vi "LifeEye_ver18_32bit.vi"() -> ()   [LabVIEW 2014]
uses:
  Keithley 2600 Series/sync_global.vi
  32bitDLLs/MADLib.dll
  LaserLineTunableFIlter/PHySpec-SDK-1.0.0/Labview-example/libPhyspec/libPhyspec.lvlib
panel:
  out "FilterWheelTemp":i32
  in  "Interline Delay (s)":dbl
  in  "2D Hyperspectral":bool
  out "Mono Calibration Handle":u32 caption="Calibration Handle"
  out "OMA V error":errorcluster
  in  "Tab Control 2":T1(tab)
  out "XY Graph OMA V":T2(graph)
  out "OMA V Hyperspectral graph":dbl[][](graph)
  out "OMA V PLE map graph":dbl[][](graph)
  out "OMA V PL external  sync plot":dbl[][](graph)
  out "timeend":i64
  out "timestart":i64
  out "Real Delay (seconds/step)":dbl
  out "Mono handle":u32
  in  "Grating Number":i16(ring) items=["", "Mirror", "300g/mm, blz=1.2um", "150g/mm, blz=1.2um"]
  in  "Filter Wheel Position":u16(ring) items=["", "Open", "320 nm", "590 nm", "715 nm", "655  nm", "Closed"]
  in  "Number of Spectra":i16=2 min=2 step=1
  out "Detector control":T3(tab)
  out "OMA V ready for sync":bool caption="ready"
  in  "OMA V correct background":bool
  in  "OMA V start background":bool
  in  "OMA V set temp":i8 caption="Set temp" min=-125 max=25 step=1
  in  "OMA V get temp":bool
  in  "OMA V start Focus":bool
  in  "OMA V Start Aquire":bool caption="Aquire"
  in  "OMA V gain":u32(ring) caption="Gain" items=["low", "high"]
  out "OMA V temp":dbl(slide) caption="Sensor Temperature" scale=-125.0..25.0
  in  "OMA V exposure time":dbl=0.001 caption="Integration time (s)" min=0.001 max=1000.0 step=0.001
  out "OMA  V ON":bool
  in  "Init OMA  V":bool
  in  "OMA V aquire mode":T4(radio) caption="Aquire mode"
  out "OMAV external sync":bool caption="sync"
  out "OMA V acquire from external":bool caption="acquire"
  out "OMA V Handles Out":T5
  out "OMA V Calibrated Array":dbl[](array[numeric]) caption="Calibrated Array" format="%.2f"
  out "Adjusted Values":T6 {"Pixel Width (microns)" format="%.2f"; "Magnification" format="%.2f"; "Detector Angle (degrees)" format="%.2f"; "Inclusion Angle (degrees)" format="%.2f"; "Focal Length (mm)" format="%.2f"; "Slope Adjust" format="%.2f"; "Center Offset" format="%.2f"}
  in  "Get param":bool
  in  "Init LockIn":bool
  out "LockIn ON":bool
  in  "Input Connection (0: Single-Ended Voltage)":u16(ring) items=["Single-Ended Voltage", "Differential Voltage", "1 MOhm Current Gain", "100 MOhm Current Gain"]
  in  "Input Coupling (0: AC)":u16(ring) items=["AC", "DC"]
  in  "Dynamic Reserve (2: Low Noise)":i8(ring)=2 items=["High Reserve"=0, "Normal"=1, "Low Noise"=2, "Auto Reserve"=-1]
  in  "Sensitivity (26: 1 V/uA)":i8(ring)=26 items=["Auto Gain"=-1, "2 nV/fA"=0, "5 nV/fA"=1, "10 nV/fA"=2, "20 nV/fA"=3, "50 nV/fA"=4, "100 nV/fA"=5, "200 nV/fA"=6, "500 nV/fA"=7, "1 uV/pA"=8, "2 uV/pA"=9, "5 uV/pA"=10, "10 uV/pA"=11, "20 uV/pA"=12, "50 uV/pA"=13, "100 uV/pA"=14, "200 uV/pA"=15, "500 uV/pA"=16, "1 mV/nA"=17, "2 mV/nA"=18, "5 mV/nA"=19, "10 mV/nA"=20, "20 mV/nA"=21, "50 mV/nA"=22, "100 mV/nA"=23, "200 mV/nA"=24, "500 mV/mA"=25, "1 V/uA"=26]
  in  "VISA resource name":refnum<visa-resource-name>
  out "LockIn Value":dbl
  in  "Histro start":bool
  in  "Histogramming Time (s)":dbl=0.001 min=0.001 max=360000.0 step=0.001
  in  "SaveHistro":bool
  in  "Init PicoHarp":bool
  out "PicoHarp ON":bool
  in  "Apply PicoHarp Settings":bool
  out "Error":bool
  out "Resolution":i32 min=0 max=2000 step=1
  out "SyncRate":i32 format="%#_7f"
  out "Ch1Rate":i32
  in  "Shutter:":bool
  in  "Bandpass (nm)":dbl min=0.0 max=30.0 step=0.1
  in  "ExcitationMap start":bool caption="OK Button"
  in  "PL Map Start":bool
  in  "Configuration File":path
  out "Current System":string
  out "LLTF error":errorcluster
  in  "PLE Start":bool
  out "LLTF handle":u32
  in  "Init LLTF":bool
  out "LLTF ON":bool
  in  "Wavelength LLTF (nm)":dbl=400.0 caption="Wavelength (nm)" min=400.0 max=1000.0 step=0.1
  in  "Tab Control":enum32{"Excitation", "Detection"}(tab)
  in  "Step delay LLTF":dbl caption="Step Delay (s)"
  in  "Steps LLTF":i32=1 caption="Steps" min=1 max=1000 step=1
  in  "End Wavelength LLTF":dbl=400.0 caption="End Wavelength (nm)" min=400.0 max=990.0 step=0.1
  in  "Start Wavelength LLTF":dbl=400.0 caption="Start Wavelength (nm)" min=400.0 max=1000.0 step=0.1
  in  "StepsDet":i32=1 caption="Steps" min=1 max=1000 step=1
  in  "Start Wavelength (nm)":dbl=400.0 min=400.0 max=2000.0 step=0.1
  in  "End Wavelength (nm)":dbl=400.0 min=400.0 max=2000.0 step=0.1
  in  "Step Delay (s)":dbl=0.1 min=0.001 max=360000.0 step=0.001
  in  "StepW (nm)":dbl=0.1 min=0.1 max=100.0 step=0.1
  in  "Forwardpix_scan":bool
  in  "Bidirectional scan":bool caption="Bidirectional"
  in  "PL_Clock":bool
  in  "SpectrMap start":bool
  in  "Stop Measurement":bool
  in  "ZScan start":bool
  out "MonoError":errorcluster
  out "PicoHarpInitError":bool
  out "PicoHarpHandle":i32
  out "Piezohandle":i32 caption="handle"
  in  "SaveIntMap":bool
  in  "SaveTRES":bool
  in  "SavePL":bool
  in  "IntMapping start":bool
  in  "StepZ (µm)":dbl=0.001 min=0.001 max=200.0 step=0.001
  in  "StepY (µm)":dbl=0.001 min=0.001 max=200.0 step=0.001
  in  "StepX (µm)":dbl=0.001 min=0.001 max=200.0 step=0.001
  in  "Pixel Delay (s)":dbl=0.1 min=0.001 max=360000.0 step=0.001
  in  "EndZ (µm)":dbl min=0.0 max=200.0 step=0.001
  in  "StartZ (µm)":dbl min=0.0 max=200.0 step=0.001
  in  "EndY (µm)":dbl min=0.0 max=200.0 step=0.001
  in  "StartY (µm)":dbl min=0.0 max=200.0 step=0.001
  in  "EndX (µm)":dbl min=0.0 max=200.0 step=0.001
  in  "StartX (µm)":dbl min=0.0 max=200.0 step=0.001
  in  "Stability check":bool
  in  "PL start":bool
  out "xRead":dbl format="%#.3g"
  out "yRead":dbl format="%#.3g"
  out "zRead":dbl format="%#.3g"
  in  "zCommand":dbl min=0.0 max=200.0 step=0.001
  in  "yCommand":dbl min=0.0 max=200.0 step=0.001
  in  "xCommand":dbl min=0.0 max=200.0 step=0.001
  in  "zGo":bool
  in  "yGo":bool
  in  "xGo":bool
  out "Busy":bool
  in  "Output Slit (µm)":i32=10 min=10 max=5000 step=1
  in  "Input Slit (µm)":i32=10 min=10 max=5000 step=1
  in  "Output Port":bool
  in  "Wavelength (nm)":dbl=400.0 min=-2000.0 max=2000.0 step=0.1
  out "PiezoStage ON":bool
  in  "Init Piezo":bool
  in  "Exit":bool
  out "Mono ON":bool
  in  "Init Mono":bool
  # "(only PLE Map)"
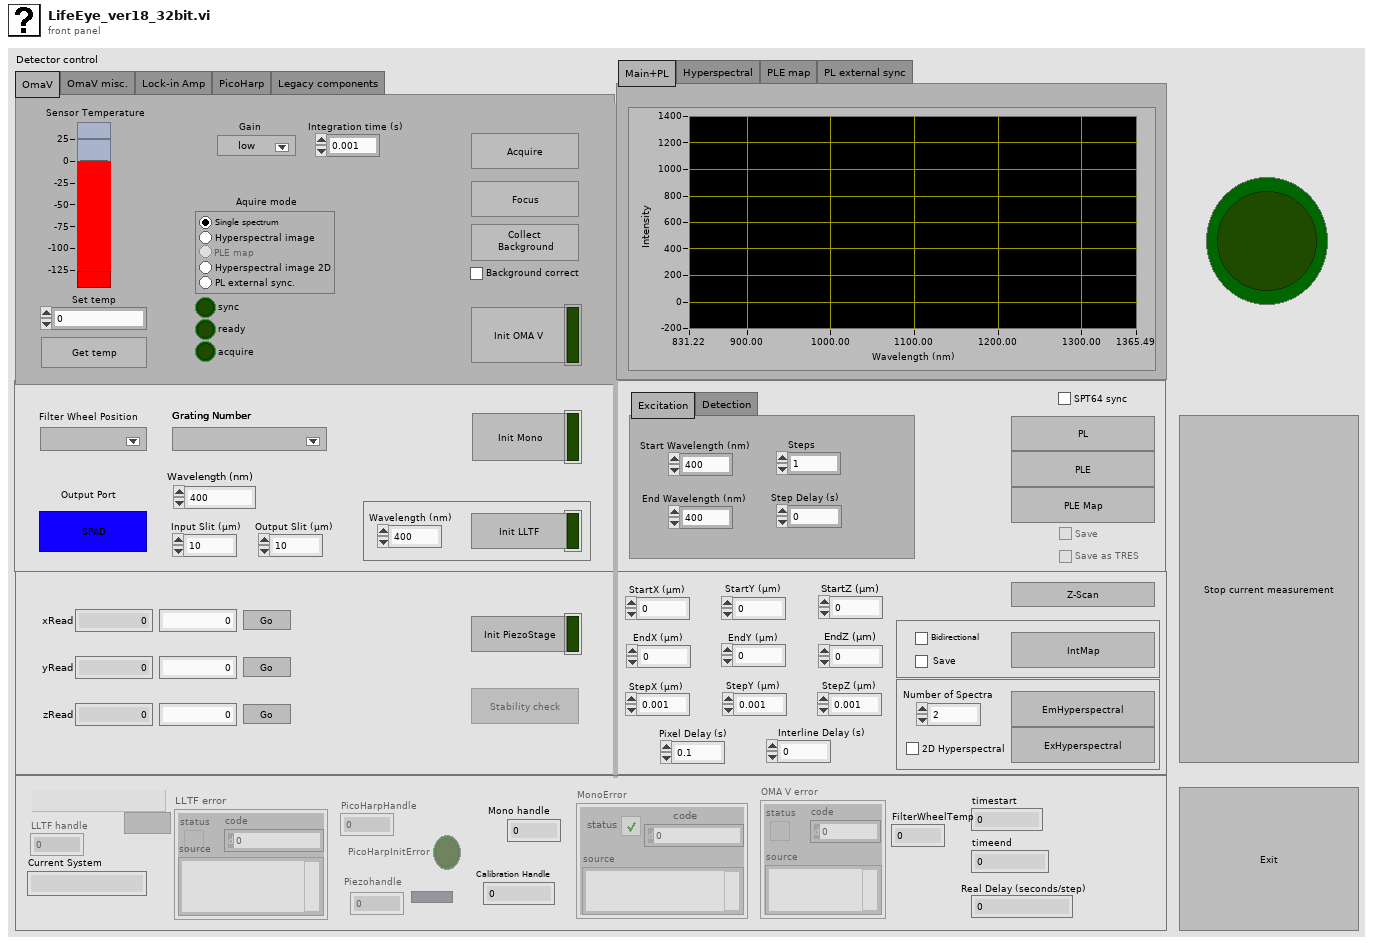
[diagram p1: front panel]
types:
  T1 = enum32{"Main+PL", "Hyperspectral", "PLE map", "PL external sync"}
  T2 = cluster{"Calibrated Array":dbl[], "Array F32":sgl[]}
  T3 = enum32{"OmaV", "OmaV misc.", "Lock-in Amp", "PicoHarp", "Legacy components"}
  T4 = enum32{"OMA V mode Single spectrum", "OMA V mode Hyperspectral", "OMA V mode PLE map", "OMA V mode Hyperspectral 2D", "OMA V mode PL external sync"}
  T5 = cluster{"Camera Handle":u32, "Pulser Handle":u32, "File Handle":u32, "Display Handle":u32, "Image Handle":u32}
  T6 = cluster{"Center Offset":dbl, "Slope Adjust":dbl, "Focal Length (mm)":dbl, "Inclusion Angle (degrees)":dbl, "Detector Angle (degrees)":dbl, "Magnification":dbl, "Pixel Width (microns)":dbl}
  T7 = enum8{"Enabled", "Disabled", "Disabled and Grayed Out"}
  T8 = cluster{"Acquire / focus mode \n1 is Sync circualar buffers":i32, "OMA V exposure time":dbl, "Number of Images":i32, "Number of software\naccumulations":i32}
  T9 = cluster{"Value From Calibration":dbl, "Value From Calibration":dbl, "Value From Calibration":dbl, "Value From Calibration":dbl, "Value From Calibration":dbl, "Value From Calibration":dbl, "Value From Calibration":dbl}
  T10 = cluster{"OMA V Calibrated Array":dbl[], "Array F32":sgl[]}
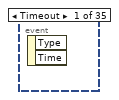
[diagram p2: hidden frame]
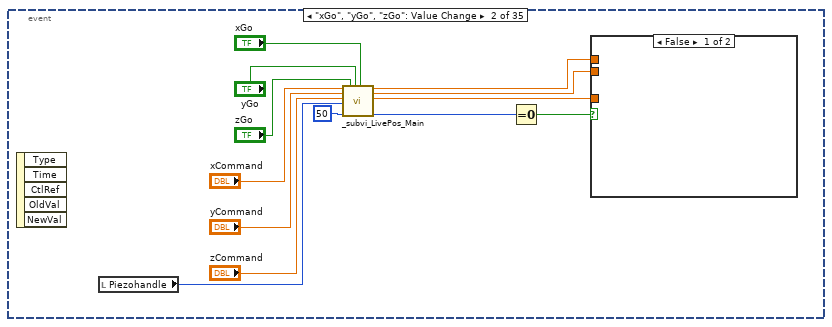
[diagram p3: hidden frame]
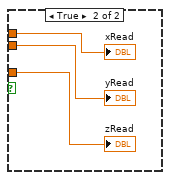
[diagram p4: hidden frame]
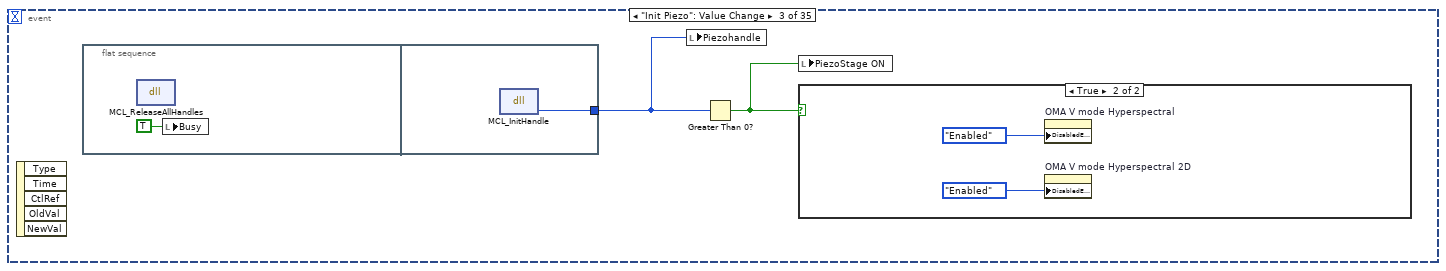
[diagram p5: hidden frame]
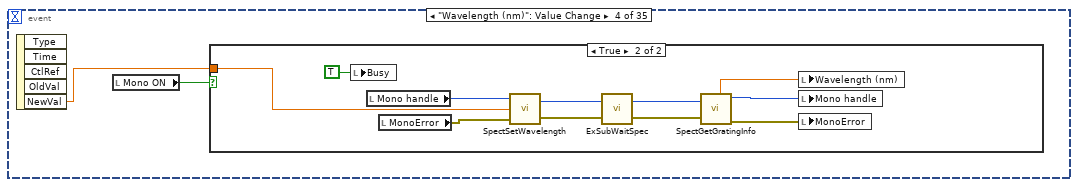
[diagram p7: hidden frame]
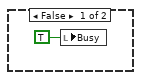
[diagram p8: hidden frame]
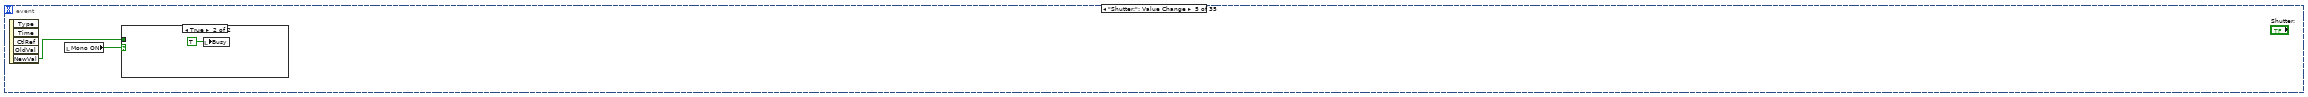
[diagram p9: hidden frame]
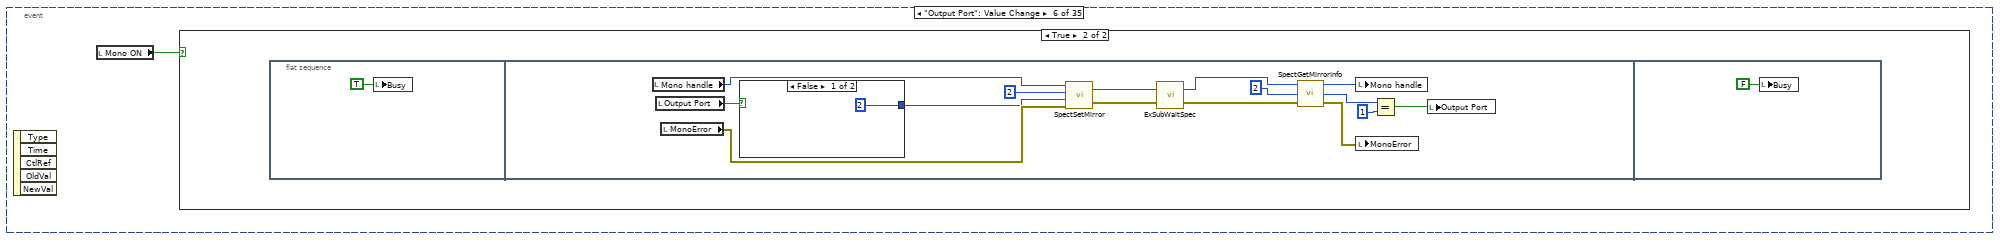
[diagram p11: hidden frame]
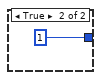
[diagram p13: hidden frame]
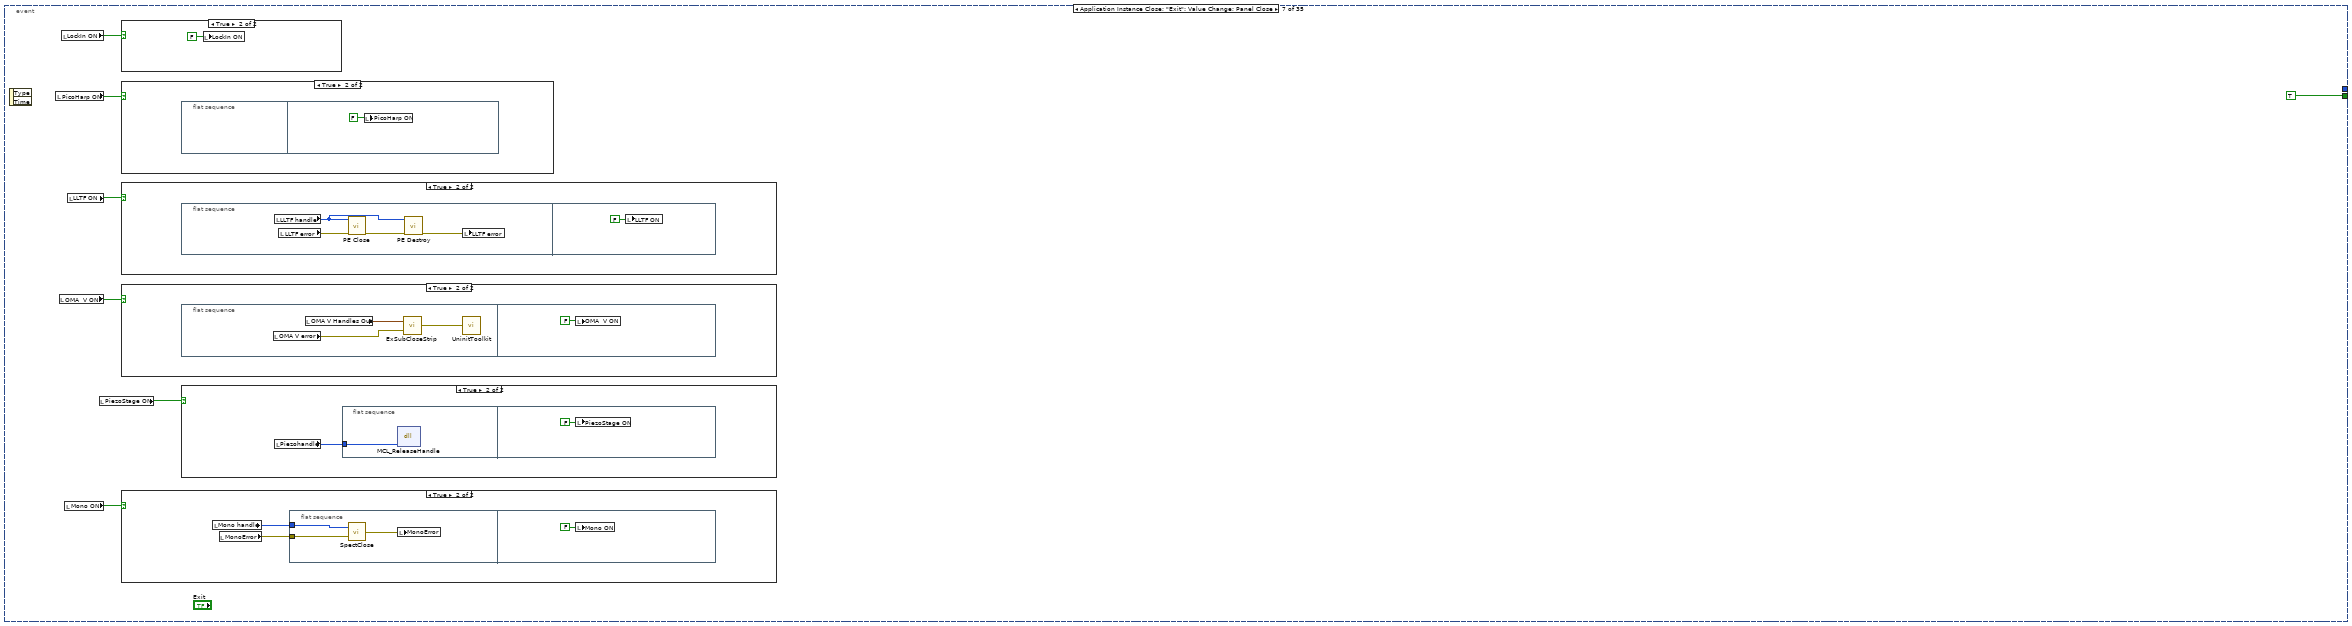
[diagram p14: hidden frame]
diagram:
  w4 = T7."Disabled and Grayed Out" ("Disabled")
  w14 = u16 1 items=["", "Mirror", "150g/mm, blz=1.2um", "300g/mm, blz=1.2um"] ("Grating Number")
  w15 = u16 1 items=["", "Open", "320 nm", "590 nm", "655 nm", "715  nm", "Closed"] ("Filter Wheel Position")
  w17 = FALSE
  w8 = FALSE
  # "PicoHarpResolution"
  # "PicoHarpSettingsError"
  # "PicoHarpInitError"
  # "PicoHarpHandle"
  # "MonoHandle"
  # "MonoError"
  # "PiezoHandle"
  # "error"
  n1 = while {
    stop <- w23 stop-if-true
    # "General seq."
    n2 = stacked-sequence {
      seq-local: [w26 _ _] -> [_ w461 _]
      seq-local: [w24 _ _] -> [_ w460 _]
      seq-local: [_ w461 _] -> [_ _ w2112]
      tunnel: [_ _ w2112] -> w23
      frame #0 {
        n3 = event shown="[19] \"Init LLTF\": Value Change" {
          selector: _ -> [_ _ _ _ _ _ _ _ _ _ _ _ _ _ _ _ _ _ _ _ _ _ _ _ _ _ _ _ _ _ _ _ _ _ _]
          dyn-events: _ -> [_ _ _ _ _ _ _ _ _ _ _ _ _ _ _ _ _ _ _ _ _ _ _ _ _ _ _ _ _ _ _ _ _ _ _]
          timeout: 1000 -> [_ _ _ _ _ _ _ _ _ _ _ _ _ _ _ _ _ _ _ _ _ _ _ _ _ _ _ _ _ _ _ _ _ _ _]
          tunnel: [_ _ _ _ _ _ TRUE _ _ _ _ _ _ _ _ _ _ _ _ _ _ _ _ _ _ _ _ _ _ _ _ _ _ _ _] -> w26
          tunnel: [_ _ _ _ _ _ _ _ _ _ _ _ _ w192 w195 w198 w201 w204 _ _ _ w247 w253 w257 _ _ _ w400 _ _ _ _ w438 w441 _] -> w24
          event Timeout {
            n4 = event-data() -> ()  [unwired: 1 in, 2 out]
          }
          event "xGo", "yGo", "zGo": Value Change {
            n5 = event-data() -> ()  [unwired: 1 in, 5 out]
            n6 = local read "Piezohandle"() -> (w27:i32)
            n7 = call "_subvi_LivePos_Main.vi"("xCommand"="xCommand", "yCommand"="yCommand", "zCommand"="zCommand", "handle"=w27, "counter"=u32 50, "commandZ"="zGo", "commandY"="yGo", "commandX"="xGo") -> ("xRead"=w39:dbl, "yRead"=w38:dbl, "zRead"=w37:dbl, "counter"=w32:u32)  [unwired: 8 out]
            n8 = Equal To 0?(x=w32) -> (x = 0?=w33:bool)
            n9 = case shown="False" w33 {
              tunnel: w39 -> [_ w42]
              tunnel: w38 -> [_ w41]
              tunnel: w37 -> [_ w40]
              frame False {
              }
              frame True {
                "xRead" <- w42
                "yRead" <- w41
                "zRead" <- w40
              }
            }
          }
          event "Init Piezo": Value Change {
            n10 = event-data() -> ()  [unwired: 1 in, 5 out]
            n11 = flat-sequence {
              tunnel: [w48] -> w44
              frame #0 {
                n12 = dll-call lib="C:/LabView_Projects/LifeEye/32bitDLLs/MADLib.dll" fn="MCL_ReleaseAllHandles" label="Release All Handles"() -> ()  [unwired: 3 in, 3 out]
                n13 = local write "Busy"(TRUE ("Busy")) -> ()
              }
              frame #1 {
                n14 = dll-call lib="C:/LabView_Projects/LifeEye/32bitDLLs/Madlib.dll" fn="MCL_InitHandle" label="Init Handle"() -> ("handle"=w48:i32)  [unwired: 3 in, 2 out]
              }
            }
            n15 = local write "Piezohandle"(w44) -> ()
            n16 = Greater Than 0?(x=w44) -> (x > 0?=w43:bool)
            n17 = local write "PiezoStage ON"(w43) -> ()
            n18 = case shown="True" w43 {
              frame False {
              }
              frame True {
                n19 = property on="OMA V mode Hyperspectral" class="Bool (strict)"("DisabledEnum"=T7."Enabled" ("Disabled")) -> ()  [unwired: 2 in, 2 out]
                n20 = property on="OMA V mode Hyperspectral 2D" class="Bool (strict)"("DisabledEnum"=T7."Enabled" ("Disabled")) -> ()  [unwired: 2 in, 2 out]
              }
            }
          }
          event "Wavelength (nm)": Value Change {
            n21 = event-data() -> ("NewVal"=w49:dbl)  [unwired: 1 in, 4 out]
            n22 = local read "Mono ON"() -> (w50:bool)
            n23 = case shown="True" w50 {
              tunnel: w49 -> [_ w59]
              frame False {
                n24 = local write "Busy"(TRUE ("Busy")) -> ()
              }
              frame True {
                n25 = local write "Busy"(TRUE ("Busy")) -> ()
                n26 = local read "Mono handle"() -> (w61:u32)
                n27 = local read "MonoError"() -> (w60:errorcluster)
                n28 = call "SpectSetWavelength.vi"("error in"=w60, "Wavelength"=w59, "Spectrometer Handle"=w61) -> ("error out"=w57:errorcluster, "Spectrumeter Handle"=w58:u32)
                n29 = call "ExSubWaitSpec.vi"("error in (no error)"=w57, "Spectrometer Handle"=w58) -> ("error out"=w55:errorcluster, "Spectrometer handle"=w56:u32)
                n30 = call "SpectGetGratingInfo.vi"("Spectrometer Handle"=w56, "error in"=w55) -> ("Current Wavelength"=w54:dbl, "Spectrometer Handle"=w52:u32, "error out"=w53:errorcluster)  [unwired: 3 out]
                n31 = local write "Wavelength (nm)"(w54) -> ()
                n32 = local write "Mono handle"(w52) -> ()
                n33 = local write "MonoError"(w53) -> ()
              }
            }
          }
          event "Shutter:": Value Change {
            n34 = event-data() -> ("NewVal"=w64:bool)  [unwired: 1 in, 4 out]
            n35 = local read "Mono ON"() -> (w63:bool)
            n36 = case shown="True" w63 {
              tunnel: w64 -> [_ _]
              frame False {
              }
              frame True {
                n37 = local write "Busy"(TRUE ("Busy")) -> ()
              }
            }
          }
          event "Output Port": Value Change {
            n38 = event-data() -> ()  [unwired: 1 in, 5 out]
            n39 = local read "Mono ON"() -> (w66:bool)
            n40 = case shown="True" w66 {
              frame False {
              }
              frame True {
                n41 = flat-sequence {
                  frame #0 {
                    n42 = local write "Busy"(TRUE ("Busy")) -> ()
                  }
                  frame #1 {
                    n43 = local read "Mono handle"() -> (w77:u32)
                    n44 = local read "Output Port"() -> (w69:bool)
                    n45 = local read "MonoError"() -> (w78:errorcluster)
                    n46 = case shown="False" w69 {
                      tunnel: [2 1] -> w75
                      frame False {
                      }
                      frame True {
                      }
                    }
                    n47 = call "SpectSetMirror.vi"("error in"=w78, "Position"=w75, "Mirror"=i16 2, "Spectrometer Handle"=w77) -> ("error out"=w80:errorcluster, "Spectrometer Handle"=w79:u32)
                    n48 = call "ExSubWaitSpec.vi"("error in (no error)"=w80, "Spectrometer Handle"=w79) -> ("error out"=w82:errorcluster, "Spectrometer handle"=w81:u32)
                    n49 = call "SpectGetMirrorInfo.vi"("error in"=w82, "Mirror"=i16 2, "Spectrometer Handle"=w81) -> ("error out"=w73:errorcluster, "Position"=w72:i16, "Spectrometer Handle"=w74:u32)
                    n50 = local write "Mono handle"(w74) -> ()
                    n51 = local write "MonoError"(w73) -> ()
                    n52 = Equal?(x=w72, y=i16 1) -> (x = y?=w70:bool)
                    n53 = local write "Output Port"(w70) -> ()
                  }
                  frame #2 {
                    n54 = local write "Busy"(FALSE ("Busy")) -> ()
                  }
                }
              }
            }
          }
          event Application Instance Close; "Exit": Value Change; Panel Close {
            n55 = event-data() -> ()  [unwired: 1 in, 2 out]
            n56 = local read "PicoHarp ON"() -> (w91:bool)
            n57 = local read "OMA  V ON"() -> (w86:bool)
            n58 = local read "LockIn ON"() -> (w88:bool)
            n59 = local read "Mono ON"() -> (w90:bool)
            n60 = local read "LLTF ON"() -> (w87:bool)
            n61 = local read "PiezoStage ON"() -> (w89:bool)
            n62 = case shown="True" w88 {
              frame False {
              }
              frame True {
                n63 = local write "LockIn ON"(FALSE ("LockIn ON")) -> ()
              }
            }
            n64 = case shown="True" w91 {
              frame False {
              }
              frame True {
                n65 = flat-sequence {
                  frame #0 {
                  }
                  frame #1 {
                    n66 = local write "PicoHarp ON"(FALSE ("PicoHarp ON")) -> ()
                  }
                }
              }
            }
            n67 = case shown="True" w87 {
              frame False {
              }
              frame True {
                n68 = flat-sequence {
                  frame #0 {
                    n69 = local read "LLTF handle"() -> (w97:u32)
                    n70 = local read "LLTF error"() -> (w99:errorcluster)
                    n71 = call "PE Close.vi"("error in (no error)"=w99, "peHandle"=w97) -> ("error out"=w100:errorcluster)  [unwired: 8 in, 1 out]
                    n72 = call "PE Destroy.vi"("error in (no error)"=w100, "peHandle"=w97) -> ("error out"=w98:errorcluster)  [unwired: 8 in, 1 out]
                    n73 = local write "LLTF error"(w98) -> ()
                  }
                  frame #1 {
                    n74 = local write "LLTF ON"(FALSE ("LLTF ON")) -> ()
                  }
                }
              }
            }
            n75 = case shown="True" w86 {
              frame False {
              }
              frame True {
                n76 = flat-sequence {
                  frame #0 {
                    n77 = local read "OMA V error"() -> (w94:errorcluster)
                    n78 = local read "OMA V Handles Out"() -> (w95:T5)
                    n79 = call "ExSubCloseStrip.vi"("error in (no error)"=w94, "Handles In"=w95) -> ("error out"=w93:errorcluster)
                    n80 = call "UninitToolkit.vi"("error in"=w93) -> ()  [unwired: 1 out]
                  }
                  frame #1 {
                    n81 = local write "OMA  V ON"(FALSE ("OMA  V ON")) -> ()
                  }
                }
              }
            }
            n82 = case shown="True" w90 {
              frame False {
              }
              frame True {
                n83 = local read "Mono handle"() -> (w107:u32)
                n84 = local read "MonoError"() -> (w106:errorcluster)
                n85 = flat-sequence {
                  tunnel: w107 -> [w109]
                  tunnel: w106 -> [w108]
                  frame #0 {
                    n86 = call "SpectClose.vi"("error in"=w108, "Spectrometer Handle"=w109) -> ("error out"=w110:errorcluster)
                    n87 = local write "MonoError"(w110) -> ()
                  }
                  frame #1 {
                    n88 = local write "Mono ON"(FALSE ("Mono ON")) -> ()
                  }
                }
              }
            }
            n89 = case shown="True" w89 {
              frame False {
              }
              frame True {
                n90 = local read "Piezohandle"() -> (w103:i32)
                n91 = flat-sequence {
                  tunnel: w103 -> [w104]
                  frame #0 {
                    n92 = dll-call lib="C:/LabView_Projects/LifeEye/32bitDLLs/MADLib.dll" fn="MCL_ReleaseHandle" label="Release Handle"("handle"=w104) -> ()  [unwired: 4 in, 3 out]
                  }
                  frame #1 {
                    n93 = local write "PiezoStage ON"(FALSE ("PiezoStage ON")) -> ()
                  }
                }
              }
            }
          }
          event "Input Slit (µm)", "Output Slit (µm)": Value Change {
            n94 = event-data() -> ("OldVal"=w113:i32, "NewVal"=w114:i32)  [unwired: 1 in, 3 out]
            n95 = local read "Mono ON"() -> (w115:bool)
            n96 = case shown="True" w115 {
              tunnel: w114 -> [_ _]
              tunnel: w113 -> [_ _]
              frame False {
              }
              frame True {
                n97 = flat-sequence {
                  frame #0 {
                    n98 = local write "Busy"(TRUE ("Busy")) -> ()
                  }
                  frame #1 {
                    n99 = local read "Mono handle"() -> (w138:u32)
                    n100 = local read "MonoError"() -> (w137:errorcluster)
                    n101 = local read "Output Slit (µm)"() -> (w131:i32)
                    n102 = local read "Input Slit (µm)"() -> (w132:i32)
                    n103 = call "SpectSetSlit.vi"("Spectrometer Handle"=w138, "Slit Number"=i16 2, "Position"=w132, "error in"=w137) -> ("Spectrometer Handle"=w135:u32, "error out"=w134:errorcluster)  [unwired: 1 in]
                    n104 = call "ExSubWaitSpec.vi"("error in (no error)"=w134, "Spectrometer Handle"=w135) -> ("error out"=w130:errorcluster, "Spectrometer handle"=w129:u32)
                    n105 = call "SpectSetSlit.vi"("Spectrometer Handle"=w129, "Slit Number"=i16 4, "Position"=w131, "error in"=w130) -> ("Spectrometer Handle"=w127:u32, "error out"=w128:errorcluster)  [unwired: 1 in]
                    n106 = call "ExSubWaitSpec.vi"("error in (no error)"=w128, "Spectrometer Handle"=w127) -> ("error out"=w125:errorcluster, "Spectrometer handle"=w126:u32)
                    n107 = call "SpectGetSlitInfo.vi"("Spectrometer Handle"=w126, "Slit"=i16 2, "error in"=w125) -> ("Spectrometer Handle"=w123:u32, "Position"=w120:dbl, "error out"=w122:errorcluster)  [unwired: 1 out]
                    n108 = local write "Input Slit (µm)"(w120) -> ()
                    n109 = call "SpectGetSlitInfo.vi"("Spectrometer Handle"=w123, "Slit"=i16 4, "error in"=w122) -> ("Spectrometer Handle"=w118:u32, "Position"=w119:dbl, "error out"=w117:errorcluster)  [unwired: 1 out]
                    n110 = local write "Mono handle"(w118) -> ()
                    n111 = local write "Output Slit (µm)"(w119) -> ()
                    n112 = local write "MonoError"(w117) -> ()
                  }
                }
              }
            }
          }
          event "Bandpass (nm)": Value Change {
            n113 = event-data() -> ()  [unwired: 1 in, 5 out]
          }
          event "Init PicoHarp": Value Change {
            n114 = event-data() -> ()  [unwired: 1 in, 5 out]
          }
          event "Init Mono": Value Change {
            n115 = event-data() -> ()  [unwired: 1 in, 5 out]
            n116 = local read "Mono ON"() -> (w140:bool)
            n117 = Not(x=w140) -> (.not. x?=w139:bool)
            n118 = case shown="True" w139 {
              frame False {
                n119 = local write "Busy"(TRUE ("Busy")) -> ()
              }
              frame True {
                n120 = flat-sequence {
                  tunnel: [w151] -> w143
                  tunnel: [w150] -> w142
                  tunnel: w143 -> [w189]
                  tunnel: w142 -> [w190]
                  frame #0 {
                    n121 = local write "Busy"(TRUE ("Busy")) -> ()
                  }
                  frame #1 {
                    n122 = call "InitToolkit.vi"() -> ("error out"=w155:errorcluster)  [unwired: 1 in]
                    n123 = call "SpectOpen.vi"("error in"=w155, "Spectrometer ID"=u32 0) -> ("error out"=w167:errorcluster, "Spectrometer Handle"=w168:u32)  [unwired: 1 in]
                    n124 = local read "Filter Wheel Position"() -> (w174:u16)
                    n125 = call "SpectSetup.vi"("error in"=w167, "Spectrometer Handle"=w168) -> ("error out"=w165:errorcluster, "Spectrometer Handle"=w166:u32)
                    n126 = call "SpectSetGrating.vi"("error in"=w165, "Grating Number"=i16 1, "Sepctrometer Handle"=w166) -> ("error out"=w163:errorcluster, "Spectrometer Handle"=w164:u32)
                    n127 = call "ExSubWaitSpec.vi"("error in (no error)"=w163, "Spectrometer Handle"=w164) -> ("error out"=w161:errorcluster, "Spectrometer handle"=w162:u32)
                    n128 = call "SpectSetGratingSpeed.vi"("error in"=w161, "Grating Speed"=2000.0, "Spectrometer Handle"=w162) -> ("error out"=w159:errorcluster, "Spectrometer Handle"=w160:u32)
                    n129 = call "ExSubWaitSpec.vi"("error in (no error)"=w159, "Spectrometer Handle"=w160) -> ("error out"=w146:errorcluster, "Spectrometer handle"=w145:u32)
                    n130 = call "SpectSetWavelength.vi"("error in"=w146, "Wavelength"=0.0, "Spectrometer Handle"=w145) -> ("error out"=w186:errorcluster, "Spectrumeter Handle"=w185:u32)
                    n131 = call "ExSubWaitSpec.vi"("error in (no error)"=w186, "Spectrometer Handle"=w185) -> ("error out"=w181:errorcluster, "Spectrometer handle"=w184:u32)
                    n132 = call "SpectGetGratingInfo.vi"("Spectrometer Handle"=w184, "error in"=w181) -> ("Current Wavelength"=w178:dbl, "Spectrometer Handle"=w183:u32, "Current Grating"=w177:i16, "error out"=w180:errorcluster)  [unwired: 2 out]
                    n133 = local write "Wavelength (nm)"(w178) -> ()
                    n134 = local write "Grating Number"(w177) -> ()
                    n135 = call "SpectSetFilter.vi"("Filter Number"=w174, "error in"=w180, "Filter Wheel Number"=i16 1, "Spectrometer Handle"=w183) -> ("error out"=w179:errorcluster, "Spectrometer Handle"=w182:u32)
                    n136 = call "SpectGetSlitInfo.vi"("Spectrometer Handle"=w182, "Slit"=i16 2, "error in"=w179) -> ("Spectrometer Handle"=w172:u32, "Position"=w173:dbl, "error out"=w171:errorcluster)  [unwired: 1 out]
                    n137 = local write "Input Slit (µm)"(w173) -> ()
                    n138 = call "SpectGetSlitInfo.vi"("Spectrometer Handle"=w172, "Slit"=i16 4, "error in"=w171) -> ("Spectrometer Handle"=w153:u32, "Position"=w169:dbl, "error out"=w152:errorcluster)  [unwired: 1 out]
                    n139 = local write "Output Slit (µm)"(w169) -> ()
                    n140 = call "SpectGetMirrorInfo.vi"("error in"=w152, "Mirror"=i16 2, "Spectrometer Handle"=w153) -> ("error out"=w150:errorcluster, "Position"=w149:i16, "Spectrometer Handle"=w151:u32)
                    n141 = Equal?(x=w149, y=i16 1) -> (x = y?=w147:bool)
                    n142 = local write "Output Port"(w147) -> ()
                  }
                  frame #2 {
                    n143 = local write "Mono handle"(w189) -> ()
                    n144 = local write "MonoError"(w190) -> ()
                    n145 = local write "Mono ON"(TRUE) -> ()
                    n146 = local write "Busy"(FALSE ("Busy")) -> ()
                  }
                }
              }
            }
          }
          event "Apply PicoHarp Settings": Value Change {
            n147 = event-data() -> ()  [unwired: 1 in, 5 out]
          }
          event "Stability check": Value Change {
            n148 = event-data() -> ()  [unwired: 1 in, 5 out]
          }
          event "Histro start": Value Change {
            n149 = event-data() -> ()  [unwired: 1 in, 5 out]
            n150 = local read "PicoHarp ON"() -> (w193:bool)
            n151 = case shown="True" w193 {
              tunnel: [_ 13] -> w192
              frame False {
              }
              frame True {
              }
            }
          }
          event "PL start": Value Change {
            n152 = event-data() -> ()  [unwired: 1 in, 5 out]
            n153 = local read "Mono ON"() -> (w196:bool)
            n154 = case shown="True" w196 {
              tunnel: [_ 14] -> w195
              frame False {
              }
              frame True {
              }
            }
          }
          event "ZScan start": Value Change {
            n155 = event-data() -> ()  [unwired: 1 in, 5 out]
            n156 = local read "PiezoStage ON"() -> (w199:bool)
            n157 = case shown="True" w199 {
              tunnel: [_ 15] -> w198
              frame False {
              }
              frame True {
              }
            }
          }
          event "IntMapping start": Value Change {
            n158 = event-data() -> ()  [unwired: 1 in, 5 out]
            n159 = local read "PiezoStage ON"() -> (w202:bool)
            n160 = case shown="True" w202 {
              tunnel: [_ 16] -> w201
              frame False {
              }
              frame True {
              }
            }
          }
          event "SpectrMap start": Value Change {
            n161 = event-data() -> ()  [unwired: 1 in, 5 out]
            n162 = local read "PiezoStage ON"() -> (w207:bool)
            n163 = local read "Mono ON"() -> (w206:bool)
            n164 = And(x=w207, y=w206) -> (x .and. y?=w205:bool)
            n165 = case shown="True" w205 {
              tunnel: [_ 17] -> w204
              frame False {
              }
              frame True {
              }
            }
          }
          event "Init LockIn": Value Change {
            n166 = event-data() -> ()  [unwired: 1 in, 5 out]
            n167 = local read "LockIn ON"() -> (w210:bool)
            n168 = Not(x=w210) -> (.not. x?=w209:bool)
            n169 = case shown="True" w209 {
              frame False {
              }
              frame True {
                (unwired) FALSE  # Enable Sync Filter (F: Disable)
                (unwired) u16 1 items=["6 dB/oct", "12 dB/oct", "18 db/oct", "24 dB/oct"]  # Low Pass Filter Slope (1: 12dB/oct)
                (unwired) u16 9 items=["10 us", "30 us", "100 us", "300 us", "1 ms", "3 ms", "10 ms", "30 ms", "100 ms", "300 ms", "1 s", "3 s", "10 s", "30 s", "100 s", "300 s", "1 ks", "3 ks", "10 ks", "30 ks"]  # Time Constant (8: 100ms)
                (unwired) FALSE  # Auto Phase (T: Enabled)
                (unwired) u16 0 items=["None", "Line Notch", "2x Line Notch", "Both Notch Filters"]  # Input Notch Filter (0: None)
                (unwired) u16 0 items=["Float", "Ground"]  # Input Shield Grounding (0: Float)
                (unwired) u16 0 items=["External", "Internal"]  # Reference Source (1: Internal)
                n170 = local write "LockIn ON"(TRUE ("LockIn ON")) -> ()
              }
            }
          }
          event "Init LLTF": Value Change {
            n171 = event-data() -> ()  [unwired: 1 in, 5 out]
            n172 = local read "LLTF ON"() -> (w213:bool)
            n173 = Not(x=w213) -> (.not. x?=w212:bool)
            n174 = case shown="True" w212 {
              frame False {
                n175 = local write "Busy"(TRUE ("Busy")) -> ()
              }
              frame True {
                n176 = flat-sequence {
                  tunnel: [w223] -> w216
                  tunnel: [w222] -> w215
                  tunnel: w216 -> [w236]
                  tunnel: w215 -> [w235]
                  frame #0 {
                    n177 = local write "Busy"(TRUE ("Busy")) -> ()
                  }
                  frame #1 {
                    n178 = local read "Configuration File"() -> (w218:path)
                    n179 = Path To String(path=w218) -> (string=w233:string)
                    n180 = call "PE Create.vi"("conffile"=w233) -> ("error out"=w230:errorcluster, "peHandle"=w222:u32)  [unwired: 8 in, 1 out]
                    n181 = call "PE Get System Name.vi"("error in (no error)"=w230, "size"=4095, "index"=0, "peHandle"=w222) -> ("error out"=w228:errorcluster, "name"=w229:string)  [unwired: 5 in, 1 out]
                    "Current System" <- w229
                    n182 = call "PE Open.vi"("error in (no error)"=w228, "name"=w229, "peHandle"=w222) -> ("error out"=w227:errorcluster)  [unwired: 7 in, 1 out]
                    n183 = call "PE Get Wavelength Range.vi"("error in (no error)"=w227, "peHandle"=w222) -> ("error out"=w225:errorcluster, "maximum"=w221:dbl, "minimum"=w226:dbl)  [unwired: 6 in, 1 out]
                    n184 = local write "Start Wavelength LLTF"(w226) -> ()
                    n185 = call "PE Get Wavelength.vi"("error in (no error)"=w225, "peHandle"=w222) -> ("error out"=w223:errorcluster, "wavelength"=w224:dbl)  [unwired: 7 in, 1 out]
                    n186 = Subtract(x=w221, y=5.0) -> (x-y=w220:dbl)
                    n187 = local write "End Wavelength LLTF"(w220) -> ()
                    n188 = local write "Wavelength LLTF (nm)"(w224) -> ()
                  }
                  frame #2 {
                    n189 = local write "LLTF handle"(w235) -> ()
                    n190 = local write "LLTF error"(w236) -> ()
                    n191 = local write "LLTF ON"(TRUE) -> ()
                    n192 = property on="OMA V mode PLE map" class="Bool (strict)"("DisabledEnum"=T7."Enabled" ("Disabled")) -> ()  [unwired: 2 in, 2 out]
                  }
                }
              }
            }
          }
          event "Wavelength LLTF (nm)": Value Change {
            n193 = event-data() -> ("NewVal"=w238:dbl)  [unwired: 1 in, 4 out]
            n194 = local read "LLTF ON"() -> (w239:bool)
            n195 = case shown="True" w239 {
              tunnel: w238 -> [_ w246]
              frame False {
              }
              frame True {
                n196 = local write "Busy"(TRUE ("Busy")) -> ()
                n197 = local read "LLTF handle"() -> (w243:u32)
                n198 = local read "LLTF error"() -> (w245:errorcluster)
                n199 = call "PE Set Wavelength.vi"("error in (no error)"=w245, "wavelength"=w246, "peHandle"=w243) -> ("error out"=w244:errorcluster)  [unwired: 7 in, 1 out]
                n200 = call "PE Get Wavelength.vi"("error in (no error)"=w244, "peHandle"=w243) -> ("error out"=w241:errorcluster, "wavelength"=w242:dbl)  [unwired: 7 in, 1 out]
                n201 = local write "Wavelength LLTF (nm)"(w242) -> ()
                n202 = local write "LLTF error"(w241) -> ()
              }
            }
          }
          event "PLE Start": Value Change {
            n203 = event-data() -> ()  [unwired: 1 in, 5 out]
            n204 = local read "LLTF ON"() -> (w248:bool)
            n205 = case shown="True" w248 {
              tunnel: [_ 21] -> w247
              frame False {
              }
              frame True {
              }
            }
          }
          event "PL Map Start": Value Change {
            n206 = event-data() -> ()  [unwired: 1 in, 5 out]
            n207 = local read "Mono ON"() -> (w251:bool)
            n208 = local read "LLTF ON"() -> (w250:bool)
            n209 = And(x=w251, y=w250) -> (x .and. y?=w252:bool)
            n210 = case shown="True" w252 {
              tunnel: [_ 22] -> w253
              frame False {
              }
              frame True {
              }
            }
          }
          event "ExcitationMap start": Value Change {
            n211 = event-data() -> ()  [unwired: 1 in, 5 out]
            n212 = local read "PiezoStage ON"() -> (w255:bool)
            n213 = local read "LLTF ON"() -> (w256:bool)
            n214 = And(x=w256, y=w255) -> (x .and. y?=w258:bool)
            n215 = case shown="True" w258 {
              tunnel: [_ 23] -> w257
              frame False {
              }
              frame True {
              }
            }
          }
          event "Filter Wheel Position": Value Change {
            n216 = event-data() -> ("NewVal"=w262:u16)  [unwired: 1 in, 5 out]
            n217 = local read "Mono ON"() -> (w263:bool)
            n218 = flat-sequence {
              tunnel: w262 -> [w265]
              tunnel: w263 -> [w266]
              tunnel: [w266] -> w261
              tunnel: [w265] -> w260
              tunnel: w261 -> [w268]
              tunnel: w260 -> [w267]
              frame #0 {
                n219 = local write "Busy"(TRUE ("Busy")) -> ()
              }
              frame #1 {
                n220 = case shown="True" w268 {
                  tunnel: w267 -> [_ w279]
                  frame False {
                  }
                  frame True {
                    n221 = local read "Mono handle"() -> (w276:u32)
                    n222 = local read "MonoError"() -> (w275:errorcluster)
                    n223 = call "SpectSetFilter.vi"("Filter Number"=w279, "error in"=w275, "Filter Wheel Number"=i16 1, "Spectrometer Handle"=w276) -> ("error out"=w277:errorcluster, "Spectrometer Handle"=w278:u32)
                    n224 = call "ExSubWaitSpec.vi"("error in (no error)"=w277, "Spectrometer Handle"=w278) -> ("error out"=w272:errorcluster, "Spectrometer handle"=w273:u32)
                    n225 = call "SpectGetFilter.vi"("error in"=w272, "Filter Wheel Number"=i16 1, "Spectrometer Handle"=w273) -> ("error out"=w270:errorcluster, "Filter Number"=w269:i16, "Spectrometer Handle"=w271:u32)
                    n226 = local write "Mono handle"(w271) -> ()
                    n227 = local write "Filter Wheel Position"(w269) -> ()
                    n228 = local write "MonoError"(w270) -> ()
                  }
                }
              }
              frame #2 {
                n229 = local write "Busy"(FALSE ("Busy")) -> ()
              }
            }
          }
          event "Grating Number": Value Change {
            n230 = event-data() -> ("NewVal"=w284:i16)  [unwired: 1 in, 5 out]
            n231 = local read "Mono ON"() -> (w285:bool)
            n232 = flat-sequence {
              tunnel: w284 -> [w287]
              tunnel: w285 -> [w288]
              tunnel: [w288] -> w283
              tunnel: [w287] -> w282
              tunnel: w283 -> [w290]
              tunnel: w282 -> [w289]
              frame #0 {
                n233 = local write "Busy"(TRUE ("Busy")) -> ()
              }
              frame #1 {
                n234 = case shown="True" w290 {
                  tunnel: w289 -> [_ w292]
                  frame False {
                  }
                  frame True {
                    n235 = local read "Mono handle"() -> (w298:u32)
                    n236 = local read "MonoError"() -> (w297:errorcluster)
                    n237 = local read "Wavelength (nm)"() -> (w291:dbl)
                    n238 = call "SpectSetGrating.vi"("error in"=w297, "Grating Number"=w292, "Sepctrometer Handle"=w298) -> ("error out"=w304:errorcluster, "Spectrometer Handle"=w303:u32)
                    n239 = call "ExSubWaitSpec.vi"("error in (no error)"=w304, "Spectrometer Handle"=w303) -> ("error out"=w306:errorcluster, "Spectrometer handle"=w305:u32)
                    n240 = call "SpectSetGratingSpeed.vi"("error in"=w306, "Grating Speed"=2000.0, "Spectrometer Handle"=w305) -> ("error out"=w308:errorcluster, "Spectrometer Handle"=w307:u32)
                    n241 = call "ExSubWaitSpec.vi"("error in (no error)"=w308, "Spectrometer Handle"=w307) -> ("error out"=w310:errorcluster, "Spectrometer handle"=w309:u32)
                    n242 = call "SpectSetWavelength.vi"("error in"=w310, "Wavelength"=w291, "Spectrometer Handle"=w309) -> ("error out"=w299:errorcluster, "Spectrumeter Handle"=w300:u32)
                    n243 = call "ExSubWaitSpec.vi"("error in (no error)"=w299, "Spectrometer Handle"=w300) -> ("error out"=w302:errorcluster, "Spectrometer handle"=w301:u32)
                    n244 = call "SpectGetGratingInfo.vi"("Spectrometer Handle"=w301, "error in"=w302) -> ("Current Wavelength"=w295:dbl, "Spectrometer Handle"=w296:u32, "Current Grating"=w294:i16, "error out"=w293:errorcluster)  [unwired: 2 out]
                    n245 = local write "Wavelength (nm)"(w295) -> ()
                    n246 = local write "Mono handle"(w296) -> ()
                    n247 = local write "Grating Number"(w294) -> ()
                    n248 = local write "MonoError"(w293) -> ()
                  }
                }
              }
              frame #2 {
                n249 = local write "Busy"(FALSE ("Busy")) -> ()
              }
            }
          }
          event "Init OMA  V": Value Change {
            n250 = event-data() -> ()  [unwired: 1 in, 6 out]
            n251 = local read "OMA  V ON"() -> (w313:bool)
            n252 = local read "Mono ON"() -> (w316:bool)
            n253 = Not(x=w313) -> (.not. x?=w315:bool)
            n254 = And(x=w315, y=w316) -> (x .and. y?=w314:bool)
            n255 = case shown="True" w314 {
              frame False {
              }
              frame True {
                n256 = flat-sequence {
                  frame #0 {
                    n257 = local write "Busy"(TRUE ("Busy")) -> ()
                    n258 = Wait (ms)(milliseconds to wait=u32 500) -> ()  [unwired: 1 out]
                  }
                  frame #1 {
                    w329 = u32 1 ("Turret Number")
                    w360 = 2  # Edge Trigger, 2 is negative
                    w361 = 1  # Timing Mode, 1 is freerun/timed mode
                    w365 = 0  # Pulser Handle
                    w368 = 1  # Number of Images
                    w369 = 1  # Acquire / focus mode  1 is Sync circualar buffers
                    w367 = 1  # Number of software accumulations
                    w372 = u32 0  # Camera Device ID
                    n259 = local read "Mono handle"() -> (w339:u32)
                    n260 = local read "MonoError"() -> (w338:errorcluster)
                    n261 = local read "OMA V exposure time"() -> (w348:dbl)
                    n262 = local read "Wavelength (nm)"() -> (w328:dbl)
                    n263 = local read "Grating Number"() -> (w322:i16)
                    n264 = case shown="3" w322 {
                      tunnel: [w375 w383 w391] -> w319
                      frame 1, Default {
                        w376 = 25.0  # Pixel Width (microns)
                        w377 = 1.0  # Magnification
                        w378 = 1.35  # Detector Angle (degrees)
                        w379 = 30.3  # Inclusion Angle (degrees)
                        w380 = 300.0  # Focal Length (mm)
                        w381 = 0.0  # Slope Adjust
                        w382 = -3.71785  # Center Offset
                        n265 = Bundle("Center Offset"=w382, "Slope Adjust"=w381, "Focal Length (mm)"=w380, "Inclusion Angle (degrees)"=w379, "Detector Angle (degrees)"=w378, "Magnification"=w377, "Pixel Width (microns)"=w376) -> (w375:T6)  [unwired: 1 in]
                      }
                      frame 2 {
                        w384 = 25.0  # Pixel Width (microns)
                        w385 = 1.0  # Magnification
                        w386 = -2.77  # Detector Angle (degrees)
                        w387 = 32.7  # Inclusion Angle (degrees)
                        w388 = 295.6  # Focal Length (mm)
                        w389 = -0.000221379  # Slope Adjust
                        w390 = -0.047502  # Center Offset
                        n266 = Bundle("Center Offset"=w390, "Slope Adjust"=w389, "Focal Length (mm)"=w388, "Inclusion Angle (degrees)"=w387, "Detector Angle (degrees)"=w386, "Magnification"=w385, "Pixel Width (microns)"=w384) -> (w383:T6)  [unwired: 1 in]
                      }
                      frame 3 {
                        w392 = 25.0  # Pixel Width (microns)
                        w393 = 1.0  # Magnification
                        w394 = -2.77  # Detector Angle (degrees)
                        w395 = 31.85  # Inclusion Angle (degrees)
                        w396 = 297.6  # Focal Length (mm)
                        w397 = 0.000251338  # Slope Adjust
                        w398 = -1.24655  # Center Offset
                        n267 = Bundle("Center Offset"=w398, "Slope Adjust"=w397, "Focal Length (mm)"=w396, "Inclusion Angle (degrees)"=w395, "Detector Angle (degrees)"=w394, "Magnification"=w393, "Pixel Width (microns)"=w392) -> (w391:T6)  [unwired: 1 in]
                      }
                    }
                    n268 = call "CameraOpen.vi"("Camera Device ID"=w372) -> ("error out"=w349:errorcluster, "Camera Handle"=w343:u32)  [unwired: 1 in]
                    n269 = call "CameraGetTemp.vi"("Camera Handle"=w343, "error in (no error)"=w349) -> ("Camera Handle"=w371:u32, "Temperature"=w346:dbl, "error out"=w370:errorcluster)
                    n270 = local write "OMA V temp"(w346) -> ()
                    n271 = call "CalibOpen.vi"("Spectrometer Handle"=w339, "Detector Handle"=w343, "error in"=w338, "Detector Position"=u32 0, "Calibration Type"=u32 1, "Calibration Device ID"=u32 0) -> ("error out"=w321:errorcluster, "Calibration Handle"=w320:u32)
                    n272 = call "ExSubOMAVStrip.vi"("error in (no error)"=w370, "Camera Handle"=w371) -> ("error out"=w358:errorcluster, "Camera Handle"=w357:u32)
                    n273 = call "ExSubSetupCam.vi"("error in (no error)"=w358, "Camera Handle"=w357) -> ("error out"=w359:errorcluster, "Camera Handle"=w363:u32)
                    n274 = call "CameraTrigger.vi"("error in"=w359, "Trigger Edge"=w360, "Timing Mode"=w361, "Camera Handle"=w363) -> ("error out"=w364:errorcluster, "Camera Handle"=w362:u32)
                    n275 = Bundle("Acquire / focus mode \n1 is Sync circualar buffers"=w369, "OMA V exposure time"=w348, "Number of Images"=w368, "Number of software\naccumulations"=w367) -> (w366:T8)  [unwired: 1 in]
                    n276 = call "ExSubInitCam.vi"("error in (no error)"=w364, "Camera Information"=w366, "Camera Handle"=w362) -> ("error out"=w352:errorcluster, "Camera Handle"=w354:u32)
                    n277 = call "CalibSetAdjVals.vi"("Calibration Handle"=w320, "Turret Number"=w329, "Grating Number"=w322, "error in"=w321, "Spectrometer Calibration Parameters"=w319) -> ("Calibration Handle"=w332:u32, "error out"=w334:errorcluster)
                    n278 = call "CalibSetSpectInfo.vi"("Calibration Handle"=w332, "Current Grating Number"=w322, "Current Wavelength"=w328, "error in"=w334, "Current Turret Number"=w329) -> ("Calibration Handle"=w331:u32, "error out"=w335:errorcluster)
                    n279 = Path To String(path=path "C:/LabView_Projects/LifeEye/OMAV.txt" ("Full File Name\nfor Acqure")) -> (string=w356:string)
                    n280 = call "CameraADCset.vi"("error in (no error)"=w352, "ADC Gain"=2, "ADC Speed"=-1, "Camera Handle"=w354) -> ("error out"=w351:errorcluster, "Camera Handle"=w353:u32)  [unwired: 2 in]
                    n281 = call "ExSubCreateFileStrip.vi"("error in (no error)"=w351, "File and Display Name"=w356, "Pulser Handle"=w365, "Camera Handle"=w353) -> ("error out"=w326:errorcluster, "Handles Out"=w327:T5)
                    n282 = local write "OMA V Handles Out"(w327) -> ()
                    n283 = Unbundle(w327) -> ("Camera Handle"=w324:u32)  [unwired: 4 out]
                    n284 = call "CalibGetCalibArray.vi"("error in"=w335, "Array Size"=u32 1024, "Calibration Handle"=w331) -> ("error out"=w336:errorcluster, "Calibrated Array"=w330:dbl[], "Calibration Handle"=w333:u32)
                    n285 = local write "Mono Calibration Handle"(w333) -> ()
                    n286 = local write "OMA V Calibrated Array"(w330) -> ()
                    n287 = local write "MonoError"(w336) -> ()
                    n288 = call "CameraADCget.vi"("Camera handle"=w324, "error in (no error)"=w326) -> ("ADC Gain"=w323:i32, "error out"=w325:errorcluster)  [unwired: 6 out]
                    n289 = case shown="2" w323 {
                      frame 0, Default {
                      }
                      frame 2 {
                        w373 = u32 1 items=["low", "high"] ("OMA V gain")
                        n290 = local write "OMA V gain"(w373) -> ()
                      }
                      frame 1 {
                        w374 = u32 0 items=["low", "high"] ("OMA V gain")
                        n291 = local write "OMA V gain"(w374) -> ()
                      }
                    }
                    n292 = call "ToolKitIsError.vi"("error in"=w325) -> ("error out"=w345:errorcluster)  [unwired: 1 in, 1 out]
                    n293 = Not(x=w345) -> (.not. x?=w344:bool)
                    n294 = local write "OMA  V ON"(w344) -> ()
                  }
                  frame #2 {
                    n295 = local write "Busy"(FALSE ("Busy")) -> ()
                  }
                }
              }
            }
          }
          event "OMA V Start Aquire": Value Change {
            n296 = event-data() -> ()  [unwired: 1 in, 6 out]
            n297 = local read "OMA  V ON"() -> (w401:bool)
            n298 = local read "Mono ON"() -> (w402:bool)
            n299 = And(x=w402, y=w401) -> (x .and. y?=w403:bool)
            n300 = case shown="True" w403 {
              tunnel: [_ 27] -> w400
              frame False {
              }
              frame True {
              }
            }
          }
          event "OMA V correct background": Value Change {
            n301 = event-data() -> ()  [unwired: 1 in, 6 out]
            n302 = local read "OMA  V ON"() -> (w407:bool)
            n303 = local read "Mono ON"() -> (w406:bool)
            n304 = And(x=w407, y=w406) -> (x .and. y?=w405:bool)
            n305 = case shown="True" w405 {
              frame False {
              }
              frame True {
                n306 = local read "OMA V error"() -> (w411:errorcluster)
                n307 = local read "OMA V Handles Out"() -> (w413:T5)
                n308 = local read "OMA V correct background"() -> (w410:bool)
                n309 = Unbundle(w413) -> ("Camera Handle"=w412:u32)  [unwired: 4 out]
                n310 = case shown="True" w410 {
                  tunnel: [0 0] -> w409
                  frame False {
                  }
                  frame True {
                    n311 = local write "OMA V correct background"(FALSE ("OMA V correct background")) -> ()
                  }
                }
                n312 = call "CameraOnlineBackSubSetup.vi"("error in"=w411, "Background Flag"=w409, "Camera Handle"=w412) -> ("error out"=w408:errorcluster)  [unwired: 1 in, 2 out]
                n313 = local write "OMA V error"(w408) -> ()
              }
            }
          }
          event "OMA V gain": Value Change {
            n314 = event-data() -> ("NewVal"=w417:u32)  [unwired: 1 in, 5 out]
            n315 = local read "OMA  V ON"() -> (w418:bool)
            n316 = case shown="True" w418 {
              tunnel: w417 -> [_ w425]
              frame False {
              }
              frame True {
                n317 = Increment(x=w425) -> (x+1=w424:u32)
                n318 = local read "OMA V error"() -> (w420:errorcluster)
                n319 = local read "OMA V Handles Out"() -> (w423:T5)
                n320 = Unbundle(w423) -> ("Camera Handle"=w422:u32)  [unwired: 4 out]
                n321 = call "CameraADCset.vi"("error in (no error)"=w420, "ADC Gain"=w424, "ADC Speed"=-1, "Camera Handle"=w422) -> ("error out"=w419:errorcluster)  [unwired: 2 in, 1 out]
                n322 = local write "OMA V error"(w419) -> ()
              }
            }
          }
          event "OMA V get temp": Value Change {
            n323 = event-data() -> ()  [unwired: 1 in, 6 out]
            n324 = local read "OMA  V ON"() -> (w426:bool)
            n325 = case shown="True" w426 {
              frame False {
              }
              frame True {
                n326 = local read "OMA V error"() -> (w430:errorcluster)
                n327 = local read "OMA V Handles Out"() -> (w428:T5)
                n328 = Unbundle(w428) -> ("Camera Handle"=w427:u32)  [unwired: 4 out]
                n329 = call "CameraGetTemp.vi"("Camera Handle"=w427, "error in (no error)"=w430) -> ("Temperature"=w429:dbl, "error out"=w431:errorcluster)  [unwired: 1 out]
                n330 = local write "OMA V temp"(w429) -> ()
                n331 = local write "OMA V error"(w431) -> ()
              }
            }
          }
          event "OMA V set temp": Value Change {
            n332 = event-data() -> ()  [unwired: 1 in, 6 out]
            n333 = local read "OMA  V ON"() -> (w432:bool)
            n334 = case shown="True" w432 {
              frame False {
              }
              frame True {
                n335 = local read "OMA V error"() -> (w434:errorcluster)
                n336 = local read "OMA V Handles Out"() -> (w436:T5)
                n337 = local read "OMA V set temp"() -> (w437:i8)
                n338 = Unbundle(w436) -> ("Camera Handle"=w435:u32)  [unwired: 4 out]
                n339 = call "CameraSetTemp.vi"("error in (no error)"=w434, "Temperature"=w437, "Camera Handle"=w435) -> ("error out"=w433:errorcluster)  [unwired: 1 out]
                n340 = local write "OMA V error"(w433) -> ()
              }
            }
          }
          event "OMA V start background": Value Change {
            n341 = event-data() -> ()  [unwired: 1 in, 6 out]
            n342 = local read "OMA  V ON"() -> (w439:bool)
            n343 = case shown="False" w439 {
              tunnel: [_ 32] -> w438
              frame False {
              }
              frame True {
              }
            }
          }
          event "OMA V start Focus": Value Change {
            n344 = event-data() -> ()  [unwired: 1 in, 6 out]
            n345 = local read "OMA  V ON"() -> (w442:bool)
            n346 = case shown="False" w442 {
              tunnel: [_ 33] -> w441
              frame False {
              }
              frame True {
              }
            }
          }
          event "Get param": Value Change {
            n347 = event-data() -> ()  [unwired: 1 in, 6 out]
            n348 = flat-sequence {
              frame #0 {
                n349 = local read "Mono Calibration Handle"() -> (w444:u32)
                n350 = call "CalibGetID.vi"("Enumerated ID"=u32 44, "Calibration Handle"=w444) -> ("Value From Calibration"=w453:dbl)  [unwired: 1 in, 2 out]
                n351 = call "CalibGetID.vi"("Enumerated ID"=u32 45, "Calibration Handle"=w444) -> ("Value From Calibration"=w452:dbl)  [unwired: 1 in, 2 out]
                n352 = call "CalibGetID.vi"("Enumerated ID"=u32 46, "Calibration Handle"=w444) -> ("Value From Calibration"=w451:dbl)  [unwired: 1 in, 2 out]
                n353 = call "CalibGetID.vi"("Enumerated ID"=u32 47, "Calibration Handle"=w444) -> ("Value From Calibration"=w450:dbl)  [unwired: 1 in, 2 out]
                n354 = call "CalibGetID.vi"("Enumerated ID"=u32 48, "Calibration Handle"=w444) -> ("Value From Calibration"=w449:dbl)  [unwired: 1 in, 2 out]
                n355 = call "CalibGetID.vi"("Enumerated ID"=u32 49, "Calibration Handle"=w444) -> ("Value From Calibration"=w448:dbl)  [unwired: 1 in, 2 out]
                n356 = call "CalibGetID.vi"("Enumerated ID"=u32 14, "Calibration Handle"=w444) -> ("Value From Calibration"=w447:dbl)  [unwired: 1 in, 2 out]
                n357 = Bundle("Value From Calibration"=w453, "Value From Calibration"=w452, "Value From Calibration"=w451, "Value From Calibration"=w450, "Value From Calibration"=w449, "Value From Calibration"=w448, "Value From Calibration"=w447) -> (w445:T9)  [unwired: 1 in]
                n358 = local write "Adjusted Values"(w445) -> ()
              }
              frame #1 {
              }
            }
          }
        }
      }
      frame #1 {
        # "Case handler"
        n359 = case shown="16" w460 {
          frame 0, Default {
          }
          frame 1 {
          }
          frame 2 {
          }
          frame 3 {
          }
          frame 4 {
          }
          frame 5 {
          }
          frame 6 {
          }
          frame 7 {
          }
          frame 8 {
          }
          frame 9 {
          }
          frame 10 {
          }
          frame 11 {
          }
          frame 12 {
          }
          frame 13 {
          }
          frame 14 {
            w468 = u32 2 ("y")
            # "PL start"
            # "Number of steps"
            # "Next step"
            # "Start"
            n360 = local read "End Wavelength (nm)"() -> (w463:dbl)
            n361 = local read "Start Wavelength (nm)"() -> (w470:dbl)
            n362 = local read "StepW (nm)"() -> (w466:dbl)
            n363 = Subtract(x=w463, y=w470) -> (x-y=w465:dbl)
            n364 = Divide(x=w465, y=w466) -> (x/y=w464:dbl)
            n365 = To Unsigned Long Integer(number=w464) -> (unsigned 32bit integer=w462:u32)
            n366 = Increment(x=w462) -> ()  [unwired: 1 out]
            n367 = Less?(x=w462, y=w468) -> (x < y?=w467:bool)
            n368 = local read "Mono handle"() -> (w472:u32)
            n369 = local read "MonoError"() -> (w473:errorcluster)
            n370 = Select(t=w465, s=w467, f=w466) -> (s? t:f=w469:dbl)
            n371 = Select(t=w468, s=w467, f=w462) -> (s? t:f=w471:u32)
            n372 = stacked-sequence {
              seq-local: [w484 _ _] -> [_ w586 _]
              seq-local: [w483 _ _] -> [_ w585 _]
              seq-local: [_ w586 _] -> [_ _ w588]
              seq-local: [_ w585 _] -> [_ _ w587]
              tunnel: w469 -> [w504 _ _]
              tunnel: w470 -> [w503 _ _]
              tunnel: w473 -> [w478 _ _]
              tunnel: w472 -> [w479 _ _]
              tunnel: w471 -> [w502 _ _]
              frame #0 {
                w475 = i16 1 ("Filter Wheel Number")
                n373 = call "SpectGetFilter.vi"("error in"=w478, "Filter Wheel Number"=w475, "Spectrometer Handle"=w479) -> ("error out"=w476:errorcluster, "Filter Number"=w474:i16, "Spectrometer Handle"=w477:u32)
                n374 = call "SpectSetFilter.vi"("Filter Number"=i16 6 ("Filter Wheel Number"), "error in"=w476, "Filter Wheel Number"=w475, "Spectrometer Handle"=w477) -> ("error out"=w500:errorcluster, "Spectrometer Handle"=w501:u32)
                n375 = local write "FilterWheelTemp"(w474) -> ()
                n376 = call "ExSubWaitSpec.vi"("error in (no error)"=w500, "Spectrometer Handle"=w501) -> ("error out"=w498:errorcluster, "Spectrometer handle"=w499:u32)
                n377 = call "SpectGetFilter.vi"("error in"=w498, "Filter Wheel Number"=i16 1, "Spectrometer Handle"=w499) -> ("error out"=w493:errorcluster, "Filter Number"=w497:i16, "Spectrometer Handle"=w494:u32)
                n378 = local write "Filter Wheel Position"(w497) -> ()
                n379 = while {
                  tunnel: w504 -> [w543]
                  shift-right: [w542] -> _
                  shift-left: w503 -> [w525]
                  tunnel: w502 -> [w517]
                  shift-right: [w533] -> w485
                  shift-left: w494 -> [w523]
                  shift-right: [w537] -> w481
                  shift-left: w493 -> [w524]
                  i -> [w540]
                  stop <- w518 continue-if-true
                  n380 = Decrement(x=w517) -> ()  [unwired: 1 out]
                  n381 = local read "PicoHarp ON"() -> (w536:bool)
                  n382 = local read "LockIn ON"() -> (w535:bool)
                  n383 = Add(x=w525, y=w543) -> (x+y=w542:dbl)
                  n384 = call "SpectSetWavelength.vi"("error in"=w524, "Wavelength"=w525, "Spectrometer Handle"=w523) -> ("error out"=w527:errorcluster, "Spectrumeter Handle"=w526:u32)
                  n385 = Equal?(x=0, y=w540) -> (x = y?=w541:bool)
                  n386 = local read "Stop Measurement"() -> (w538:bool)
                  n387 = Or(x=w536, y=w535) -> (x .or. y?=w534:bool)
                  n388 = call "ExSubWaitSpec.vi"("error in (no error)"=w527, "Spectrometer Handle"=w526) -> ("error out"=w528:errorcluster, "Spectrometer handle"=w529:u32)
                  n389 = Greater?(x=w517, y=w540) -> (0:w531:bool)
                  n390 = Not(x=w538) -> (.not. x?=w530:bool)
                  n391 = call "SpectGetGratingInfo.vi"("Spectrometer Handle"=w529, "error in"=w528) -> ("Current Wavelength"=w520:dbl, "Spectrometer Handle"=w521:u32, "error out"=w522:errorcluster)  [unwired: 3 out]
                  n392 = local write "Wavelength (nm)"(w520) -> ()
                  n393 = case shown="True" w541 {
                    tunnel: [w545 w547] -> w533
                    tunnel: [w544 w549] -> w532
                    tunnel: w521 -> [w545 w553]
                    tunnel: w522 -> [w544 w552]
                    frame False {
                    }
                    frame True {
                      n394 = local read "FilterWheelTemp"() -> (w546:i32)
                      n395 = call "SpectSetFilter.vi"("Filter Number"=w546, "error in"=w552, "Filter Wheel Number"=i16 1, "Spectrometer Handle"=w553) -> ("error out"=w558:errorcluster, "Spectrometer Handle"=w559:u32)
                      n396 = call "ExSubWaitSpec.vi"("error in (no error)"=w558, "Spectrometer Handle"=w559) -> ("error out"=w556:errorcluster, "Spectrometer handle"=w557:u32)
                      n397 = call "SpectGetFilter.vi"("error in"=w556, "Filter Wheel Number"=i16 1, "Spectrometer Handle"=w557) -> ("error out"=w550:errorcluster, "Filter Number"=w551:i16, "Spectrometer Handle"=w548:u32)
                      n398 = local write "Filter Wheel Position"(w551) -> ()
                      n399 = flat-sequence {
                        tunnel: w550 -> [w562]
                        tunnel: [w562] -> w549
                        tunnel: w548 -> [w561]
                        tunnel: [w561] -> w547
                        tunnel: [w560] -> _
                        frame #0 {
                          n400 = Tick Count (ms)() -> (millisecond timer value=w560:u32)
                          n401 = local write "timestart"(w560) -> ()
                        }
                      }
                    }
                  }
                  n402 = And(x=w531, y=w530) -> (x .and. y?=w519:bool)
                  n403 = case shown="False" w534 {
                    tunnel: w532 -> [w568 w584]
                    tunnel: [w567 w584] -> w537
                    tunnel: w520 -> [_ _]
                    tunnel: w519 -> [w563 w583]
                    tunnel: [w563 w583] -> w518
                    frame False {
                      n404 = local read "PiezoStage ON"() -> (w564:bool)
                      n405 = And(x="PL_Clock", y=w564) -> (x .and. y?=w565:bool)
                      n406 = case shown="True" w565 {
                        tunnel: w568 -> [w569 w575]
                        tunnel: [w569 w575] -> w567
                        frame False {
                          n407 = local read "Step Delay (s)"() -> (w571:dbl)
                          n408 = Multiply(x=w571, y=1000.0) -> (x*y=w572:dbl)
                          n409 = Wait (ms)(milliseconds to wait=w572) -> ()  [unwired: 1 out]
                        }
                        frame True {
                          n410 = flat-sequence {
                            tunnel: [w576] -> w573
                            tunnel: [w578] -> w574
                            tunnel: w573 -> [w578]
                            tunnel: w574 -> [w582]
                            frame #0 {
                              n411 = local read "Piezohandle"() -> (w577:i32)
                              n412 = dll-call lib="C:/LabView_Projects/LifeEye/32bitDLLs/Madlib.dll" fn="MCL_PixelClock"("handle"=w577) -> ("handle"=w576:i32)  [unwired: 4 in, 2 out]
                            }
                            frame #1 {
                              n413 = local read "Step Delay (s)"() -> (w579:dbl)
                              n414 = Multiply(x=w579, y=1000.0) -> (x*y=w581:dbl)
                              n415 = Wait (ms)(milliseconds to wait=w581) -> ()  [unwired: 1 out]
                            }
                            frame #2 {
                              n416 = dll-call lib="C:/LabView_Projects/LifeEye/32bitDLLs/Madlib.dll" fn="MCL_LineClock"("handle"=w582) -> ()  [unwired: 5 in, 2 out]
                            }
                          }
                        }
                      }
                    }
                    frame True {
                    }
                  }
                }
                n417 = flat-sequence {
                  tunnel: w481 -> [w516]
                  tunnel: [w516] -> w480
                  frame #0 {
                    n418 = Tick Count (ms)() -> (millisecond timer value=w513:u32)
                    n419 = local read "StepW (nm)"() -> (w506:dbl)
                    n420 = local read "timestart"() -> (w509:i64)
                    n421 = local write "timeend"(w513) -> ()
                    n422 = local read "End Wavelength (nm)"() -> (w515:dbl)
                    n423 = local read "Start Wavelength (nm)"() -> (w514:dbl)
                    n424 = Subtract(x=w513, y=w509) -> (x-y=w511:i64)
                    n425 = Divide(x=w511, y=u32 1000) -> (x/y=w508:dbl)
                    n426 = Subtract(x=w515, y=w514) -> (x-y=w507:dbl)
                    n427 = Divide(x=w507, y=w506) -> (x/y=w505:dbl)
                    n428 = Divide(x=w508, y=w505) -> (x/y=w512:dbl)
                    n429 = local write "Real Delay (seconds/step)"(w512) -> ()
                  }
                }
                n430 = call "SpectSetFilter.vi"("Filter Number"=i16 6 ("Filter Wheel Number"), "error in"=w480, "Filter Wheel Number"=i16 1, "Spectrometer Handle"=w485) -> ("error out"=w491:errorcluster, "Spectrometer Handle"=w492:u32)
                n431 = call "ExSubWaitSpec.vi"("error in (no error)"=w491, "Spectrometer Handle"=w492) -> ("error out"=w489:errorcluster, "Spectrometer handle"=w490:u32)
                n432 = call "SpectGetFilter.vi"("error in"=w489, "Filter Wheel Number"=i16 1, "Spectrometer Handle"=w490) -> ("error out"=w483:errorcluster, "Filter Number"=w482:i16, "Spectrometer Handle"=w484:u32)
                n433 = local write "Filter Wheel Position"(w482) -> ()
              }
              frame #1 {
              }
              frame #2 {
                n434 = local write "Mono handle"(w588) -> ()
                n435 = local write "MonoError"(w587) -> ()
              }
            }
          }
          frame 15 {
            w592 = u32 2 ("y")
            # "Number of steps"
            # "Next step"
            # "Start"
            n436 = local read "EndZ (µm)"() -> (w594:dbl)
            n437 = local read "StartZ (µm)"() -> (w595:dbl)
            n438 = local read "StepZ (µm)"() -> (w598:dbl)
            n439 = Subtract(x=w594, y=w595) -> (x-y=w590:dbl)
            n440 = Divide(x=w590, y=w598) -> (x/y=w589:dbl)
            n441 = To Unsigned Long Integer(number=w589) -> (unsigned 32bit integer=w593:u32)
            n442 = Less?(x=w593, y=w592) -> (x < y?=w591:bool)
            n443 = Select(t=w590, s=w591, f=w598) -> (s? t:f=w596:dbl)
            n444 = Select(t=w592, s=w591, f=w593) -> (s? t:f=w597:u32)
            n445 = stacked-sequence {
              tunnel: w595 -> [w601 _]
              tunnel: w596 -> [w600 _]
              tunnel: w597 -> [w599 _]
              frame #0 {
                n446 = while {
                  shift-right: [w610] -> _
                  shift-left: w601 -> [w613]
                  tunnel: w600 -> [w612]
                  tunnel: w599 -> [w608]
                  i -> [w609]
                  stop <- w603 continue-if-true
                  n447 = flat-sequence {
                    tunnel: w613 -> [w621]
                    tunnel: w612 -> [w620]
                    tunnel: [w619] -> w611
                    tunnel: w609 -> [w618]
                    tunnel: w608 -> [w617]
                    tunnel: [w616] -> w607
                    tunnel: [w614] -> w606
                    tunnel: [w629] -> w610
                    tunnel: w611 -> [w629]
                    tunnel: [w628] -> w602
                    tunnel: w607 -> [w628]
                    tunnel: w606 -> [w627]
                    frame #0 {
                      w624 = FALSE ("commandX")
                      n448 = Greater?(x=w617, y=w618) -> (0:w616:bool)
                      n449 = Add(x=w621, y=w620) -> (x+y=w619:dbl)
                      n450 = local read "Piezohandle"() -> (w614:i32)
                      n451 = call "_subvi_LivePos_Main.vi"("zCommand"=w621, "handle"=w614, "counter"=u32 50, "commandZ"=TRUE, "commandY"=w624, "commandX"=w624) -> ("xRead"=w623:dbl, "yRead"=w622:dbl, "zRead"=w615:dbl)  [unwired: 2 in, 9 out]
                      n452 = local write "xRead"(w623) -> ()
                      n453 = local write "yRead"(w622) -> ()
                      n454 = local write "zRead"(w615) -> ()
                    }
                    frame #1 {
                      n455 = local read "PicoHarp ON"() -> (w630:bool)
                      n456 = local read "Pixel Delay (s)"() -> (w631:dbl)
                      n457 = case shown="False" w630 {
                        tunnel: w631 -> [w634 _]
                        tunnel: w627 -> [w632 _]
                        frame False {
                          n458 = flat-sequence {
                            tunnel: w634 -> [w637]
                            tunnel: [w635] -> w633
                            tunnel: w632 -> [w635]
                            tunnel: w633 -> [w640]
                            frame #0 {
                              n459 = Multiply(x=w637, y=1000.0) -> (x*y=w636:dbl)
                              n460 = Wait (ms)(milliseconds to wait=w636) -> ()  [unwired: 1 out]
                            }
                            frame #1 {
                              n461 = dll-call lib="C:/LabView_Projects/LifeEye/32bitDLLs/Madlib.dll" fn="MCL_SingleReadN"("axis"=u32 3, "handle"=w640) -> ()  [unwired: 5 in, 3 out]
                            }
                          }
                        }
                        frame True {
                        }
                      }
                    }
                  }
                  n462 = local read "Stop Measurement"() -> (w604:bool)
                  n463 = Not(x=w604) -> (.not. x?=w605:bool)
                  n464 = And(x=w605, y=w602) -> (x .and. y?=w603:bool)
                }
              }
              frame #1 {
              }
            }
          }
          frame 16 {
            # "Int map start"
            n465 = flat-sequence {
              frame #0 {
                w653 = u32 2 ("y")
                w660 = u32 2 ("y")
                # "Number of stepsY"
                # "Next stepY"
                # "StartY"
                # "Number of stepsX"
                # "Next stepX"
                # "StartX"
                n466 = local write "Forwardpix_scan"(FALSE ("Forwardpix_scan")) -> ()
                n467 = local read "Piezohandle"() -> (w646:i32)
                n468 = Subtract(x="EndX (µm)", y="StartX (µm)") -> (x-y=w662:dbl)
                n469 = Subtract(x="EndY (µm)", y="StartY (µm)") -> (x-y=w655:dbl)
                n470 = Divide(x=w662, y="StepX (µm)") -> (x/y=w663:dbl)
                n471 = Divide(x=w655, y="StepY (µm)") -> (x/y=w656:dbl)
                n472 = To Unsigned Long Integer(number=w656) -> (unsigned 32bit integer=w642:u32)
                n473 = To Unsigned Long Integer(number=w663) -> (unsigned 32bit integer=w643:u32)
                n474 = Increment(x=w643) -> ()  [unwired: 1 out]
                n475 = Increment(x=w642) -> (x+1=w641:u32)
                n476 = Less?(x=w643, y=w660) -> (x < y?=w661:bool)
                n477 = Less?(x=w641, y=w653) -> (x < y?=w654:bool)
                n478 = Select(t=w662, s=w661, f="StepX (µm)") -> (s? t:f=w657:dbl)
                n479 = Select(t=w655, s=w654, f="StepY (µm)") -> (s? t:f=w650:dbl)
                n480 = Select(t=w660, s=w661, f=w643) -> (s? t:f=w647:u32)
                n481 = Select(t=w653, s=w654, f=w641) -> (s? t:f=w648:u32)
                n482 = while {
                  tunnel: w647 -> [w685]
                  tunnel: w657 -> [w683]
                  shift-right: [w682] -> _
                  shift-left: "StartY (µm)" -> [w675]
                  tunnel: w648 -> [w667]
                  tunnel: "StartX (µm)" -> [w686]
                  tunnel: [w684] -> _
                  tunnel: w650 -> [w681]
                  shift-right: [w668] -> _
                  shift-left: w646 -> [w674]
                  tunnel: "EndX (µm)" -> [w670]
                  tunnel: [w669] -> _
                  i -> [w679]
                  stop <- w664 continue-if-true
                  # "startX"
                  # "endX"
                  n483 = flat-sequence {
                    tunnel: w675 -> [w690]
                    tunnel: w674 -> [w695]
                    tunnel: [w695] -> w673
                    tunnel: w673 -> [w706]
                    tunnel: [w706] -> w671
                    tunnel: [w707] -> w672
                    tunnel: w671 -> [w707]
                    frame #0 {
                      n484 = local read "Bidirectional scan"() -> (w692:bool)
                      n485 = case shown="False" w692 {
                        tunnel: [w698 _] -> w691
                        tunnel: [TRUE FALSE] -> w693
                        frame False {
                          n486 = local read "StartX (µm)"() -> (w698:dbl)
                        }
                        frame True {
                        }
                      }
                      n487 = call "_subvi_LivePos_Main.vi"("xCommand"=w691, "yCommand"=w690, "handle"=w695, "counter"=u32 50, "commandZ"=FALSE, "commandY"=TRUE, "commandX"=w693) -> ()  [unwired: 1 in, 12 out]
                    }
                    frame #1 {
                      # "interline delay"
                      n488 = local read "Interline Delay (s)"() -> (w701:dbl)
                      n489 = Multiply(x=w701, y=1000.0) -> (x*y=w702:dbl)
                      n490 = local read "Forwardpix_scan"() -> (w705:bool)
                      n491 = Wait (ms)(milliseconds to wait=w702) -> ()  [unwired: 1 out]
                      n492 = Not(x=w705) -> (.not. x?=w704:bool)
                      n493 = local write "Forwardpix_scan"(w704) -> ()
                    }
                    frame #2 {
                    }
                  }
                  n494 = Add(x=w675, y=w681) -> (x+y=w682:dbl)
                  n495 = Decrement(x=w667) -> (x-1=w666:u32)
                  n496 = Greater?(x=w666, y=w679) -> (0:w680:bool)
                  n497 = local read "Stop Measurement"() -> (w676:bool)
                  n498 = while {
                    shift-right: [w718] -> w684
                    shift-left: w686 -> [w719]
                    tunnel: w685 -> [w733]
                    tunnel: w683 -> [w722]
                    shift-right: [w729] -> w678
                    shift-left: w680 -> [w730]
                    tunnel: w679 -> [w726]
                    shift-right: [w723] -> w668
                    shift-left: w672 -> [w723]
                    shift-right: [w718] -> w669
                    shift-left: w670 -> [w720]
                    i -> [w728]
                    stop <- w713 continue-if-true
                    n499 = local read "Piezohandle"() -> (w709:i32)
                    n500 = local read "Stop Measurement"() -> (w724:bool)
                    n501 = local read "Bidirectional scan"() -> (w715:bool)
                    n502 = local read "Forwardpix_scan"() -> (w717:bool)
                    n503 = Greater?(x=w733, y=w728) -> (0:w710:bool)
                    n504 = Not(x=w724) -> (.not. x?=w711:bool)
                    n505 = Not(x=w717) -> (.not. x?=w716:bool)
                    n506 = And(x=w711, y=w710) -> (x .and. y?=w712:bool)
                    n507 = And(x=w715, y=w716) -> (x .and. y?=w714:bool)
                    n508 = case shown="False" w712 {
                      selector: w712 -> [w736 w738]
                      tunnel: [w736 w738] -> w713
                      tunnel: w709 -> [w735 w737]
                      tunnel: [w734 w737] -> w708
                      frame False {
                        n509 = dll-call lib="C:/LabView_Projects/LifeEye/32bitDLLs/Madlib.dll" fn="MCL_LineClock"("handle"=w735) -> ("handle"=w734:i32)  [unwired: 4 in, 2 out]
                      }
                      frame True {
                      }
                    }
                    n510 = case shown="True" w714 {
                      tunnel: w720 -> [_ w742]
                      tunnel: w722 -> [w740 w744]
                      tunnel: [w741 w743] -> w718
                      tunnel: [w739 w742] -> w721
                      tunnel: w719 -> [w739 _]
                      frame False {
                        n511 = Add(x=w739, y=w740) -> (x+y=w741:dbl)
                      }
                      frame True {
                        n512 = Subtract(x=w742, y=w744) -> (x-y=w743:dbl)
                      }
                    }
                    n513 = flat-sequence {
                      tunnel: w721 -> [w752]
                      tunnel: [w747] -> w732
                      tunnel: [w754] -> w731
                      tunnel: w730 -> [w754]
                      tunnel: [w749] -> _
                      tunnel: w728 -> [w749]
                      tunnel: [w749] -> w727
                      tunnel: w726 -> [w753]
                      tunnel: [w753] -> w725
                      tunnel: w708 -> [w745]
                      tunnel: w732 -> [w764]
                      tunnel: w731 -> [w763]
                      tunnel: [w763] -> w729
                      tunnel: w727 -> [w762]
                      tunnel: w725 -> [w761]
                      frame #0 {
                        n514 = Equal?(x=w749, y=0) -> (x = y?=w750:bool)
                        n515 = dll-call lib="C:/LabView_Projects/LifeEye/32bitDLLs/Madlib.dll" fn="MCL_SingleWriteN"("position"=w752, "axis"=u32 1, "handle"=w745) -> ("handle"=w746:i32)  [unwired: 5 in, 3 out]
                        n516 = case shown="True" w750 {
                          tunnel: w746 -> [w755 w757]
                          tunnel: [w755 w756] -> w747
                          frame False {
                          }
                          frame True {
                            n517 = dll-call lib="C:/LabView_Projects/LifeEye/32bitDLLs/Madlib.dll" fn="MCL_PixelClock"("handle"=w757) -> ("handle"=w756:i32)  [unwired: 4 in, 2 out]
                          }
                        }
                      }
                      frame #1 {
                        n518 = local read "PicoHarp ON"() -> (w760:bool)
                        n519 = local read "LockIn ON"() -> (w759:bool)
                        n520 = Or(x=w760, y=w759) -> (x .or. y?=w758:bool)
                        n521 = case shown="True" w758 {
                          tunnel: "Pixel Delay (s)" -> [w769 _]
                          tunnel: w764 -> [w767 _]
                          tunnel: w762 -> [_ _]
                          tunnel: w761 -> [_ _]
                          frame False {
                            n522 = flat-sequence {
                              tunnel: w769 -> [w772]
                              tunnel: [w771] -> w768
                              tunnel: w767 -> [w771]
                              tunnel: w768 -> [w774]
                              tunnel: [w774] -> w766
                              tunnel: w766 -> [w775]
                              frame #0 {
                                n523 = Multiply(x=w772, y=1000.0) -> (x*y=w770:dbl)
                                n524 = Wait (ms)(milliseconds to wait=w770) -> ()  [unwired: 1 out]
                              }
                              frame #1 {
                              }
                              frame #2 {
                                n525 = dll-call lib="C:/LabView_Projects/LifeEye/32bitDLLs/Madlib.dll" fn="MCL_SingleReadN"("axis"=u32 1, "handle"=w775) -> ("position"=w778:dbl)  [unwired: 5 in, 2 out]
                                n526 = dll-call lib="C:/LabView_Projects/LifeEye/32bitDLLs/Madlib.dll" fn="MCL_SingleReadN"("axis"=u32 2, "handle"=w775) -> ("position"=w779:dbl)  [unwired: 5 in, 2 out]
                                n527 = local write "xRead"(w778) -> ()
                                n528 = local write "yRead"(w779) -> ()
                              }
                            }
                          }
                          frame True {
                          }
                        }
                      }
                    }
                  }
                  n529 = Not(x=w676) -> (.not. x?=w677:bool)
                  n530 = And(x=w677, y=w678) -> (x .and. y?=w665:bool)
                  n531 = case shown="True" w665 {
                    selector: w665 -> [w687 w689]
                    tunnel: [w687 w689] -> w664
                    frame False {
                      n532 = local read "Piezohandle"() -> (w688:i32)
                      n533 = dll-call lib="C:/LabView_Projects/LifeEye/32bitDLLs/Madlib.dll" fn="MCL_FrameClock"("handle"=w688) -> ()  [unwired: 5 in, 2 out]
                    }
                    frame True {
                    }
                  }
                }
              }
              frame #1 {
              }
              frame #2 {
              }
            }
          }
          frame 17 {
            # "SpectrMap start"
            n534 = flat-sequence {
              tunnel: [w809] -> w781
              tunnel: [w808] -> w780
              tunnel: w781 -> [w935]
              tunnel: w780 -> [w936]
              frame #0 {
                w782 = i16 1 ("Filter Wheel Number")
                w815 = u32 2 ("y")
                # "Y step"
                # "Number of stepsW"
                # "Next step"
                # "StartY"
                # "X step"
                # "StartX"
                n535 = local read "Mono handle"() -> (w785:u32)
                n536 = local read "StartX (µm)"() -> (w805:dbl)
                n537 = local read "StartY (µm)"() -> (w804:dbl)
                n538 = local read "MonoError"() -> (w787:errorcluster)
                n539 = local read "End Wavelength (nm)"() -> (w810:dbl)
                n540 = local read "Number of Spectra"() -> (w790:i16)
                n541 = local read "EndX (µm)"() -> (w807:dbl)
                n542 = local read "EndY (µm)"() -> (w806:dbl)
                n543 = call "SpectGetFilter.vi"("error in"=w787, "Filter Wheel Number"=w782, "Spectrometer Handle"=w785) -> ("error out"=w786:errorcluster, "Filter Number"=w783:i16, "Spectrometer Handle"=w784:u32)
                n544 = local read "Start Wavelength (nm)"() -> (w812:dbl)
                n545 = Subtract(x=w807, y=w805) -> (x-y=w803:dbl)
                n546 = Subtract(x=w806, y=w804) -> (x-y=w802:dbl)
                n547 = local write "FilterWheelTemp"(w783) -> ()
                n548 = call "SpectSetFilter.vi"("Filter Number"=i16 6 ("Filter Wheel Number"), "error in"=w786, "Filter Wheel Number"=w782, "Spectrometer Handle"=w784) -> ("error out"=w798:errorcluster, "Spectrometer Handle"=w799:u32)
                n549 = Decrement(x=w790) -> (x-1=w789:i16)
                n550 = local read "StepW (nm)"() -> (w811:dbl)
                n551 = Divide(x=w803, y=w789) -> (x/y=w801:dbl)
                n552 = Divide(x=w802, y=w789) -> (x/y=w800:dbl)
                n553 = Subtract(x=w810, y=w812) -> (x-y=w817:dbl)
                n554 = call "ExSubWaitSpec.vi"("error in (no error)"=w798, "Spectrometer Handle"=w799) -> ("error out"=w796:errorcluster, "Spectrometer handle"=w797:u32)
                n555 = Divide(x=w817, y=w811) -> (x/y=w818:dbl)
                n556 = call "SpectGetFilter.vi"("error in"=w796, "Filter Wheel Number"=i16 1, "Spectrometer Handle"=w797) -> ("error out"=w791:errorcluster, "Filter Number"=w793:i16, "Spectrometer Handle"=w792:u32)
                n557 = To Unsigned Long Integer(number=w818) -> (unsigned 32bit integer=w788:u32)
                n558 = Increment(x=w788) -> ()  [unwired: 1 out]
                n559 = local write "Filter Wheel Position"(w793) -> ()
                n560 = Less?(x=w788, y=w815) -> (x < y?=w816:bool)
                n561 = Select(t=w817, s=w816, f=w811) -> (s? t:f=w814:dbl)
                n562 = Select(t=w815, s=w816, f=w788) -> (s? t:f=w813:u32)
                n563 = while {
                  tunnel: w790 -> [w850]
                  tunnel: w801 -> [w848]
                  shift-right: [w847] -> _
                  shift-left: w812 -> [w824]
                  tunnel: w813 -> [w821]
                  tunnel: w805 -> [w851]
                  tunnel: [w849] -> _
                  tunnel: w814 -> [w846]
                  shift-right: [w838] -> w809
                  shift-left: w792 -> [w832]
                  shift-right: [w835] -> w808
                  shift-left: w791 -> [w831]
                  tunnel: w804 -> [w834]
                  tunnel: w800 -> [w833]
                  i -> [w840]
                  stop <- w819 continue-if-true
                  n564 = Add(x=w824, y=w846) -> (x+y=w847:dbl)
                  n565 = Decrement(x=w821) -> (x-1=w822:u32)
                  n566 = call "SpectSetWavelength.vi"("error in"=w831, "Wavelength"=w824, "Spectrometer Handle"=w832) -> ("error out"=w829:errorcluster, "Spectrumeter Handle"=w830:u32)
                  n567 = Greater?(x=w822, y=w840) -> (0:w845:bool)
                  n568 = call "ExSubWaitSpec.vi"("error in (no error)"=w829, "Spectrometer Handle"=w830) -> ("error out"=w827:errorcluster, "Spectrometer handle"=w828:u32)
                  n569 = local read "Stop Measurement"() -> (w842:bool)
                  n570 = Equal?(x=0, y=w840) -> (x = y?=w839:bool)
                  n571 = call "SpectGetGratingInfo.vi"("Spectrometer Handle"=w828, "error in"=w827) -> ("Current Wavelength"=w823:dbl, "Spectrometer Handle"=w826:u32, "error out"=w825:errorcluster)  [unwired: 3 out]
                  n572 = local write "Wavelength (nm)"(w823) -> ()
                  n573 = case shown="True" w839 {
                    tunnel: [w856 w860] -> w836
                    tunnel: [w855 w859] -> w837
                    tunnel: w826 -> [w856 w862]
                    tunnel: w825 -> [w855 w861]
                    frame False {
                    }
                    frame True {
                      n574 = local read "FilterWheelTemp"() -> (w857:i32)
                      n575 = call "SpectSetFilter.vi"("Filter Number"=w857, "error in"=w861, "Filter Wheel Number"=i16 1, "Spectrometer Handle"=w862) -> ("error out"=w867:errorcluster, "Spectrometer Handle"=w868:u32)
                      n576 = call "ExSubWaitSpec.vi"("error in (no error)"=w867, "Spectrometer Handle"=w868) -> ("error out"=w865:errorcluster, "Spectrometer handle"=w866:u32)
                      n577 = call "SpectGetFilter.vi"("error in"=w865, "Filter Wheel Number"=i16 1, "Spectrometer Handle"=w866) -> ("error out"=w859:errorcluster, "Filter Number"=w863:i16, "Spectrometer Handle"=w860:u32)
                      n578 = local write "Filter Wheel Position"(w863) -> ()
                    }
                  }
                  n579 = while {
                    shift-right: [w894] -> w849
                    shift-left: w851 -> [w892]
                    tunnel: w850 -> [w873]
                    tunnel: w848 -> [w893]
                    shift-right: [w888] -> w844
                    shift-left: w845 -> [w889]
                    tunnel: w840 -> [w885]
                    shift-right: [w882] -> w838
                    shift-left: w836 -> [w882]
                    shift-right: [w881] -> w835
                    shift-left: w837 -> [w881]
                    shift-right: [w877] -> _
                    shift-left: w834 -> [w876]
                    tunnel: w833 -> [w878]
                    i -> [w887]
                    stop <- w879 continue-if-true
                    n580 = Add(x=w892, y=w893) -> (x+y=w894:dbl)
                    n581 = Add(x=w876, y=w878) -> (x+y=w877:dbl)
                    n582 = Decrement(x=w873) -> (x-1=w872:i16)
                    n583 = Greater?(x=w872, y=w887) -> (0:w875:bool)
                    n584 = local read "Stop Measurement"() -> (w883:bool)
                    n585 = Not(x=w883) -> (.not. x?=w874:bool)
                    n586 = And(x=w875, y=w874) -> (x .and. y?=w871:bool)
                    n587 = flat-sequence {
                      tunnel: w892 -> [w901]
                      tunnel: [w899] -> w891
                      tunnel: [w904] -> w890
                      tunnel: w889 -> [w904]
                      tunnel: [w902] -> _
                      tunnel: w887 -> [w902]
                      tunnel: [w902] -> w886
                      tunnel: w885 -> [w903]
                      tunnel: [w903] -> w884
                      tunnel: [w902] -> w880
                      tunnel: w876 -> [w900]
                      tunnel: w871 -> [w898]
                      tunnel: [w898] -> w870
                      tunnel: w891 -> [w912]
                      tunnel: w890 -> [w919]
                      tunnel: [w919] -> w888
                      tunnel: w886 -> [w918]
                      tunnel: w884 -> [w917]
                      tunnel: w880 -> [w913]
                      tunnel: [w911] -> w869
                      tunnel: w870 -> [w911]
                      frame #0 {
                        n588 = local read "Piezohandle"() -> (w899:i32)
                        n589 = flat-sequence {
                          tunnel: w901 -> [w906]
                          tunnel: w899 -> [w905]
                          tunnel: w900 -> [w909]
                          tunnel: w899 -> [w908]
                          frame #0 {
                            n590 = dll-call lib="C:/LabView_Projects/LifeEye/32bitDLLs/Madlib.dll" fn="MCL_SingleWriteN"("position"=w906, "axis"=u32 1, "handle"=w905) -> ()  [unwired: 6 in, 3 out]
                          }
                          frame #1 {
                            n591 = dll-call lib="C:/LabView_Projects/LifeEye/32bitDLLs/Madlib.dll" fn="MCL_SingleWriteN"("position"=w909, "axis"=u32 2, "handle"=w908) -> ()  [unwired: 6 in, 3 out]
                          }
                        }
                      }
                      frame #1 {
                        n592 = Equal?(x=w913, y=0) -> (x = y?=w914:bool)
                        n593 = local read "PicoHarp ON"() -> (w920:bool)
                        n594 = case shown="True" w914 {
                          tunnel: w912 -> [_ w921]
                          frame False {
                          }
                          frame True {
                            n595 = dll-call lib="C:/LabView_Projects/LifeEye/32bitDLLs/Madlib.dll" fn="MCL_PixelClock"("handle"=w921) -> ()  [unwired: 5 in, 2 out]
                          }
                        }
                        n596 = local read "Pixel Delay (s)"() -> (w916:dbl)
                        n597 = case shown="False" w920 {
                          tunnel: w916 -> [w924 _]
                          tunnel: w912 -> [w922 _]
                          tunnel: w918 -> [_ _]
                          tunnel: w917 -> [_ _]
                          frame False {
                            n598 = flat-sequence {
                              tunnel: w924 -> [w926]
                              tunnel: [w925] -> w923
                              tunnel: w922 -> [w925]
                              tunnel: w923 -> [w932]
                              frame #0 {
                                n599 = Multiply(x=w926, y=1000.0) -> (x*y=w927:dbl)
                                n600 = Wait (ms)(milliseconds to wait=w927) -> ()  [unwired: 1 out]
                              }
                              frame #1 {
                                n601 = dll-call lib="C:/LabView_Projects/LifeEye/32bitDLLs/Madlib.dll" fn="MCL_SingleReadN"("axis"=u32 1, "handle"=w932) -> ("position"=w934:dbl, "handle"=w929:i32)  [unwired: 4 in, 2 out]
                                n602 = local write "xRead"(w934) -> ()
                                n603 = dll-call lib="C:/LabView_Projects/LifeEye/32bitDLLs/Madlib.dll" fn="MCL_SingleReadN"("axis"=u32 2, "handle"=w929) -> ("position"=w931:dbl)  [unwired: 5 in, 2 out]
                                n604 = local write "yRead"(w931) -> ()
                              }
                            }
                          }
                          frame True {
                          }
                        }
                      }
                    }
                    n605 = case shown="False" w869 {
                      selector: w869 -> [w895 w897]
                      tunnel: [w895 w897] -> w879
                      frame False {
                        n606 = local read "Piezohandle"() -> (w896:i32)
                        n607 = dll-call lib="C:/LabView_Projects/LifeEye/32bitDLLs/Madlib.dll" fn="MCL_LineClock"("handle"=w896) -> ()  [unwired: 5 in, 2 out]
                      }
                      frame True {
                      }
                    }
                  }
                  n608 = Not(x=w842) -> (.not. x?=w843:bool)
                  n609 = And(x=w843, y=w844) -> (x .and. y?=w820:bool)
                  n610 = case shown="False" w820 {
                    selector: w820 -> [w852 w854]
                    tunnel: [w852 w854] -> w819
                    frame False {
                      n611 = local read "Piezohandle"() -> (w853:i32)
                      n612 = dll-call lib="C:/LabView_Projects/LifeEye/32bitDLLs/Madlib.dll" fn="MCL_FrameClock"("handle"=w853) -> ()  [unwired: 5 in, 2 out]
                    }
                    frame True {
                    }
                  }
                }
              }
              frame #1 {
                n613 = call "SpectSetFilter.vi"("Filter Number"=i16 6 ("Filter Wheel Number"), "error in"=w936, "Filter Wheel Number"=i16 1, "Spectrometer Handle"=w935) -> ("error out"=w945:errorcluster, "Spectrometer Handle"=w946:u32)
                n614 = call "ExSubWaitSpec.vi"("error in (no error)"=w945, "Spectrometer Handle"=w946) -> ("error out"=w943:errorcluster, "Spectrometer handle"=w944:u32)
                n615 = call "SpectGetFilter.vi"("error in"=w943, "Filter Wheel Number"=i16 1, "Spectrometer Handle"=w944) -> ("error out"=w937:errorcluster, "Filter Number"=w939:i16, "Spectrometer Handle"=w938:u32)
                n616 = local write "Mono handle"(w938) -> ()
                n617 = local write "Filter Wheel Position"(w939) -> ()
                n618 = local write "MonoError"(w937) -> ()
              }
              frame #2 {
              }
            }
          }
          frame 21 {
            # "PLE start"
            # "Next step"
            # "Start"
            n619 = local read "Steps LLTF"() -> (w947:i32)
            n620 = local read "End Wavelength LLTF"() -> (w949:dbl)
            n621 = Decrement(x=w947) -> ()  [unwired: 1 out]
            n622 = local read "Start Wavelength LLTF"() -> (w951:dbl)
            n623 = Subtract(x=w949, y=w951) -> (x-y=w950:dbl)
            n624 = local read "LLTF error"() -> (w952:errorcluster)
            n625 = Divide(x=w950, y=w947) -> (x/y=w948:dbl)
            n626 = stacked-sequence {
              seq-local: [w953 _ _] -> [_ w1018 _]
              seq-local: [_ w1018 _] -> [_ _ w1019]
              tunnel: w948 -> [w961 _ _]
              tunnel: w951 -> [w956 _ _]
              tunnel: w952 -> [w958 _ _]
              tunnel: w947 -> [w960 _ _]
              frame #0 {
                n627 = flat-sequence {
                  tunnel: w958 -> [w972]
                  tunnel: [w971] -> w959
                  tunnel: w956 -> [w970]
                  tunnel: w959 -> [w974]
                  tunnel: [w974] -> w955
                  tunnel: [w977] -> w957
                  tunnel: w955 -> [w977]
                  frame #0 {
                    n628 = local read "LLTF handle"() -> (w973:u32)
                    n629 = call "PE Set Wavelength.vi"("error in (no error)"=w972, "wavelength"=w970, "peHandle"=w973) -> ("error out"=w971:errorcluster)  [unwired: 7 in, 1 out]
                  }
                  frame #1 {
                    n630 = Wait (ms)(milliseconds to wait=1000.0 ("y")) -> ()  [unwired: 1 out]
                  }
                  frame #2 {
                    n631 = Tick Count (ms)() -> (millisecond timer value=w976:u32)
                    n632 = local write "timestart"(w976) -> ()
                  }
                }
                n633 = while {
                  tunnel: w961 -> [w995]
                  shift-right: [w994] -> _
                  shift-left: w956 -> [w992]
                  tunnel: w960 -> [w979]
                  shift-right: [w986] -> w954
                  shift-left: w957 -> [w991]
                  i -> [w993]
                  stop <- w984 continue-if-true
                  n634 = Add(x=w992, y=w995) -> (x+y=w994:dbl)
                  n635 = Decrement(x=w979) -> (x-1=w978:i32)
                  n636 = local read "LLTF handle"() -> (w985:u32)
                  n637 = Greater?(x=w978, y=w993) -> (0:w981:bool)
                  n638 = local read "Stop Measurement"() -> (w983:bool)
                  n639 = call "PE Set Wavelength.vi"("error in (no error)"=w991, "wavelength"=w992, "peHandle"=w985) -> ("error out"=w990:errorcluster)  [unwired: 7 in, 1 out]
                  n640 = call "PE Get Wavelength.vi"("error in (no error)"=w990, "peHandle"=w985) -> ("error out"=w988:errorcluster, "wavelength"=w989:dbl)  [unwired: 7 in, 1 out]
                  n641 = local write "Wavelength LLTF (nm)"(w989) -> ()
                  n642 = case shown="False" FALSE {
                    tunnel: w988 -> [w1001 w1017]
                    tunnel: [w997 w1017] -> w986
                    tunnel: [w996 w1016] -> w980
                    tunnel: w981 -> [w996 w1016]
                    frame False {
                      n643 = local read "PL_Clock"() -> (w1000:bool)
                      n644 = local read "PiezoStage ON"() -> (w999:bool)
                      n645 = And(x=w1000, y=w999) -> (x .and. y?=w998:bool)
                      n646 = case shown="True" w998 {
                        tunnel: w1001 -> [w1002 w1008]
                        tunnel: [w1002 w1008] -> w997
                        frame False {
                          n647 = local read "Step delay LLTF"() -> (w1004:dbl)
                          n648 = Multiply(x=w1004, y=1000.0) -> (x*y=w1005:dbl)
                          n649 = Wait (ms)(milliseconds to wait=w1005) -> ()  [unwired: 1 out]
                        }
                        frame True {
                          n650 = flat-sequence {
                            tunnel: [w1009] -> w1006
                            tunnel: [w1011] -> w1007
                            tunnel: w1006 -> [w1011]
                            tunnel: w1007 -> [w1015]
                            frame #0 {
                              n651 = local read "Piezohandle"() -> (w1010:i32)
                              n652 = dll-call lib="C:/LabView_Projects/LifeEye/32bitDLLs/Madlib.dll" fn="MCL_PixelClock"("handle"=w1010) -> ("handle"=w1009:i32)  [unwired: 4 in, 2 out]
                            }
                            frame #1 {
                              n653 = local read "Step delay LLTF"() -> (w1012:dbl)
                              n654 = Multiply(x=w1012, y=1000.0) -> (x*y=w1014:dbl)
                              n655 = Wait (ms)(milliseconds to wait=w1014) -> ()  [unwired: 1 out]
                            }
                            frame #2 {
                              n656 = dll-call lib="C:/LabView_Projects/LifeEye/32bitDLLs/Madlib.dll" fn="MCL_LineClock"("handle"=w1015) -> ()  [unwired: 5 in, 2 out]
                            }
                          }
                        }
                      }
                    }
                    frame True {
                    }
                  }
                  n657 = Not(x=w983) -> (.not. x?=w982:bool)
                  n658 = And(x=w980, y=w982) -> (x .and. y?=w984:bool)
                }
                n659 = flat-sequence {
                  tunnel: w954 -> [w969]
                  tunnel: [w969] -> w953
                  frame #0 {
                    n660 = local read "Steps LLTF"() -> (w963:i32)
                    n661 = local read "timestart"() -> (w967:i64)
                    n662 = Tick Count (ms)() -> (millisecond timer value=w968:u32)
                    n663 = Subtract(x=w968, y=w967) -> (x-y=w966:i64)
                    n664 = Divide(x=w966, y=u32 1000) -> (x/y=w964:dbl)
                    n665 = Divide(x=w964, y=w963) -> (x/y=w962:dbl)
                    n666 = local write "Real Delay (seconds/step)"(w962) -> ()
                  }
                }
              }
              frame #1 {
              }
              frame #2 {
                n667 = local write "LLTF error"(w1019) -> ()
              }
            }
          }
          frame 22 {
            # "PLmap start"
            n668 = flat-sequence {
              tunnel: [w1041] -> w1021
              tunnel: [w1040] -> w1020
              tunnel: w1021 -> [w1145]
              tunnel: w1020 -> [w1144]
              frame #0 {
                n669 = local read "Mono handle"() -> (w1024:u32)
                n670 = local read "Steps LLTF"() -> (w1023:i32)
                n671 = local read "MonoError"() -> (w1025:errorcluster)
                n672 = local read "StepsDet"() -> (w1022:i32)
                n673 = local read "End Wavelength (nm)"() -> (w1042:dbl)
                n674 = local read "End Wavelength LLTF"() -> (w1044:dbl)
                n675 = Decrement(x=w1022) -> ()  [unwired: 1 out]
                n676 = Decrement(x=w1023) -> ()  [unwired: 1 out]
                n677 = local read "Start Wavelength LLTF"() -> (w1036:dbl)
                n678 = local read "Start Wavelength (nm)"() -> (w1043:dbl)
                n679 = call "SpectSetFilter.vi"("Filter Number"=i16 6 ("Filter Wheel Number"), "error in"=w1025, "Filter Wheel Number"=i16 1, "Spectrometer Handle"=w1024) -> ("error out"=w1034:errorcluster, "Spectrometer Handle"=w1035:u32)
                n680 = Subtract(x=w1044, y=w1036) -> (x-y=w1046:dbl)
                n681 = Subtract(x=w1042, y=w1043) -> (x-y=w1045:dbl)
                n682 = call "ExSubWaitSpec.vi"("error in (no error)"=w1034, "Spectrometer Handle"=w1035) -> ("error out"=w1032:errorcluster, "Spectrometer handle"=w1033:u32)
                n683 = Divide(x=w1046, y=w1023) -> (x/y=w1037:dbl)
                n684 = Divide(x=w1045, y=w1022) -> (x/y=w1038:dbl)
                n685 = local read "LLTF error"() -> (w1039:errorcluster)
                n686 = call "SpectGetFilter.vi"("error in"=w1032, "Filter Wheel Number"=i16 1, "Spectrometer Handle"=w1033) -> ("error out"=w1028:errorcluster, "Filter Number"=w1027:i16, "Spectrometer Handle"=w1026:u32)
                n687 = local write "Filter Wheel Position"(w1027) -> ()
                n688 = while {
                  shift-right: [w1083] -> _
                  shift-left: w1043 -> [w1057]
                  tunnel: [w1084] -> _
                  shift-right: [w1075] -> w1041
                  shift-left: w1026 -> [w1059]
                  shift-right: [w1065] -> w1040
                  shift-left: w1028 -> [w1058]
                  shift-right: [w1074] -> _
                  shift-left: w1039 -> [w1070]
                  tunnel: w1038 -> [w1073]
                  tunnel: w1022 -> [w1049]
                  tunnel: w1037 -> [w1072]
                  tunnel: w1036 -> [w1069]
                  tunnel: w1023 -> [w1071]
                  i -> [w1077]
                  stop <- w1047 continue-if-true
                  n689 = Decrement(x=w1049) -> ()  [unwired: 1 out]
                  n690 = local read "LLTF handle"() -> (w1060:u32)
                  n691 = local write "Wavelength (nm)"(w1057) -> ()
                  n692 = Add(x=w1057, y=w1073) -> (x+y=w1083:dbl)
                  n693 = call "SpectSetWavelength.vi"("error in"=w1058, "Wavelength"=w1057, "Spectrometer Handle"=w1059) -> ("error out"=w1055:errorcluster, "Spectrumeter Handle"=w1056:u32)
                  n694 = Equal?(x=0, y=w1077) -> (x = y?=w1076:bool)
                  n695 = local read "Stop Measurement"() -> (w1079:bool)
                  n696 = call "PE Set Wavelength.vi"("error in (no error)"=w1070, "wavelength"=w1069, "peHandle"=w1060) -> ("error out"=w1064:errorcluster)  [unwired: 7 in, 1 out]
                  n697 = call "ExSubWaitSpec.vi"("error in (no error)"=w1055, "Spectrometer Handle"=w1056) -> ("error out"=w1053:errorcluster, "Spectrometer handle"=w1054:u32)
                  n698 = call "SpectGetGratingInfo.vi"("Spectrometer Handle"=w1054, "error in"=w1053) -> ("Current Wavelength"=w1052:dbl, "Spectrometer Handle"=w1051:u32, "error out"=w1050:errorcluster)  [unwired: 3 out]
                  n699 = local write "Wavelength (nm)"(w1052) -> ()
                  n700 = case shown="True" w1076 {
                    tunnel: [w1092 w1097] -> w1068
                    tunnel: [w1091 w1096] -> w1067
                    tunnel: w1051 -> [w1092 w1094]
                    tunnel: w1050 -> [w1091 w1093]
                    frame False {
                    }
                    frame True {
                      n701 = call "SpectSetFilter.vi"("Filter Number"=i16 1 ("Filter Wheel Number"), "error in"=w1093, "Filter Wheel Number"=i16 1, "Spectrometer Handle"=w1094) -> ("error out"=w1103:errorcluster, "Spectrometer Handle"=w1104:u32)
                      n702 = call "ExSubWaitSpec.vi"("error in (no error)"=w1103, "Spectrometer Handle"=w1104) -> ("error out"=w1101:errorcluster, "Spectrometer handle"=w1102:u32)
                      n703 = call "SpectGetFilter.vi"("error in"=w1101, "Filter Wheel Number"=i16 1, "Spectrometer Handle"=w1102) -> ("error out"=w1096:errorcluster, "Filter Number"=w1095:i16, "Spectrometer Handle"=w1097:u32)
                      n704 = local write "Filter Wheel Position"(w1095) -> ()
                    }
                  }
                  n705 = flat-sequence {
                    tunnel: [w1090] -> w1063
                    tunnel: w1064 -> [w1090]
                    tunnel: w1067 -> [w1088]
                    tunnel: [w1088] -> w1066
                    frame #0 {
                      n706 = Wait (ms)(milliseconds to wait=u32 50) -> ()  [unwired: 1 out]
                    }
                  }
                  n707 = Greater?(x=w1049, y=w1077) -> (0:w1082:bool)
                  n708 = call "PE Get Wavelength.vi"("error in (no error)"=w1063, "peHandle"=w1060) -> ("error out"=w1062:errorcluster, "wavelength"=w1061:dbl)  [unwired: 7 in, 1 out]
                  n709 = while {
                    shift-right: [w1120] -> w1084
                    shift-left: w1069 -> [w1119]
                    shift-right: [w1126] -> w1081
                    shift-left: w1082 -> [w1126]
                    shift-right: [w1129] -> w1075
                    shift-left: w1068 -> [w1129]
                    shift-right: [w1128] -> w1065
                    shift-left: w1066 -> [w1128]
                    shift-right: [w1106] -> w1074
                    shift-left: w1062 -> [w1122]
                    tunnel: w1072 -> [w1121]
                    tunnel: w1071 -> [w1105]
                    i -> [w1114]
                    stop <- w1110 continue-if-true
                    n710 = Decrement(x=w1105) -> ()  [unwired: 1 out]
                    n711 = local read "LLTF handle"() -> (w1124:u32)
                    n712 = local read "PL_Clock"() -> (w1118:bool)
                    n713 = local read "Stop Measurement"() -> (w1130:bool)
                    n714 = Add(x=w1119, y=w1121) -> (x+y=w1120:dbl)
                    n715 = local read "PiezoStage ON"() -> (w1117:bool)
                    n716 = call "PE Set Wavelength.vi"("error in (no error)"=w1122, "wavelength"=w1119, "peHandle"=w1124) -> ("error out"=w1123:errorcluster)  [unwired: 7 in, 1 out]
                    n717 = Greater?(x=w1105, y=w1114) -> (0:w1127:bool)
                    n718 = And(x=w1117, y=w1118) -> (x .and. y?=w1115:bool)
                    n719 = Not(x=w1130) -> (.not. x?=w1131:bool)
                    n720 = call "PE Get Wavelength.vi"("error in (no error)"=w1123, "peHandle"=w1124) -> ("error out"=w1109:errorcluster, "wavelength"=w1125:dbl)  [unwired: 7 in, 1 out]
                    n721 = Equal?(x=w1114, y=0) -> (x = y?=w1112:bool)
                    n722 = local write "Wavelength LLTF (nm)"(w1125) -> ()
                    n723 = And(x=w1127, y=w1131) -> (x .and. y?=w1111:bool)
                    n724 = And(x=w1115, y=w1112) -> (x .and. y?=w1116:bool)
                    n725 = case shown="True" w1116 {
                      tunnel: w1109 -> [w1137 w1138]
                      tunnel: [w1137 w1138] -> w1108
                      frame False {
                      }
                      frame True {
                        n726 = local read "Piezohandle"() -> (w1139:i32)
                        n727 = dll-call lib="C:/LabView_Projects/LifeEye/32bitDLLs/Madlib.dll" fn="MCL_PixelClock"("handle"=w1139) -> ()  [unwired: 5 in, 2 out]
                      }
                    }
                    n728 = flat-sequence {
                      tunnel: [w1140] -> w1107
                      tunnel: w1108 -> [w1140]
                      frame #0 {
                        n729 = local read "Step delay LLTF"() -> (w1141:dbl)
                        n730 = Multiply(x=w1141, y=1000.0) -> (x*y=w1143:dbl)
                        n731 = Wait (ms)(milliseconds to wait=w1143) -> ()  [unwired: 1 out]
                      }
                    }
                    n732 = case shown="False" w1111 {
                      selector: w1111 -> [w1133 w1136]
                      tunnel: [w1133 w1136] -> w1110
                      tunnel: w1107 -> [w1132 w1135]
                      tunnel: [w1132 w1135] -> w1106
                      frame False {
                        n733 = local read "Piezohandle"() -> (w1134:i32)
                        n734 = dll-call lib="C:/LabView_Projects/LifeEye/32bitDLLs/Madlib.dll" fn="MCL_LineClock"("handle"=w1134) -> ()  [unwired: 5 in, 2 out]
                      }
                      frame True {
                      }
                    }
                  }
                  n735 = local write "Wavelength LLTF (nm)"(w1061) -> ()
                  n736 = Not(x=w1079) -> (.not. x?=w1080:bool)
                  n737 = And(x=w1080, y=w1081) -> (x .and. y?=w1048:bool)
                  n738 = case shown="True" w1048 {
                    selector: w1048 -> [w1085 w1087]
                    tunnel: [w1085 w1087] -> w1047
                    frame False {
                      n739 = local read "Piezohandle"() -> (w1086:i32)
                      n740 = dll-call lib="C:/LabView_Projects/LifeEye/32bitDLLs/Madlib.dll" fn="MCL_FrameClock"("handle"=w1086) -> ()  [unwired: 5 in, 2 out]
                    }
                    frame True {
                    }
                  }
                }
              }
              frame #1 {
                n741 = call "SpectSetFilter.vi"("Filter Number"=i16 6 ("Filter Wheel Number"), "error in"=w1144, "Filter Wheel Number"=i16 1, "Spectrometer Handle"=w1145) -> ("error out"=w1154:errorcluster, "Spectrometer Handle"=w1155:u32)
                n742 = call "ExSubWaitSpec.vi"("error in (no error)"=w1154, "Spectrometer Handle"=w1155) -> ("error out"=w1152:errorcluster, "Spectrometer handle"=w1153:u32)
                n743 = call "SpectGetFilter.vi"("error in"=w1152, "Filter Wheel Number"=i16 1, "Spectrometer Handle"=w1153) -> ("error out"=w1148:errorcluster, "Filter Number"=w1147:i16, "Spectrometer Handle"=w1146:u32)
                n744 = local write "Mono handle"(w1146) -> ()
                n745 = local write "Filter Wheel Position"(w1147) -> ()
                n746 = local write "MonoError"(w1148) -> ()
              }
              frame #2 {
              }
            }
          }
          frame 23 {
            n747 = flat-sequence {
              frame #0 {
                # "stepY"
                # "rangeY"
                # "stepX"
                # "startW"
                # "startX"
                # "rangeW"
                # "rangeX"
                n748 = local read "StartY (µm)"() -> (w1164:dbl)
                n749 = local read "StartX (µm)"() -> (w1165:dbl)
                n750 = local read "Steps LLTF"() -> (w1161:i32)
                n751 = local read "EndX (µm)"() -> (w1167:dbl)
                n752 = local read "EndY (µm)"() -> (w1166:dbl)
                n753 = local read "End Wavelength LLTF"() -> (w1171:dbl)
                n754 = Decrement(x=w1161) -> ()  [unwired: 1 out]
                n755 = Subtract(x=w1167, y=w1165) -> (x-y=w1163:dbl)
                n756 = Subtract(x=w1166, y=w1164) -> (x-y=w1162:dbl)
                n757 = local read "Start Wavelength LLTF"() -> (w1168:dbl)
                n758 = case shown="False" "2D Hyperspectral" {
                  tunnel: w1163 -> [w1177 w1187]
                  tunnel: w1162 -> [w1175 w1186]
                  tunnel: [w1176 w1185] -> w1160
                  tunnel: [w1173 w1184] -> w1159
                  tunnel: [w1172 w1178] -> w1158
                  tunnel: [_ w1180] -> w1157
                  frame False {
                    n759 = local read "Number of Spectra"() -> (w1172:i16)
                    n760 = Decrement(x=w1172) -> (x-1=w1174:i16)
                    n761 = Divide(x=w1177, y=w1174) -> (x/y=w1176:dbl)
                    n762 = Divide(x=w1175, y=w1174) -> (x/y=w1173:dbl)
                  }
                  frame True {
                    n763 = local read "StepX (µm)"() -> (w1185:dbl)
                    n764 = local read "StepY (µm)"() -> (w1184:dbl)
                    n765 = Divide(x=w1187, y=w1185) -> (x/y=w1183:dbl)
                    n766 = Divide(x=w1186, y=w1184) -> (x/y=w1182:dbl)
                    n767 = To Long Integer(number=w1183) -> (32bit integer=w1179:i32)
                    n768 = To Long Integer(number=w1182) -> (32bit integer=w1181:i32)
                    n769 = Increment(x=w1179) -> (x+1=w1178:i32)
                    n770 = Increment(x=w1181) -> (x+1=w1180:i32)
                  }
                }
                n771 = Subtract(x=w1171, y=w1168) -> (x-y=w1170:dbl)
                n772 = Divide(x=w1170, y=w1161) -> (x/y=w1169:dbl)
                n773 = while {
                  tunnel: w1160 -> [w1215]
                  tunnel: w1169 -> [w1218]
                  shift-right: [w1217] -> _
                  shift-left: w1168 -> [w1216]
                  tunnel: w1158 -> [w1214]
                  tunnel: w1161 -> [w1192]
                  tunnel: w1165 -> [w1213]
                  tunnel: w1164 -> [w1196]
                  tunnel: w1159 -> [w1197]
                  tunnel: w1157 -> [w1188]
                  tunnel: "2D Hyperspectral" -> [w1189]
                  i -> [w1206]
                  stop <- w1190 continue-if-true
                  n774 = Decrement(x=w1192) -> ()  [unwired: 1 out]
                  n775 = Greater?(x=w1192, y=w1206) -> (0:w1208:bool)
                  n776 = Add(x=w1218, y=w1216) -> (x+y=w1217:dbl)
                  n777 = local read "Stop Measurement"() -> (w1209:bool)
                  n778 = Equal?(x=0, y=w1206) -> (x = y?=w1204:bool)
                  n779 = flat-sequence {
                    tunnel: w1216 -> [w1363]
                    tunnel: w1204 -> [w1362]
                    tunnel: [w1362] -> w1202
                    tunnel: [w1361] -> w1198
                    tunnel: w1213 -> [w1366]
                    tunnel: [w1366] -> w1212
                    tunnel: [w1371] -> w1203
                    tunnel: w1202 -> [w1371]
                    tunnel: [w1370] -> w1199
                    tunnel: w1198 -> [w1370]
                    tunnel: w1196 -> [w1364]
                    tunnel: [w1364] -> w1194
                    tunnel: w1212 -> [w1376]
                    tunnel: w1203 -> [w1374]
                    tunnel: [w1376] -> w1201
                    tunnel: [w1373] -> w1200
                    tunnel: w1199 -> [w1373]
                    tunnel: [w1372] -> w1195
                    tunnel: w1194 -> [w1372]
                    tunnel: [w1382] -> w1211
                    tunnel: w1201 -> [w1382]
                    tunnel: w1200 -> [w1381]
                    tunnel: [w1379] -> w1193
                    tunnel: w1195 -> [w1379]
                    frame #0 {
                      n780 = local read "LLTF handle"() -> (w1361:u32)
                      n781 = call "PE Set Wavelength.vi"("wavelength"=w1363, "peHandle"=w1361) -> ()  [unwired: 8 in, 2 out]
                    }
                    frame #1 {
                      n782 = local read "Piezohandle"() -> (w1369:i32)
                      n783 = dll-call lib="C:/LabView_Projects/LifeEye/32bitDLLs/Madlib.dll" fn="MCL_SingleWriteN"("position"=w1366, "axis"=u32 1, "handle"=w1369) -> ("handle"=w1368:i32)  [unwired: 5 in, 3 out]
                      n784 = dll-call lib="C:/LabView_Projects/LifeEye/32bitDLLs/Madlib.dll" fn="MCL_SingleWriteN"("position"=w1364, "axis"=u32 2, "handle"=w1368) -> ()  [unwired: 6 in, 3 out]
                    }
                    frame #2 {
                      n785 = case shown="False" w1374 {
                        tunnel: [u32 50 ("milliseconds to wait") u32 1000 ("milliseconds to wait")] -> w1375
                        frame False {
                        }
                        frame True {
                        }
                      }
                      n786 = Wait (ms)(milliseconds to wait=w1375) -> ()  [unwired: 1 out]
                    }
                    frame #3 {
                      n787 = call "PE Get Wavelength.vi"("peHandle"=w1381) -> ("wavelength"=w1380:dbl)  [unwired: 8 in, 2 out]
                      n788 = local write "Wavelength LLTF (nm)"(w1380) -> ()
                    }
                  }
                  n789 = case shown="True" w1189 {
                    tunnel: w1215 -> [w1226 w1301]
                    tunnel: w1214 -> [w1225 w1300]
                    tunnel: w1211 -> [w1224 w1299]
                    tunnel: w1208 -> [w1223 w1298]
                    tunnel: [w1222 w1297] -> w1207
                    tunnel: w1197 -> [w1221 w1296]
                    tunnel: w1193 -> [w1220 w1295]
                    tunnel: w1188 -> [w1219 _]
                    frame True {
                      n790 = flat-sequence {
                        tunnel: w1226 -> [w1235]
                        tunnel: w1225 -> [w1234]
                        tunnel: w1224 -> [w1233]
                        tunnel: w1223 -> [w1232]
                        tunnel: [w1232] -> w1222
                        tunnel: w1221 -> [w1231]
                        tunnel: w1220 -> [w1230]
                        tunnel: w1219 -> [w1229]
                        frame #0 {
                          n791 = local read "Piezohandle"() -> (w1228:i32)
                          n792 = dll-call lib="C:/LabView_Projects/LifeEye/32bitDLLs/Madlib.dll" fn="MCL_PixelClock"("handle"=w1228) -> ("handle"=w1227:i32)  [unwired: 4 in, 2 out]
                          n793 = while {
                            tunnel: w1235 -> [w1252]
                            tunnel: w1234 -> [w1251]
                            tunnel: w1233 -> [w1250]
                            tunnel: w1231 -> [w1243]
                            tunnel: w1227 -> [w1240]
                            shift-right: [w1241] -> _
                            shift-left: w1230 -> [w1242]
                            tunnel: w1229 -> [w1236]
                            i -> [w1246]
                            stop <- w1249 continue-if-true
                            n794 = Add(x=w1242, y=w1243) -> (x+y=w1241:dbl)
                            n795 = Decrement(x=w1236) -> (x-1=w1245:i32)
                            n796 = dll-call lib="C:/LabView_Projects/LifeEye/32bitDLLs/Madlib.dll" fn="MCL_SingleWriteN"("position"=w1242, "axis"=u32 2, "handle"=w1240) -> ()  [unwired: 6 in, 3 out]
                            n797 = Greater?(x=w1245, y=w1246) -> (0:w1239:bool)
                            n798 = while {
                              shift-right: [w1274] -> _
                              shift-left: w1250 -> [w1266]
                              tunnel: w1252 -> [w1273]
                              tunnel: w1251 -> [w1261]
                              tunnel: w1240 -> [w1260]
                              tunnel: [w1259] -> w1248
                              tunnel: [w1257] -> w1247
                              tunnel: w1239 -> [w1256]
                              tunnel: [w1256] -> w1238
                              i -> [w1272]
                              stop <- w1270 continue-if-true
                              n799 = Decrement(x=w1261) -> ()  [unwired: 1 out]
                              n800 = Add(x=w1273, y=w1266) -> (x+y=w1274:dbl)
                              n801 = Greater?(x=w1261, y=w1272) -> (0:w1262:bool)
                              n802 = flat-sequence {
                                tunnel: w1260 -> [w1276]
                                tunnel: [w1275] -> w1267
                                tunnel: w1266 -> [w1277]
                                tunnel: [w1279] -> w1263
                                tunnel: w1262 -> [w1279]
                                tunnel: [w1281] -> w1268
                                tunnel: w1267 -> [w1281]
                                tunnel: [w1280] -> w1264
                                tunnel: w1263 -> [w1280]
                                tunnel: [w1286] -> w1269
                                tunnel: w1268 -> [w1286]
                                tunnel: [w1282] -> w1265
                                tunnel: w1264 -> [w1282]
                                tunnel: w1269 -> [w1287]
                                tunnel: [w1294] -> w1258
                                tunnel: w1265 -> [w1294]
                                tunnel: [w1289] -> w1257
                                frame #0 {
                                n803 = dll-call lib="C:/LabView_Projects/LifeEye/32bitDLLs/Madlib.dll" fn="MCL_SingleWriteN"("position"=w1277, "axis"=u32 1, "handle"=w1276) -> ("handle"=w1275:i32)  [unwired: 5 in, 3 out]
                                }
                                frame #1 {
                                }
                                frame #2 {
                                n804 = local read "Pixel Delay (s)"() -> (w1283:dbl)
                                n805 = Multiply(x=w1283, y=1000.0) -> (x*y=w1285:dbl)
                                n806 = Wait (ms)(milliseconds to wait=w1285) -> ()  [unwired: 1 out]
                                }
                                frame #3 {
                                n807 = dll-call lib="C:/LabView_Projects/LifeEye/32bitDLLs/Madlib.dll" fn="MCL_SingleReadN"("axis"=u32 1, "handle"=w1287) -> ("position"=w1293:dbl, "handle"=w1288:i32)  [unwired: 4 in, 2 out]
                                n808 = local write "xRead"(w1293) -> ()
                                n809 = dll-call lib="C:/LabView_Projects/LifeEye/32bitDLLs/Madlib.dll" fn="MCL_SingleReadN"("axis"=u32 2, "handle"=w1288) -> ("position"=w1290:dbl, "handle"=w1289:i32)  [unwired: 4 in, 2 out]
                                n810 = local write "yRead"(w1290) -> ()
                                }
                              }
                              n811 = local read "Stop Measurement"() -> (w1271:bool)
                              n812 = Not(x=w1271) -> (.not. x?=w1259:bool)
                              n813 = And(x=w1258, y=w1259) -> (x .and. y?=w1270:bool)
                            }
                            n814 = case shown="False" w1238 {
                              selector: w1238 -> [w1254 w1255]
                              tunnel: [w1254 w1255] -> w1237
                              tunnel: w1247 -> [w1253 _]
                              frame False {
                                n815 = dll-call lib="C:/LabView_Projects/LifeEye/32bitDLLs/Madlib.dll" fn="MCL_LineClock"("handle"=w1253) -> ()  [unwired: 5 in, 2 out]
                              }
                              frame True {
                              }
                            }
                            n816 = And(x=w1237, y=w1248) -> (x .and. y?=w1249:bool)
                          }
                        }
                      }
                    }
                    frame False {
                      n817 = flat-sequence {
                        tunnel: w1301 -> [w1309]
                        tunnel: w1300 -> [w1308]
                        tunnel: w1299 -> [w1307]
                        tunnel: w1298 -> [w1306]
                        tunnel: [w1306] -> w1297
                        tunnel: w1296 -> [w1305]
                        tunnel: w1295 -> [w1304]
                        frame #0 {
                          n818 = local read "Piezohandle"() -> (w1303:i32)
                          n819 = dll-call lib="C:/LabView_Projects/LifeEye/32bitDLLs/Madlib.dll" fn="MCL_PixelClock"("handle"=w1303) -> ("handle"=w1302:i32)  [unwired: 4 in, 2 out]
                          n820 = while {
                            shift-right: [w1331] -> _
                            shift-left: w1307 -> [w1322]
                            tunnel: w1309 -> [w1330]
                            tunnel: w1308 -> [w1311]
                            tunnel: w1305 -> [w1314]
                            shift-right: [w1312] -> _
                            shift-left: w1304 -> [w1313]
                            tunnel: w1302 -> [w1310]
                            i -> [w1329]
                            stop <- w1326 continue-if-true
                            n821 = Decrement(x=w1311) -> ()  [unwired: 1 out]
                            n822 = Add(x=w1330, y=w1322) -> (x+y=w1331:dbl)
                            n823 = Add(x=w1314, y=w1313) -> (x+y=w1312:dbl)
                            n824 = local read "Stop Measurement"() -> (w1328:bool)
                            n825 = Greater?(x=w1311, y=w1329) -> (0:w1318:bool)
                            n826 = flat-sequence {
                              tunnel: w1310 -> [w1335]
                              tunnel: [w1338] -> w1323
                              tunnel: w1322 -> [w1336]
                              tunnel: [w1342] -> w1319
                              tunnel: w1318 -> [w1342]
                              tunnel: w1313 -> [w1337]
                              tunnel: [w1344] -> w1324
                              tunnel: w1323 -> [w1344]
                              tunnel: [w1343] -> w1320
                              tunnel: w1319 -> [w1343]
                              tunnel: [w1349] -> w1325
                              tunnel: w1324 -> [w1349]
                              tunnel: [w1345] -> w1321
                              tunnel: w1320 -> [w1345]
                              tunnel: w1325 -> [w1350]
                              tunnel: [w1357] -> w1317
                              tunnel: w1321 -> [w1357]
                              tunnel: [w1352] -> w1315
                              frame #0 {
                                n827 = dll-call lib="C:/LabView_Projects/LifeEye/32bitDLLs/Madlib.dll" fn="MCL_SingleWriteN"("position"=w1336, "axis"=u32 1, "handle"=w1335) -> ("handle"=w1340:i32)  [unwired: 5 in, 3 out]
                                n828 = dll-call lib="C:/LabView_Projects/LifeEye/32bitDLLs/Madlib.dll" fn="MCL_SingleWriteN"("position"=w1337, "axis"=u32 2, "handle"=w1340) -> ("handle"=w1338:i32)  [unwired: 5 in, 3 out]
                              }
                              frame #1 {
                              }
                              frame #2 {
                                n829 = local read "Pixel Delay (s)"() -> (w1346:dbl)
                                n830 = Multiply(x=w1346, y=1000.0) -> (x*y=w1348:dbl)
                                n831 = Wait (ms)(milliseconds to wait=w1348) -> ()  [unwired: 1 out]
                              }
                              frame #3 {
                                n832 = dll-call lib="C:/LabView_Projects/LifeEye/32bitDLLs/Madlib.dll" fn="MCL_SingleReadN"("axis"=u32 1, "handle"=w1350) -> ("position"=w1356:dbl, "handle"=w1351:i32)  [unwired: 4 in, 2 out]
                                n833 = local write "xRead"(w1356) -> ()
                                n834 = dll-call lib="C:/LabView_Projects/LifeEye/32bitDLLs/Madlib.dll" fn="MCL_SingleReadN"("axis"=u32 2, "handle"=w1351) -> ("position"=w1353:dbl, "handle"=w1352:i32)  [unwired: 4 in, 2 out]
                                n835 = local write "yRead"(w1353) -> ()
                              }
                            }
                            n836 = case shown="False" w1317 {
                              selector: w1317 -> [w1333 w1334]
                              tunnel: [w1333 w1334] -> w1316
                              tunnel: w1315 -> [w1332 _]
                              frame False {
                                n837 = dll-call lib="C:/LabView_Projects/LifeEye/32bitDLLs/Madlib.dll" fn="MCL_LineClock"("handle"=w1332) -> ()  [unwired: 5 in, 2 out]
                              }
                              frame True {
                              }
                            }
                            n838 = Not(x=w1328) -> (.not. x?=w1327:bool)
                            n839 = And(x=w1316, y=w1327) -> (x .and. y?=w1326:bool)
                          }
                        }
                      }
                    }
                  }
                  n840 = Not(x=w1209) -> (.not. x?=w1210:bool)
                  n841 = And(x=w1207, y=w1210) -> (x .and. y?=w1191:bool)
                  n842 = case shown="True" w1191 {
                    selector: w1191 -> [w1358 w1360]
                    tunnel: [w1358 w1360] -> w1190
                    frame False {
                    }
                    frame True {
                      n843 = local read "Piezohandle"() -> (w1359:i32)
                      n844 = dll-call lib="C:/LabView_Projects/LifeEye/32bitDLLs/Madlib.dll" fn="MCL_LineClock"("handle"=w1359) -> ()  [unwired: 5 in, 2 out]
                    }
                  }
                }
              }
              frame #1 {
              }
            }
          }
          frame 27 {
            # "OMA V  aquire  start"
            n845 = flat-sequence {
              frame #0 {
                w1386 = u32 1 ("Turret Number")
                n846 = local read "OMA V exposure time"() -> (w1383:dbl)
                n847 = local read "OMA V aquire mode"() -> (w1384:T4)
                n848 = local read "OMA V error"() -> (w1398:errorcluster)
                n849 = local read "MonoError"() -> (w1401:errorcluster)
                n850 = case shown="\"OMA V mode PL external sync\"" w1384 {
                  tunnel: [w1413 w1414 w1415 w1416 w1417] -> w1394
                  tunnel: w1383 -> [w1413 w1414 w1415 w1416 w1417]
                  frame "OMA V mode Single spectrum", Default {
                  }
                  frame "OMA V mode Hyperspectral" {
                  }
                  frame "OMA V mode PLE map" {
                  }
                  frame "OMA V mode Hyperspectral 2D" {
                  }
                  frame "OMA V mode PL external sync" {
                  }
                }
                n851 = local read "OMA V Handles Out"() -> (w1396:T5)
                n852 = local read "Wavelength (nm)"() -> (w1402:dbl)
                n853 = local read "Grating Number"() -> (w1387:i16)
                n854 = local read "Mono Calibration Handle"() -> (w1404:u32)
                n855 = case shown="1, Default" w1387 {
                  tunnel: [w1931 w1939 w1947] -> w1408
                  frame 1, Default {
                    w1932 = 25.0  # Pixel Width (microns)
                    w1933 = 1.0  # Magnification
                    w1934 = 1.35  # Detector Angle (degrees)
                    w1935 = 30.3  # Inclusion Angle (degrees)
                    w1936 = 300.0  # Focal Length (mm)
                    w1937 = 0.0  # Slope Adjust
                    w1938 = -3.71785  # Center Offset
                    n856 = Bundle("Center Offset"=w1938, "Slope Adjust"=w1937, "Focal Length (mm)"=w1936, "Inclusion Angle (degrees)"=w1935, "Detector Angle (degrees)"=w1934, "Magnification"=w1933, "Pixel Width (microns)"=w1932) -> (w1931:T6)  [unwired: 1 in]
                  }
                  frame 2 {
                    w1940 = 25.0  # Pixel Width (microns)
                    w1941 = 1.0  # Magnification
                    w1942 = -2.77  # Detector Angle (degrees)
                    w1943 = 32.7  # Inclusion Angle (degrees)
                    w1944 = 295.6  # Focal Length (mm)
                    w1945 = -0.000221379  # Slope Adjust
                    w1946 = -0.047502  # Center Offset
                    n857 = Bundle("Center Offset"=w1946, "Slope Adjust"=w1945, "Focal Length (mm)"=w1944, "Inclusion Angle (degrees)"=w1943, "Detector Angle (degrees)"=w1942, "Magnification"=w1941, "Pixel Width (microns)"=w1940) -> (w1939:T6)  [unwired: 1 in]
                  }
                  frame 3 {
                    w1948 = 25.0  # Pixel Width (microns)
                    w1949 = 1.0  # Magnification
                    w1950 = -2.77  # Detector Angle (degrees)
                    w1951 = 31.85  # Inclusion Angle (degrees)
                    w1952 = 297.6  # Focal Length (mm)
                    w1953 = 0.000251338  # Slope Adjust
                    w1954 = -1.24655  # Center Offset
                    n858 = Bundle("Center Offset"=w1954, "Slope Adjust"=w1953, "Focal Length (mm)"=w1952, "Inclusion Angle (degrees)"=w1951, "Detector Angle (degrees)"=w1950, "Magnification"=w1949, "Pixel Width (microns)"=w1948) -> (w1947:T6)  [unwired: 1 in]
                  }
                }
                n859 = Unbundle(w1396) -> ("Camera Handle"=w1393:u32, "Image Handle"=w1390:u32)  [unwired: 3 out]
                n860 = call "CameraExperiment.vi"("Number of Accumulations"=u32 1, "Acquire / Focus Flag"=u32 1, "error in"=w1398, "Number of Images"=u32 1, "Exposure (sec)"=w1394, "Camera Handle"=w1393) -> ("error out"=w1392:errorcluster)  [unwired: 1 out]
                n861 = call "CalibSetAdjVals.vi"("Calibration Handle"=w1404, "Turret Number"=w1386, "Grating Number"=w1387, "error in"=w1401, "Spectrometer Calibration Parameters"=w1408) -> ("Calibration Handle"=w1385:u32, "error out"=w1409:errorcluster)
                n862 = call "CalibSetSpectInfo.vi"("Calibration Handle"=w1385, "Current Grating Number"=w1387, "Current Wavelength"=w1402, "error in"=w1409, "Current Turret Number"=w1386) -> ("Calibration Handle"=w1407:u32, "error out"=w1410:errorcluster)
                n863 = call "CalibGetCalibArray.vi"("error in"=w1410, "Array Size"=u32 1024, "Calibration Handle"=w1407) -> ("error out"=w1411:errorcluster, "Calibrated Array"=w1400:dbl[])  [unwired: 1 out]
                n864 = local write "OMA V Calibrated Array"(w1400) -> ()
                n865 = case shown="\"OMA V mode PL external sync\"" w1384 {
                  tunnel: w1400 -> [w1423 w1447 w1577 w1702 w1805]
                  tunnel: w1393 -> [w1422 w1467 w1589 w1704 w1824]
                  tunnel: w1392 -> [w1421 w1454 w1579 w1701 w1801]
                  tunnel: [w1420 w1465 w1587 w1703 w1822] -> w1391
                  tunnel: w1390 -> [w1419 w1466 w1588 w1700 w1825]
                  tunnel: [w1418 w1467 w1589 w1699 w1823] -> w1389
                  frame "OMA V mode Single spectrum", Default {
                    w1432 = 1  # Strip to pul out of frame
                    n866 = call "CameraStart.vi"("error in"=w1421, "Camera Handle"=w1422) -> ("error out"=w1427:errorcluster, "Camera Handle"=w1426:u32)
                    n867 = while {
                      tunnel: [w1439] -> w1431
                      tunnel: [w1440] -> w1430
                      tunnel: w1427 -> [w1434]
                      tunnel: w1426 -> [w1433]
                      stop <- w1436 stop-if-true
                      n868 = call "CameraCheckData.vi"("Camera Handle"=w1433, "error in"=w1434) -> ("Camera Handle"=w1440:u32, "Number Of Frames Available"=w1441:i32, "error out"=w1439:errorcluster)
                      n869 = Unbundle By Name(w1439) -> ("status"=w1438:bool)
                      n870 = Greater Than 0?(x=w1441) -> (x > 0?=w1437:bool)
                      n871 = Or(x=w1438, y=w1437) -> (x .or. y?=w1436:bool)
                      n872 = Wait (ms)(milliseconds to wait=u32 5) -> ()  [unwired: 1 out]
                    }
                    n873 = call "CameraGetData.vi"("error in"=w1431, "Data Handle"=w1419, "Camera Handle"=w1430) -> ("error out"=w1429:errorcluster, "Data Handle"=w1428:u32, "Camera Handle"=w1418:u32)
                    n874 = call "ImageGetLineF32.vi"("error in"=w1429, "Z Position"=w1432, "Y Position"=w1432, "Data Handle"=w1428) -> ("error out"=w1420:errorcluster, "Array F32"=w1425:sgl[])  [unwired: 1 out]
                    n875 = Bundle("Calibrated Array"=w1423, "Array F32"=w1425) -> (→"XY Graph OMA V":T2)  [unwired: 1 in]
                  }
                  frame "OMA V mode Hyperspectral" {
                    n876 = Index Array(array=w1447, index=1) -> (element=w1445:dbl)
                    n877 = Index Array(array=w1447, index=0) -> (element=w1443:dbl)
                    n878 = Index Array(array=w1447, index=1023) -> (element=w1460:dbl)
                    n879 = local read "StartY (µm)"() -> (w1468:dbl)
                    n880 = local read "StartX (µm)"() -> (w1469:dbl)
                    n881 = local read "EndX (µm)"() -> (w1475:dbl)
                    n882 = local read "EndY (µm)"() -> (w1474:dbl)
                    n883 = property on="OMA V Hyperspectral graph" class="IntGraph (strict)"("YScale.Offset"=0.0 ("Y Scale.Offset and Multiplier:Offset"), "YScale.Multiplier"=1.0 ("Y Scale.Offset and Multiplier:Multiplier"), "YScale.Precision"=u8 0 ("Y Scale.Display Format:Precision")) -> ()  [unwired: 2 in, 2 out]
                    n884 = Subtract(x=w1445, y=w1443) -> (x-y=w1444:dbl)
                    n885 = local read "Number of Spectra"() -> (w1450:i16)
                    n886 = Subtract(x=w1443, y=w1444) -> (x-y=w1442:dbl)
                    n887 = Subtract(x=w1460, y=w1443) -> (x-y=w1457:dbl)
                    n888 = Subtract(x=w1474, y=w1468) -> (x-y=w1472:dbl)
                    n889 = Subtract(x=w1475, y=w1469) -> (x-y=w1473:dbl)
                    n890 = Subtract(x=w1450, y=i16 1) -> (x-y=w1448:i16)
                    n891 = Divide(x=w1457, y=1023.0) -> (x/y=w1455:dbl)
                    n892 = Initialize Array(0.0 ("element"), w1450, 1024 ("dimension size")) -> (w1453:dbl[][])
                    n893 = Divide(x=w1472, y=w1448) -> (x/y=w1470:dbl)
                    n894 = Divide(x=w1473, y=w1448) -> (x/y=w1471:dbl)
                    n895 = while {
                      tunnel: w1471 -> [w1506]
                      tunnel: w1470 -> [w1504]
                      tunnel: w1450 -> [w1477]
                      shift-right: [w1502] -> _
                      shift-left: w1469 -> [w1507]
                      shift-right: [w1501] -> _
                      shift-left: w1468 -> [w1505]
                      tunnel: w1454 -> [w1497]
                      tunnel: w1467 -> [w1495]
                      tunnel: w1466 -> [w1492]
                      tunnel: [w1489] -> w1465
                      shift-right: [w1484] -> _
                      shift-left: w1453 -> [w1487]
                      i -> [w1488]
                      stop <- w1499 continue-if-true
                      n896 = Add(x=w1507, y=w1506) -> (x+y=w1502:dbl)
                      n897 = Add(x=w1505, y=w1504) -> (x+y=w1501:dbl)
                      n898 = Decrement(x=w1477) -> (x-1=w1476:i16)
                      n899 = local read "Piezohandle"() -> (w1503:i32)
                      n900 = Greater?(x=w1476, y=w1488) -> (0:w1483:bool)
                      n901 = local read "Stop Measurement"() -> (w1500:bool)
                      n902 = flat-sequence {
                        tunnel: w1507 -> [w1514]
                        tunnel: w1503 -> [w1513]
                        tunnel: [w1512] -> w1498
                        tunnel: w1497 -> [w1512]
                        tunnel: w1495 -> [w1511]
                        tunnel: [w1511] -> w1493
                        tunnel: w1492 -> [w1510]
                        tunnel: [w1510] -> w1490
                        tunnel: w1487 -> [w1509]
                        tunnel: [w1509] -> w1485
                        tunnel: w1483 -> [w1508]
                        tunnel: [w1508] -> w1481
                        tunnel: w1505 -> [w1523]
                        tunnel: w1503 -> [w1522]
                        tunnel: w1498 -> [w1521]
                        tunnel: [w1521] -> w1496
                        tunnel: [w1520] -> w1494
                        tunnel: w1493 -> [w1520]
                        tunnel: [w1519] -> w1491
                        tunnel: w1490 -> [w1519]
                        tunnel: [w1518] -> w1486
                        tunnel: w1485 -> [w1518]
                        tunnel: [w1517] -> w1482
                        tunnel: w1481 -> [w1517]
                        tunnel: [w1516] -> w1478
                        tunnel: w1496 -> [w1540]
                        tunnel: w1494 -> [w1539]
                        tunnel: w1491 -> [w1538]
                        tunnel: [w1537] -> w1489
                        tunnel: w1488 -> [w1533]
                        tunnel: w1486 -> [w1534]
                        tunnel: [w1531] -> w1484
                        tunnel: w1482 -> [w1536]
                        tunnel: [w1536] -> w1480
                        tunnel: w1478 -> [w1528]
                        frame #0 {
                          n903 = dll-call lib="C:/LabView_Projects/LifeEye/32bitDLLs/Madlib.dll" fn="MCL_SingleWriteN"("position"=w1514, "axis"=u32 1, "handle"=w1513) -> ()  [unwired: 6 in, 3 out]
                        }
                        frame #1 {
                          n904 = dll-call lib="C:/LabView_Projects/LifeEye/32bitDLLs/Madlib.dll" fn="MCL_SingleWriteN"("position"=w1523, "axis"=u32 2, "handle"=w1522) -> ("handle"=w1516:i32)  [unwired: 5 in, 3 out]
                        }
                        frame #2 {
                          w1547 = 1  # Strip to pul out of frame
                          n905 = call "CameraStart.vi"("error in"=w1540, "Camera Handle"=w1539) -> ("error out"=w1542:errorcluster, "Camera Handle"=w1541:u32)
                          n906 = dll-call lib="C:/LabView_Projects/LifeEye/32bitDLLs/Madlib.dll" fn="MCL_SingleReadN"("axis"=u32 1, "handle"=w1528) -> ("position"=w1526:dbl, "handle"=w1527:i32)  [unwired: 4 in, 2 out]
                          n907 = while {
                            tunnel: [w1554] -> w1546
                            tunnel: [w1555] -> w1545
                            tunnel: w1542 -> [w1549]
                            tunnel: w1541 -> [w1548]
                            stop <- w1551 stop-if-true
                            n908 = call "CameraCheckData.vi"("Camera Handle"=w1548, "error in"=w1549) -> ("Camera Handle"=w1555:u32, "Number Of Frames Available"=w1556:i32, "error out"=w1554:errorcluster)
                            n909 = Unbundle By Name(w1554) -> ("status"=w1553:bool)
                            n910 = Greater Than 0?(x=w1556) -> (x > 0?=w1552:bool)
                            n911 = Or(x=w1553, y=w1552) -> (x .or. y?=w1551:bool)
                            n912 = Wait (ms)(milliseconds to wait=u32 5) -> ()  [unwired: 1 out]
                          }
                          n913 = local write "xRead"(w1526) -> ()
                          n914 = dll-call lib="C:/LabView_Projects/LifeEye/32bitDLLs/Madlib.dll" fn="MCL_SingleReadN"("axis"=u32 2, "handle"=w1527) -> ("position"=w1525:dbl)  [unwired: 5 in, 2 out]
                          n915 = local write "yRead"(w1525) -> ()
                          n916 = call "CameraGetData.vi"("error in"=w1546, "Data Handle"=w1538, "Camera Handle"=w1545) -> ("error out"=w1544:errorcluster, "Data Handle"=w1543:u32)  [unwired: 1 out]
                          n917 = call "ImageGetLineF32.vi"("error in"=w1544, "Z Position"=w1547, "Y Position"=w1547, "Data Handle"=w1543) -> ("error out"=w1537:errorcluster, "Array F32"=w1532:sgl[])  [unwired: 1 out]
                          n918 = Replace Array Subset(array=w1534, new element=w1532, index (row)=w1533) -> (w1531:dbl[][])  [unwired: 1 in]
                          n919 = Transpose 2D Array(2D array=w1531) -> (transposed array=→"OMA V Hyperspectral graph":dbl[][])
                        }
                      }
                      n920 = Not(x=w1500) -> (.not. x?=w1479:bool)
                      n921 = And(x=w1480, y=w1479) -> (x .and. y?=w1499:bool)
                    }
                    n922 = property on="OMA V Hyperspectral graph" class="IntGraph (strict)"("XScale.Offset"=w1442, "XScale.Multiplier"=w1455, "XScale.Precision"=u8 1 ("X Scale.Display Format:Precision")) -> ()  [unwired: 2 in, 2 out]
                  }
                  frame "OMA V mode Hyperspectral 2D" {
                    n923 = Index Array(array=w1577, index=1) -> (element=w1575:dbl)
                    n924 = Index Array(array=w1577, index=0) -> (element=w1573:dbl)
                    n925 = Index Array(array=w1577, index=1023) -> (element=w1582:dbl)
                    n926 = local read "StartX (µm)"() -> (w1590:dbl)
                    n927 = local read "StartY (µm)"() -> (w1564:dbl)
                    n928 = local read "StepY (µm)"() -> (w1565:dbl)
                    n929 = local read "StepX (µm)"() -> (w1566:dbl)
                    n930 = local read "EndX (µm)"() -> (w1594:dbl)
                    n931 = local read "EndY (µm)"() -> (w1593:dbl)
                    n932 = property on="OMA V Hyperspectral graph" class="IntGraph (strict)"("YScale.Offset"=0.0 ("Y Scale.Offset and Multiplier:Offset"), "YScale.Multiplier"=1.0 ("Y Scale.Offset and Multiplier:Multiplier"), "YScale.Precision"=u8 0 ("Y Scale.Display Format:Precision")) -> ()  [unwired: 2 in, 2 out]
                    n933 = Subtract(x=w1575, y=w1573) -> (x-y=w1574:dbl)
                    n934 = Subtract(x=w1573, y=w1574) -> (x-y=w1572:dbl)
                    n935 = Subtract(x=w1582, y=w1573) -> (x-y=w1581:dbl)
                    n936 = Subtract(x=w1594, y=w1590) -> (x-y=w1592:dbl)
                    n937 = Subtract(x=w1593, y=w1564) -> (x-y=w1591:dbl)
                    n938 = Divide(x=w1592, y=w1566) -> (x/y=w1563:dbl)
                    n939 = Divide(x=w1591, y=w1565) -> (x/y=w1562:dbl)
                    n940 = Divide(x=w1581, y=1023.0) -> (x/y=w1571:dbl)
                    n941 = To Long Integer(number=w1563) -> (32bit integer=w1561:i32)
                    n942 = To Long Integer(number=w1562) -> (32bit integer=w1557:i32)
                    n943 = Increment(x=w1561) -> (x+1=w1560:i32)
                    n944 = Increment(x=w1557) -> (x+1=w1559:i32)
                    n945 = property on="OMA V Hyperspectral graph" class="IntGraph (strict)"("XScale.Offset"=w1572, "XScale.Multiplier"=w1571, "XScale.Precision"=u8 1 ("X Scale.Display Format:Precision")) -> ()  [unwired: 2 in, 2 out]
                    n946 = Multiply(x=w1560, y=w1559) -> (x*y=w1558:i32)
                    n947 = Initialize Array(0.0 ("element"), w1558, 1024 ("dimension size")) -> (w1578:dbl[][])
                    n948 = while {
                      tunnel: w1590 -> [w1614]
                      tunnel: w1589 -> [w1613]
                      tunnel: w1588 -> [w1612]
                      tunnel: w1566 -> [w1608]
                      tunnel: w1565 -> [w1605]
                      shift-right: [w1611] -> w1587
                      shift-left: w1579 -> [w1610]
                      shift-right: [w1604] -> _
                      shift-left: w1564 -> [w1601]
                      tunnel: w1561 -> [w1598]
                      tunnel: w1557 -> [w1597]
                      shift-right: [w1596] -> _
                      shift-left: w1578 -> [w1609]
                      i -> [w1595]
                      stop <- w1607 continue-if-true
                      n949 = Add(x=w1601, y=w1605) -> (x+y=w1604:dbl)
                      n950 = Greater?(x=w1597, y=w1595) -> (0:w1600:bool)
                      n951 = local read "Piezohandle"() -> (w1602:i32)
                      n952 = while {
                        tunnel: w1608 -> [w1647]
                        shift-right: [w1646] -> _
                        shift-left: w1614 -> [w1648]
                        tunnel: w1610 -> [w1642]
                        tunnel: w1613 -> [w1640]
                        tunnel: w1612 -> [w1637]
                        tunnel: [w1634] -> w1611
                        shift-right: [w1630] -> w1596
                        shift-left: w1609 -> [w1633]
                        tunnel: [w1625] -> w1606
                        tunnel: w1602 -> [w1624]
                        tunnel: w1600 -> [w1621]
                        tunnel: [w1621] -> w1599
                        tunnel: w1598 -> [w1616]
                        tunnel: w1595 -> [w1620]
                        i -> [w1618]
                        stop <- w1644 continue-if-true
                        n953 = Add(x=w1648, y=w1647) -> (x+y=w1646:dbl)
                        n954 = Increment(x=w1616) -> (x+1=w1615:i32)
                        n955 = Multiply(x=w1615, y=w1620) -> (x*y=w1619:i32)
                        n956 = Add(x=w1618, y=w1619) -> (x+y=w1617:i32)
                        n957 = Greater?(x=w1616, y=w1618) -> (0:w1629:bool)
                        n958 = local read "Stop Measurement"() -> (w1645:bool)
                        n959 = flat-sequence {
                          tunnel: w1648 -> [w1656]
                          tunnel: w1624 -> [w1655]
                          tunnel: [w1654] -> w1643
                          tunnel: w1642 -> [w1654]
                          tunnel: w1640 -> [w1653]
                          tunnel: [w1653] -> w1638
                          tunnel: w1637 -> [w1652]
                          tunnel: [w1652] -> w1635
                          tunnel: w1633 -> [w1651]
                          tunnel: [w1651] -> w1631
                          tunnel: w1629 -> [w1650]
                          tunnel: [w1650] -> w1627
                          tunnel: [w1649] -> w1622
                          tunnel: w1643 -> [w1663]
                          tunnel: [w1663] -> w1641
                          tunnel: [w1662] -> w1639
                          tunnel: w1638 -> [w1662]
                          tunnel: [w1661] -> w1636
                          tunnel: w1635 -> [w1661]
                          tunnel: [w1660] -> w1632
                          tunnel: w1631 -> [w1660]
                          tunnel: [w1659] -> w1628
                          tunnel: w1627 -> [w1659]
                          tunnel: [w1658] -> w1623
                          tunnel: w1622 -> [w1658]
                          tunnel: w1641 -> [w1679]
                          tunnel: w1639 -> [w1678]
                          tunnel: w1636 -> [w1677]
                          tunnel: [w1676] -> w1634
                          tunnel: w1617 -> [w1673]
                          tunnel: w1632 -> [w1674]
                          tunnel: [w1671] -> w1630
                          tunnel: w1628 -> [w1675]
                          tunnel: [w1675] -> w1626
                          tunnel: w1623 -> [w1664]
                          frame #0 {
                            n960 = dll-call lib="C:/LabView_Projects/LifeEye/32bitDLLs/Madlib.dll" fn="MCL_SingleWriteN"("position"=w1656, "axis"=u32 1, "handle"=w1655) -> ("handle"=w1649:i32)  [unwired: 5 in, 3 out]
                          }
                          frame #1 {
                          }
                          frame #2 {
                            w1686 = 1  # Strip to pul out of frame
                            n961 = call "CameraStart.vi"("error in"=w1679, "Camera Handle"=w1678) -> ("error out"=w1681:errorcluster, "Camera Handle"=w1680:u32)
                            n962 = dll-call lib="C:/LabView_Projects/LifeEye/32bitDLLs/Madlib.dll" fn="MCL_SingleReadN"("axis"=u32 1, "handle"=w1664) -> ("position"=w1667:dbl, "handle"=w1668:i32)  [unwired: 4 in, 2 out]
                            n963 = while {
                              tunnel: [w1693] -> w1685
                              tunnel: [w1694] -> w1684
                              tunnel: w1681 -> [w1688]
                              tunnel: w1680 -> [w1687]
                              stop <- w1690 stop-if-true
                              n964 = call "CameraCheckData.vi"("Camera Handle"=w1687, "error in"=w1688) -> ("Camera Handle"=w1694:u32, "Number Of Frames Available"=w1695:i32, "error out"=w1693:errorcluster)
                              n965 = Unbundle By Name(w1693) -> ("status"=w1692:bool)
                              n966 = Greater Than 0?(x=w1695) -> (x > 0?=w1691:bool)
                              n967 = Or(x=w1692, y=w1691) -> (x .or. y?=w1690:bool)
                              n968 = Wait (ms)(milliseconds to wait=u32 5) -> ()  [unwired: 1 out]
                            }
                            n969 = local write "xRead"(w1667) -> ()
                            n970 = dll-call lib="C:/LabView_Projects/LifeEye/32bitDLLs/Madlib.dll" fn="MCL_SingleReadN"("axis"=u32 2, "handle"=w1668) -> ("position"=w1666:dbl)  [unwired: 5 in, 2 out]
                            n971 = local write "yRead"(w1666) -> ()
                            n972 = call "CameraGetData.vi"("error in"=w1685, "Data Handle"=w1677, "Camera Handle"=w1684) -> ("error out"=w1683:errorcluster, "Data Handle"=w1682:u32)  [unwired: 1 out]
                            n973 = call "ImageGetLineF32.vi"("error in"=w1683, "Z Position"=w1686, "Y Position"=w1686, "Data Handle"=w1682) -> ("error out"=w1676:errorcluster, "Array F32"=w1672:sgl[])  [unwired: 1 out]
                            n974 = Replace Array Subset(array=w1674, new element=w1672, index (row)=w1673) -> (w1671:dbl[][])  [unwired: 1 in]
                            n975 = Transpose 2D Array(2D array=w1671) -> (transposed array=w1665:dbl[][])
                            n976 = local write "OMA V Hyperspectral graph"(w1665) -> ()
                          }
                        }
                        n977 = Not(x=w1645) -> (.not. x?=w1625:bool)
                        n978 = And(x=w1626, y=w1625) -> (x .and. y?=w1644:bool)
                      }
                      n979 = dll-call lib="C:/LabView_Projects/LifeEye/32bitDLLs/Madlib.dll" fn="MCL_SingleWriteN"("position"=w1601, "axis"=u32 2, "handle"=w1602) -> ()  [unwired: 6 in, 3 out]
                      n980 = And(x=w1599, y=w1606) -> (x .and. y?=w1607:bool)
                    }
                  }
                  frame "OMA V mode PLE map" {
                    n981 = local read "Steps LLTF"() -> (w1697:i32)
                    n982 = local read "LLTF error"() -> (w1705:errorcluster)
                    n983 = local read "End Wavelength LLTF"() -> (w1708:dbl)
                    n984 = local read "Start Wavelength LLTF"() -> (w1706:dbl)
                    n985 = Subtract(x=w1708, y=w1706) -> (x-y=w1707:dbl)
                    n986 = Subtract(x=w1697, y=1) -> (x-y=w1696:i32)
                    n987 = Divide(x=w1707, y=w1696) -> (x/y=w1709:dbl)
                    n988 = stacked-sequence {
                      seq-local: [w1722] -> [_]
                      tunnel: w1709 -> [w1713]
                      tunnel: w1706 -> [w1714]
                      tunnel: w1705 -> [w1725]
                      tunnel: w1697 -> [w1719]
                      tunnel: w1704 -> [w1721]
                      tunnel: [w1720] -> w1703
                      tunnel: w1702 -> [w1715]
                      tunnel: w1701 -> [w1712]
                      tunnel: w1700 -> [w1711]
                      tunnel: [w1710] -> w1699
                      frame #0 {
                        n989 = flat-sequence {
                          tunnel: w1725 -> [w1730]
                          tunnel: [w1729] -> w1726
                          tunnel: w1714 -> [w1728]
                          tunnel: [w1727] -> w1716
                          tunnel: w1715 -> [w1727]
                          tunnel: w1726 -> [w1748]
                          tunnel: [w1748] -> w1723
                          tunnel: w1719 -> [w1747]
                          tunnel: [w1744] -> w1718
                          tunnel: w1716 -> [w1741]
                          tunnel: w1714 -> [w1742]
                          tunnel: w1713 -> [w1737]
                          tunnel: [w1751] -> w1724
                          tunnel: w1723 -> [w1751]
                          tunnel: [w1749] -> w1717
                          tunnel: w1718 -> [w1749]
                          frame #0 {
                            n990 = local read "LLTF handle"() -> (w1731:u32)
                            n991 = call "PE Set Wavelength.vi"("error in (no error)"=w1730, "wavelength"=w1728, "peHandle"=w1731) -> ("error out"=w1729:errorcluster)  [unwired: 7 in, 1 out]
                          }
                          frame #1 {
                            n992 = Index Array(array=w1741, index=1023) -> (element=w1739:dbl)
                            n993 = Initialize Array(0.0 ("element"), w1747, 1024 ("dimension size")) -> (w1744:dbl[][])
                            n994 = property on="OMA V PLE map graph" class="IntGraph (strict)"("YScale.Offset"=w1742, "YScale.Multiplier"=w1737, "YScale.Precision"=u8 0 ("Y Scale.Display Format:Precision")) -> ()  [unwired: 2 in, 2 out]
                            n995 = Index Array(array=w1741, index=0) -> (element=w1738:dbl)
                            n996 = Subtract(x=w1739, y=w1738) -> (x-y=w1734:dbl)
                            n997 = Divide(x=w1734, y=1023.0) -> (x/y=w1732:dbl)
                            n998 = property on="OMA V PLE map graph" class="IntGraph (strict)"("XScale.Offset"=w1738, "XScale.Multiplier"=w1732, "XScale.Precision"=u8 0 ("X Scale.Display Format:Precision")) -> ()  [unwired: 2 in, 2 out]
                          }
                          frame #2 {
                            n999 = Wait (ms)(milliseconds to wait=1000.0 ("y")) -> ()  [unwired: 1 out]
                          }
                        }
                        n1000 = while {
                          tunnel: w1713 -> [w1773]
                          shift-right: [w1758] -> _
                          shift-left: w1714 -> [w1772]
                          tunnel: w1719 -> [w1752]
                          shift-right: [w1760] -> w1722
                          shift-left: w1724 -> [w1771]
                          tunnel: w1721 -> [w1753]
                          tunnel: [w1761] -> w1720
                          shift-right: [w1757] -> _
                          shift-left: w1717 -> [w1756]
                          tunnel: w1712 -> [w1755]
                          tunnel: w1711 -> [w1754]
                          tunnel: [w1753] -> w1710
                          i -> [w1759]
                          stop <- w1767 continue-if-true
                          n1001 = Decrement(x=w1752) -> ()  [unwired: 1 out]
                          n1002 = local read "LLTF handle"() -> (w1768:u32)
                          n1003 = Greater?(x=w1752, y=w1759) -> (0:w1764:bool)
                          n1004 = Add(x=w1772, y=w1773) -> (x+y=w1758:dbl)
                          n1005 = local read "Stop Measurement"() -> (w1766:bool)
                          n1006 = call "PE Set Wavelength.vi"("error in (no error)"=w1771, "wavelength"=w1772, "peHandle"=w1768) -> ("error out"=w1770:errorcluster)  [unwired: 7 in, 1 out]
                          n1007 = call "PE Get Wavelength.vi"("error in (no error)"=w1770, "peHandle"=w1768) -> ("error out"=w1762:errorcluster, "wavelength"=w1769:dbl)  [unwired: 7 in, 1 out]
                          n1008 = local write "Wavelength LLTF (nm)"(w1769) -> ()
                          n1009 = flat-sequence {
                            tunnel: w1764 -> [w1791]
                            tunnel: [w1791] -> w1763
                            tunnel: [w1790] -> w1760
                            tunnel: w1762 -> [w1790]
                            tunnel: w1753 -> [w1782]
                            tunnel: [w1781] -> w1761
                            tunnel: w1759 -> [w1775]
                            tunnel: w1756 -> [w1776]
                            tunnel: [w1777] -> w1757
                            tunnel: w1755 -> [w1780]
                            tunnel: w1754 -> [w1779]
                            frame #0 {
                              w1789 = 1  # Strip to pul out of frame
                              n1010 = call "CameraStart.vi"("error in"=w1780, "Camera Handle"=w1782) -> ("error out"=w1784:errorcluster, "Camera Handle"=w1783:u32)
                              n1011 = while {
                                tunnel: [w1798] -> w1788
                                tunnel: [w1799] -> w1787
                                tunnel: w1784 -> [w1793]
                                tunnel: w1783 -> [w1792]
                                stop <- w1795 stop-if-true
                                n1012 = call "CameraCheckData.vi"("Camera Handle"=w1792, "error in"=w1793) -> ("Camera Handle"=w1799:u32, "Number Of Frames Available"=w1800:i32, "error out"=w1798:errorcluster)
                                n1013 = Unbundle By Name(w1798) -> ("status"=w1797:bool)
                                n1014 = Greater Than 0?(x=w1800) -> (x > 0?=w1796:bool)
                                n1015 = Or(x=w1797, y=w1796) -> (x .or. y?=w1795:bool)
                                n1016 = Wait (ms)(milliseconds to wait=u32 5) -> ()  [unwired: 1 out]
                              }
                              n1017 = call "CameraGetData.vi"("error in"=w1788, "Data Handle"=w1779, "Camera Handle"=w1787) -> ("error out"=w1786:errorcluster, "Data Handle"=w1785:u32)  [unwired: 1 out]
                              n1018 = call "ImageGetLineF32.vi"("error in"=w1786, "Z Position"=w1789, "Y Position"=w1789, "Data Handle"=w1785) -> ("error out"=w1781:errorcluster, "Array F32"=w1774:sgl[])  [unwired: 1 out]
                              n1019 = Replace Array Subset(array=w1776, new element=w1774, index (row)=w1775) -> (w1777:dbl[][])  [unwired: 1 in]
                              n1020 = Transpose 2D Array(2D array=w1777) -> (transposed array=→"OMA V PLE map graph":dbl[][])
                            }
                          }
                          n1021 = Not(x=w1766) -> (.not. x?=w1765:bool)
                          n1022 = And(x=w1763, y=w1765) -> (x .and. y?=w1767:bool)
                        }
                      }
                    }
                  }
                  frame "OMA V mode PL external sync" {
                    n1023 = Index Array(array=w1805, index=1) -> (element=w1809:dbl)
                    n1024 = Index Array(array=w1805, index=0) -> (element=w1807:dbl)
                    n1025 = Index Array(array=w1805, index=1023) -> (element=w1818:dbl)
                    n1026 = property on="OMA V PL external  sync plot" class="IntGraph (strict)"("YScale.Offset"=0.0 ("Y Scale.Offset and Multiplier:Offset"), "YScale.Multiplier"=1.0 ("Y Scale.Offset and Multiplier:Multiplier"), "YScale.Precision"=u8 0 ("Y Scale.Display Format:Precision")) -> ()  [unwired: 2 in, 2 out]
                    n1027 = Subtract(x=w1809, y=w1807) -> (x-y=w1808:dbl)
                    n1028 = Subtract(x=w1807, y=w1808) -> (x-y=w1806:dbl)
                    n1029 = Subtract(x=w1818, y=w1807) -> (x-y=w1815:dbl)
                    n1030 = Divide(x=w1815, y=1023.0) -> (x/y=w1813:dbl)
                    n1031 = Initialize Array(0.0 ("element"), 1 ("dimension size"), 1024 ("dimension size")) -> (w1804:dbl[][])
                    n1032 = property on="OMA V PL external  sync plot" class="IntGraph (strict)"("XScale.Offset"=w1806, "XScale.Multiplier"=w1813, "XScale.Precision"=u8 1 ("X Scale.Display Format:Precision")) -> ()  [unwired: 2 in, 2 out]
                    n1033 = while {
                      tunnel: w1825 -> [w1838]
                      tunnel: w1824 -> [w1831]
                      tunnel: w1801 -> [w1837]
                      tunnel: [w1836] -> w1823
                      tunnel: [w1835] -> w1822
                      shift-right: [w1833] -> _
                      shift-left: w1804 -> [w1832]
                      i -> [w1829]
                      stop <- w1828 stop-if-true
                      n1034 = flat-sequence {
                        tunnel: w1837 -> [w1840]
                        tunnel: [w1840] -> w1827
                        tunnel: w1827 -> [w1842]
                        tunnel: [w1842] -> w1826
                        tunnel: [w1844] -> w1830
                        tunnel: [w1843] -> w1828
                        tunnel: w1826 -> [w1845]
                        frame #0 {
                          w1839 = TRUE ("OMAV ready for sync")
                          n1035 = local write "OMA V ready for sync"(w1839) -> ()
                          n1036 = global write "sync_global.vi" "OMAV ready for sync"(w1839) -> ()
                        }
                        frame #1 {
                          n1037 = Wait (ms)(milliseconds to wait=u32 200) -> ()  [unwired: 1 out]
                        }
                        frame #2 {
                          n1038 = while {
                            tunnel: w1845 -> [w1850]
                            tunnel: [w1850] -> w1844
                            tunnel: [w1847] -> w1843
                            stop <- w1849 stop-if-true
                            n1039 = local read "Stop Measurement"() -> (w1847:bool)
                            n1040 = global read "sync_global.vi" "sync"() -> (w1846:bool)
                            n1041 = local write "OMAV external sync"(w1846) -> ()
                            n1042 = Or(x=w1847, y=w1846) -> (x .or. y?=w1849:bool)
                            n1043 = Wait (ms)(milliseconds to wait=u32 50) -> ()  [unwired: 1 out]
                          }
                        }
                      }
                      n1044 = case shown="False" w1828 {
                        tunnel: w1838 -> [w1875 _]
                        tunnel: [w1874 w1924] -> w1836
                        tunnel: [w1873 w1925] -> w1835
                        tunnel: [w1863 w1922] -> w1834
                        tunnel: [w1862 w1923] -> w1833
                        tunnel: w1832 -> [w1864 w1923]
                        tunnel: w1831 -> [w1872 w1924]
                        tunnel: w1830 -> [w1871 w1925]
                        tunnel: w1829 -> [w1868 _]
                        frame False {
                          w1880 = 1  # Strip to pul out of frame
                          n1045 = flat-sequence {
                            tunnel: w1872 -> [w1898]
                            tunnel: [w1898] -> w1861
                            tunnel: w1871 -> [w1897]
                            tunnel: [w1897] -> w1860
                            tunnel: w1861 -> [w1901]
                            tunnel: [w1901] -> w1857
                            tunnel: w1860 -> [w1900]
                            tunnel: [w1900] -> w1855
                            tunnel: w1857 -> [w1904]
                            tunnel: [w1904] -> w1856
                            tunnel: w1855 -> [w1903]
                            tunnel: [w1903] -> w1854
                            tunnel: w1856 -> [w1908]
                            tunnel: w1854 -> [w1907]
                            tunnel: [w1906] -> w1859
                            tunnel: [w1905] -> w1858
                            tunnel: [w1910] -> w1869
                            tunnel: [w1911] -> w1870
                            tunnel: w1859 -> [w1911]
                            tunnel: w1858 -> [w1910]
                            frame #0 {
                              w1896 = FALSE ("OMAV ready for sync")
                              n1046 = global write "sync_global.vi" "OMAV ready for sync"(w1896) -> ()
                              n1047 = local write "OMA V ready for sync"(w1896) -> ()
                              n1048 = local write "OMAV external sync"(w1896) -> ()
                              n1049 = global write "sync_global.vi" "sync"(w1896) -> ()
                            }
                            frame #1 {
                              n1050 = Wait (ms)(milliseconds to wait=u32 200) -> ()  [unwired: 1 out]
                            }
                            frame #2 {
                              n1051 = local write "OMA V acquire from external"(TRUE ("OMA V acquire from external")) -> ()
                            }
                            frame #3 {
                              n1052 = call "CameraStart.vi"("error in"=w1907, "Camera Handle"=w1908) -> ("error out"=w1905:errorcluster, "Camera Handle"=w1906:u32)
                            }
                            frame #4 {
                              n1053 = global read "sync_global.vi" "sync"() -> (w1909:bool)
                              n1054 = local write "OMAV external sync"(w1909) -> ()
                            }
                          }
                          n1055 = while {
                            tunnel: [w1918] -> w1879
                            tunnel: [w1919] -> w1878
                            tunnel: w1869 -> [w1913]
                            tunnel: w1870 -> [w1912]
                            stop <- w1915 stop-if-true
                            n1056 = call "CameraCheckData.vi"("Camera Handle"=w1912, "error in"=w1913) -> ("Camera Handle"=w1919:u32, "Number Of Frames Available"=w1920:i32, "error out"=w1918:errorcluster)
                            n1057 = Unbundle By Name(w1918) -> ("status"=w1917:bool)
                            n1058 = Greater Than 0?(x=w1920) -> (x > 0?=w1916:bool)
                            n1059 = Or(x=w1917, y=w1916) -> (x .or. y?=w1915:bool)
                            n1060 = Wait (ms)(milliseconds to wait=u32 5) -> ()  [unwired: 1 out]
                          }
                          n1061 = Equal?(x=w1868, y=0) -> (x = y?=w1866:bool)
                          n1062 = call "CameraGetData.vi"("error in"=w1879, "Data Handle"=w1875, "Camera Handle"=w1878) -> ("error out"=w1877:errorcluster, "Data Handle"=w1876:u32, "Camera Handle"=w1874:u32)
                          n1063 = call "ImageGetLineF32.vi"("error in"=w1877, "Z Position"=w1880, "Y Position"=w1880, "Data Handle"=w1876) -> ("error out"=w1873:errorcluster, "Array F32"=w1865:sgl[])  [unwired: 1 out]
                          n1064 = flat-sequence {
                            tunnel: w1864 -> [w1882]
                            tunnel: w1865 -> [w1883]
                            tunnel: w1866 -> [w1884]
                            tunnel: [w1884] -> w1853
                            tunnel: [w1883] -> w1852
                            tunnel: [w1882] -> w1851
                            tunnel: [w1885] -> w1862
                            tunnel: w1853 -> [w1888]
                            tunnel: w1852 -> [w1887]
                            tunnel: w1851 -> [w1886]
                            frame #0 {
                              n1065 = local write "OMA V acquire from external"(FALSE ("OMA V acquire from external")) -> ()
                            }
                            frame #1 {
                              n1066 = case shown="True" w1888 {
                                tunnel: w1887 -> [w1891 w1893]
                                tunnel: w1886 -> [w1890 w1894]
                                tunnel: [w1889 w1892] -> w1885
                                frame False {
                                n1067 = Build Array (concatenate)(w1890, w1891) -> (w1889:dbl[][])
                                }
                                frame True {
                                n1068 = Replace Array Subset(array=w1894, new element=w1893, index (row)=0) -> (w1892:dbl[][])  [unwired: 1 in]
                                }
                              }
                            }
                          }
                          n1069 = Transpose 2D Array(2D array=w1862) -> (transposed array=w1863:dbl[][])
                        }
                        frame True {
                          w1921 = FALSE ("OMAV ready for sync")
                          n1070 = global write "sync_global.vi" "OMAV ready for sync"(w1921) -> ()
                          n1071 = local write "OMA V ready for sync"(w1921) -> ()
                          n1072 = Transpose 2D Array(2D array=w1923) -> (transposed array=w1922:dbl[][])
                        }
                      }
                      "OMA V PL external  sync plot" <- w1834
                    }
                  }
                }
                n1073 = call "ToolKitIsError.vi"("error in"=w1411) -> ("error out"=w1412:errorcluster, "Error Flag"=w1405:bool)  [unwired: 1 in]
                n1074 = case shown="True" w1405 {
                  tunnel: w1412 -> [w1926 w1930]
                  tunnel: [w1926 w1928] -> w1403
                  frame False {
                  }
                  frame True {
                    w1927 = u16 1 items=["no dialog", "OK message", "continue or stop message"] ("type of dialog (OK msg:1)")
                    n1075 = call <vilib>:"Simple Error Handler.vi"("type of dialog (OK msg:1)"=w1927, "error in (no error)"=w1930) -> ("error?"=w1929:bool, "error out"=w1928:errorcluster)  [unwired: 3 in, 3 out]
                    n1076 = Stop(stop? (T)=w1929) -> ()
                  }
                }
                n1077 = local write "MonoError"(w1403) -> ()
                n1078 = call "CameraStop.vi"("error in"=w1391, "Camera Handle"=w1389) -> ("error out"=w1388:errorcluster)  [unwired: 1 out]
                n1079 = local write "OMA V error"(w1388) -> ()
              }
              frame #1 {
              }
            }
          }
          frame 32 {
            # "OMA V start background"
            n1080 = flat-sequence {
              frame #0 {
                w1955 = u32 1 ("Turret Number")
                n1081 = local read "MonoError"() -> (w1968:errorcluster)
                n1082 = local read "Wavelength (nm)"() -> (w1967:dbl)
                n1083 = local read "Grating Number"() -> (w1956:i16)
                n1084 = local read "Mono Calibration Handle"() -> (w1966:u32)
                n1085 = case shown="1, Default" w1956 {
                  tunnel: [w1969 w1977 w1985] -> w1965
                  frame 1, Default {
                    w1970 = 25.0  # Pixel Width (microns)
                    w1971 = 1.0  # Magnification
                    w1972 = 1.35  # Detector Angle (degrees)
                    w1973 = 30.3  # Inclusion Angle (degrees)
                    w1974 = 300.0  # Focal Length (mm)
                    w1975 = 0.0  # Slope Adjust
                    w1976 = -3.71785  # Center Offset
                    n1086 = Bundle("Center Offset"=w1976, "Slope Adjust"=w1975, "Focal Length (mm)"=w1974, "Inclusion Angle (degrees)"=w1973, "Detector Angle (degrees)"=w1972, "Magnification"=w1971, "Pixel Width (microns)"=w1970) -> (w1969:T6)  [unwired: 1 in]
                  }
                  frame 2 {
                    w1978 = 25.0  # Pixel Width (microns)
                    w1979 = 1.0  # Magnification
                    w1980 = -2.77  # Detector Angle (degrees)
                    w1981 = 32.7  # Inclusion Angle (degrees)
                    w1982 = 295.6  # Focal Length (mm)
                    w1983 = -0.000221379  # Slope Adjust
                    w1984 = -0.047502  # Center Offset
                    n1087 = Bundle("Center Offset"=w1984, "Slope Adjust"=w1983, "Focal Length (mm)"=w1982, "Inclusion Angle (degrees)"=w1981, "Detector Angle (degrees)"=w1980, "Magnification"=w1979, "Pixel Width (microns)"=w1978) -> (w1977:T6)  [unwired: 1 in]
                  }
                  frame 3 {
                    w1986 = 25.0  # Pixel Width (microns)
                    w1987 = 1.0  # Magnification
                    w1988 = -2.77  # Detector Angle (degrees)
                    w1989 = 31.85  # Inclusion Angle (degrees)
                    w1990 = 297.6  # Focal Length (mm)
                    w1991 = 0.000251338  # Slope Adjust
                    w1992 = -1.24655  # Center Offset
                    n1088 = Bundle("Center Offset"=w1992, "Slope Adjust"=w1991, "Focal Length (mm)"=w1990, "Inclusion Angle (degrees)"=w1989, "Detector Angle (degrees)"=w1988, "Magnification"=w1987, "Pixel Width (microns)"=w1986) -> (w1985:T6)  [unwired: 1 in]
                  }
                }
                n1089 = call "CalibSetAdjVals.vi"("Calibration Handle"=w1966, "Turret Number"=w1955, "Grating Number"=w1956, "error in"=w1968, "Spectrometer Calibration Parameters"=w1965) -> ("Calibration Handle"=w1963:u32, "error out"=w1964:errorcluster)
                n1090 = call "CalibSetSpectInfo.vi"("Calibration Handle"=w1963, "Current Grating Number"=w1956, "Current Wavelength"=w1967, "error in"=w1964, "Current Turret Number"=w1955) -> ("Calibration Handle"=w1961:u32, "error out"=w1960:errorcluster)
                n1091 = call "CalibGetCalibArray.vi"("error in"=w1960, "Array Size"=u32 1024, "Calibration Handle"=w1961) -> ("error out"=w1959:errorcluster, "Calibrated Array"=w1958:dbl[])  [unwired: 1 out]
                n1092 = local write "OMA V Calibrated Array"(w1958) -> ()
                n1093 = call "ToolKitIsError.vi"("error in"=w1959) -> ("error out"=w1957:errorcluster)  [unwired: 1 in, 1 out]
                n1094 = local write "MonoError"(w1957) -> ()
              }
              frame #1 {
                w2013 = 1  # Strip to pul out of frame
                n1095 = local read "OMA V error"() -> (w1997:errorcluster)
                n1096 = local read "OMA V exposure time"() -> (w1995:dbl)
                n1097 = local read "OMA V Handles Out"() -> (w2014:T5)
                n1098 = local read "OMA V Calibrated Array"() -> (w2005:dbl[])
                n1099 = Unbundle(w2014) -> ("Camera Handle"=w1998:u32, "Image Handle"=w1993:u32)  [unwired: 3 out]
                n1100 = call "CameraExperiment.vi"("Number of Accumulations"=u32 1, "Acquire / Focus Flag"=u32 1, "error in"=w1997, "Number of Images"=u32 1, "Exposure (sec)"=w1995, "Camera Handle"=w1998) -> ("error out"=w1996:errorcluster)  [unwired: 1 out]
                n1101 = call "CameraOnlineBackSubSetup.vi"("error in"=w1996, "Background Flag"=u32 0, "Background Image Handle"=w1993, "Camera Handle"=w1998) -> ("error out"=w2016:errorcluster, "Camera Handle"=w2017:u32)  [unwired: 1 out]
                n1102 = call "CameraStart.vi"("error in"=w2016, "Camera Handle"=w2017) -> ("error out"=w2015:errorcluster, "Camera Handle"=w2007:u32)
                n1103 = while {
                  tunnel: w2007 -> [w2027]
                  tunnel: [w2024] -> _
                  tunnel: [w2025] -> w2008
                  tunnel: w2015 -> [w2019]
                  stop <- w2021 stop-if-true
                  n1104 = call "CameraCheckData.vi"("Camera Handle"=w2027, "error in"=w2019) -> ("Camera Handle"=w2025:u32, "Number Of Frames Available"=w2026:i32, "error out"=w2024:errorcluster)
                  n1105 = Unbundle By Name(w2024) -> ("status"=w2023:bool)
                  n1106 = Greater Than 0?(x=w2026) -> (x > 0?=w2022:bool)
                  n1107 = Or(x=w2023, y=w2022) -> (x .or. y?=w2021:bool)
                  n1108 = Wait (ms)(milliseconds to wait=u32 5) -> ()  [unwired: 1 out]
                }
                n1109 = call "CameraGetData.vi"("Data Handle"=w1993, "Camera Handle"=w2008) -> ("error out"=w2011:errorcluster, "Data Handle"=w2012:u32, "Camera Handle"=w1994:u32)  [unwired: 1 in]
                n1110 = call "ImageGetLineF32.vi"("error in"=w2011, "Z Position"=w2013, "Y Position"=w2013, "Data Handle"=w2012) -> ("error out"=w2010:errorcluster, "Array F32"=w2006:sgl[])  [unwired: 1 out]
                n1111 = Bundle("OMA V Calibrated Array"=w2005, "Array F32"=w2006) -> (w2004:T10)  [unwired: 1 in]
                n1112 = local write "XY Graph OMA V"(w2004) -> ()
                n1113 = call "CameraOnlineBackSubSetup.vi"("error in"=w2010, "Background Flag"=1 ("Background Flag\n1-enable"), "Background Image Handle"=w1993, "Camera Handle"=w1994) -> ("error out"=w2009:errorcluster)  [unwired: 2 out]
                n1114 = call "CameraStop.vi"("error in"=w2009, "Camera Handle"=w1994) -> ("error out"=w2003:errorcluster)  [unwired: 1 out]
                n1115 = local write "OMA V error"(w2003) -> ()
              }
              frame #2 {
                n1116 = local write "OMA V correct background"(TRUE ("OMA V correct background")) -> ()
              }
            }
          }
          frame 33 {
            # "OMA V start focus"
            n1117 = flat-sequence {
              frame #0 {
                w2030 = u32 1 ("Turret Number")
                n1118 = local read "MonoError"() -> (w2033:errorcluster)
                n1119 = local read "Wavelength (nm)"() -> (w2034:dbl)
                n1120 = local read "Grating Number"() -> (w2029:i16)
                n1121 = local read "Mono Calibration Handle"() -> (w2032:u32)
                n1122 = case shown="2" w2029 {
                  tunnel: [w2043 w2051 w2059] -> w2031
                  frame 1, Default {
                    w2044 = 25.0  # Pixel Width (microns)
                    w2045 = 1.0  # Magnification
                    w2046 = 1.35  # Detector Angle (degrees)
                    w2047 = 30.3  # Inclusion Angle (degrees)
                    w2048 = 300.0  # Focal Length (mm)
                    w2049 = 0.0  # Slope Adjust
                    w2050 = -3.71785  # Center Offset
                    n1123 = Bundle("Center Offset"=w2050, "Slope Adjust"=w2049, "Focal Length (mm)"=w2048, "Inclusion Angle (degrees)"=w2047, "Detector Angle (degrees)"=w2046, "Magnification"=w2045, "Pixel Width (microns)"=w2044) -> (w2043:T6)  [unwired: 1 in]
                  }
                  frame 2 {
                    w2052 = 25.0  # Pixel Width (microns)
                    w2053 = 1.0  # Magnification
                    w2054 = -2.77  # Detector Angle (degrees)
                    w2055 = 32.7  # Inclusion Angle (degrees)
                    w2056 = 295.6  # Focal Length (mm)
                    w2057 = -0.000221379  # Slope Adjust
                    w2058 = -0.047502  # Center Offset
                    n1124 = Bundle("Center Offset"=w2058, "Slope Adjust"=w2057, "Focal Length (mm)"=w2056, "Inclusion Angle (degrees)"=w2055, "Detector Angle (degrees)"=w2054, "Magnification"=w2053, "Pixel Width (microns)"=w2052) -> (w2051:T6)  [unwired: 1 in]
                  }
                  frame 3 {
                    w2060 = 25.0  # Pixel Width (microns)
                    w2061 = 1.0  # Magnification
                    w2062 = -2.77  # Detector Angle (degrees)
                    w2063 = 31.85  # Inclusion Angle (degrees)
                    w2064 = 297.6  # Focal Length (mm)
                    w2065 = 0.000251338  # Slope Adjust
                    w2066 = -1.24655  # Center Offset
                    n1125 = Bundle("Center Offset"=w2066, "Slope Adjust"=w2065, "Focal Length (mm)"=w2064, "Inclusion Angle (degrees)"=w2063, "Detector Angle (degrees)"=w2062, "Magnification"=w2061, "Pixel Width (microns)"=w2060) -> (w2059:T6)  [unwired: 1 in]
                  }
                }
                n1126 = call "CalibSetAdjVals.vi"("Calibration Handle"=w2032, "Turret Number"=w2030, "Grating Number"=w2029, "error in"=w2033, "Spectrometer Calibration Parameters"=w2031) -> ("Calibration Handle"=w2041:u32, "error out"=w2042:errorcluster)
                n1127 = call "CalibSetSpectInfo.vi"("Calibration Handle"=w2041, "Current Grating Number"=w2029, "Current Wavelength"=w2034, "error in"=w2042, "Current Turret Number"=w2030) -> ("Calibration Handle"=w2039:u32, "error out"=w2038:errorcluster)
                n1128 = call "CalibGetCalibArray.vi"("error in"=w2038, "Array Size"=u32 1024, "Calibration Handle"=w2039) -> ("error out"=w2037:errorcluster, "Calibrated Array"=w2036:dbl[])  [unwired: 1 out]
                n1129 = local write "OMA V Calibrated Array"(w2036) -> ()
                n1130 = call "ToolKitIsError.vi"("error in"=w2037) -> ("error out"=w2035:errorcluster)  [unwired: 1 in, 1 out]
                n1131 = local write "MonoError"(w2035) -> ()
              }
              frame #1 {
                n1132 = local read "OMA V error"() -> (w2076:errorcluster)
                n1133 = local read "OMA V exposure time"() -> (w2075:dbl)
                n1134 = local read "OMA V Handles Out"() -> (w2077:T5)
                n1135 = Unbundle(w2077) -> ("Camera Handle"=w2068:u32, "Image Handle"=w2070:u32)  [unwired: 3 out]
                n1136 = call "CameraExperiment.vi"("Number of Accumulations"=u32 1, "Acquire / Focus Flag"=u32 1, "error in"=w2076, "Number of Images"=u32 1, "Exposure (sec)"=w2075, "Camera Handle"=w2068) -> ("error out"=w2073:errorcluster, "Camera Handle"=w2074:u32)
                n1137 = call "CameraStart.vi"("error in"=w2073, "Camera Handle"=w2074) -> ("error out"=w2071:errorcluster, "Camera Handle"=w2072:u32)
                n1138 = while {
                  tunnel: w2072 -> [w2092]
                  tunnel: w2071 -> [w2091]
                  tunnel: w2070 -> [w2082]
                  tunnel: [w2081] -> w2069
                  stop <- w2085 stop-if-true
                  n1139 = call "CameraCheckData.vi"("Camera Handle"=w2092, "error in"=w2091) -> ("Camera Handle"=w2084:u32, "Number Of Frames Available"=w2090:i32, "error out"=w2083:errorcluster)
                  n1140 = Greater Than 0?(x=w2090) -> (x > 0?=w2089:bool)
                  n1141 = local read "OMA V exposure time"() -> (w2086:dbl)
                  n1142 = case shown="True" w2089 {
                    tunnel: [FALSE ("Stop Measurement") w2106] -> w2085
                    tunnel: w2084 -> [_ w2097]
                    tunnel: w2083 -> [w2094 w2098]
                    tunnel: w2082 -> [_ w2099]
                    tunnel: [w2094 w2096] -> w2081
                    frame False {
                    }
                    frame True {
                      w2105 = 1 ("Strip to pul out of frame")
                      n1143 = call "CameraGetData.vi"("error in"=w2098, "Data Handle"=w2099, "Camera Handle"=w2097) -> ("error out"=w2103:errorcluster, "Data Handle"=w2104:u32)  [unwired: 1 out]
                      n1144 = local read "Stop Measurement"() -> (w2106:bool)
                      n1145 = local read "OMA V Calibrated Array"() -> (w2101:dbl[])
                      n1146 = call "ImageGetLineF32.vi"("error in"=w2103, "Z Position"=w2105, "Y Position"=w2105, "Data Handle"=w2104) -> ("error out"=w2096:errorcluster, "Array F32"=w2102:sgl[])  [unwired: 1 out]
                      n1147 = Bundle("OMA V Calibrated Array"=w2101, "Array F32"=w2102) -> (w2100:T10)  [unwired: 1 in]
                      n1148 = local write "XY Graph OMA V"(w2100) -> ()
                    }
                  }
                  n1149 = Less?(x=w2086, y=0.01) -> (x < y?=w2088:bool)
                  n1150 = case shown="True" w2088 {
                    frame False {
                    }
                    frame True {
                      n1151 = Wait (ms)(milliseconds to wait=u32 10) -> ()  [unwired: 1 out]
                    }
                  }
                }
                n1152 = call "CameraStop.vi"("error in"=w2069, "Camera Handle"=w2068) -> ("error out"=w2067:errorcluster)  [unwired: 1 out]
                n1153 = local write "OMA V error"(w2067) -> ()
              }
              frame #2 {
              }
            }
          }
        }
      }
      frame #2 {
        w2108 = FALSE ("Busy")
        n1154 = local read "PicoHarp ON"() -> (w2110:bool)
        n1155 = local read "LockIn ON"() -> (w2107:bool)
        n1156 = local write "Busy"(w2108) -> ()
        n1157 = case shown="False" FALSE {
          frame False {
          }
          frame True {
            n1158 = local read "Mono handle"() -> (w2132:u32)
            n1159 = local read "MonoError"() -> (w2131:errorcluster)
            n1160 = call "SpectGetSlitInfo.vi"("Spectrometer Handle"=w2132, "Slit"=i16 2, "error in"=w2131) -> ("Spectrometer Handle"=w2127:u32, "Position"=w2129:dbl, "error out"=w2126:errorcluster)  [unwired: 1 out]
            n1161 = local write "Input Slit (µm)"(w2129) -> ()
            n1162 = call "SpectGetSlitInfo.vi"("Spectrometer Handle"=w2127, "Slit"=i16 4, "error in"=w2126) -> ("Spectrometer Handle"=w2121:u32, "Position"=w2128:dbl, "error out"=w2120:errorcluster)  [unwired: 1 out]
            n1163 = local write "Output Slit (µm)"(w2128) -> ()
            n1164 = call "SpectGetGratingInfo.vi"("Spectrometer Handle"=w2121, "error in"=w2120) -> ("Current Wavelength"=w2124:dbl, "Spectrometer Handle"=w2123:u32, "Current Grating"=w2119:i16, "error out"=w2122:errorcluster)  [unwired: 2 out]
            n1165 = local write "Wavelength (nm)"(w2124) -> ()
            n1166 = local write "Mono handle"(w2123) -> ()
            n1167 = local write "Grating Number"(w2119) -> ()
            n1168 = local write "MonoError"(w2122) -> ()
          }
        }
        n1169 = local read "PiezoStage ON"() -> (w2111:bool)
        n1170 = case shown="True" w2110 {
          frame False {
          }
          frame True {
          }
        }
        n1171 = case shown="True" w2107 {
          frame False {
          }
          frame True {
          }
        }
        n1172 = local write "Stop Measurement"(w2108) -> ()
        n1173 = case shown="False" w2111 {
          frame False {
          }
          frame True {
            w2115 = FALSE ("commandZ")
            n1174 = local read "Piezohandle"() -> (w2113:i32)
            n1175 = call "_subvi_LivePos_Main.vi"("handle"=w2113, "counter"=u32 50, "commandZ"=w2115, "commandY"=w2115, "commandX"=w2115) -> ("xRead"=w2118:dbl, "yRead"=w2117:dbl, "zRead"=w2116:dbl)  [unwired: 3 in, 9 out]
            n1176 = local write "xRead"(w2118) -> ()
            n1177 = local write "yRead"(w2117) -> ()
            n1178 = local write "zRead"(w2116) -> ()
          }
        }
      }
    }
  }
  n1179 = local write "OMA V temp"(0.0 ("OMA V temp")) -> ()
  n1180 = local write "Wavelength (nm)"(0.0 ("Wavelength (nm)")) -> ()
  n1181 = local write "OMA V correct background"(w8) -> ()
  n1182 = local write "OMA V set temp"(i8 -100 ("OMA V set temp")) -> ()
  n1183 = local write "Filter Wheel Position"(w15) -> ()
  n1184 = local write "Grating Number"(w14) -> ()
  n1185 = property on="OMA V mode Hyperspectral" class="Bool (strict)"("DisabledEnum"=w4) -> ()  [unwired: 2 in, 2 out]
  n1186 = property on="OMA V mode PLE map" class="Bool (strict)"("DisabledEnum"=w4) -> ()  [unwired: 2 in, 2 out]
  n1187 = property on="OMA V mode Hyperspectral 2D" class="Bool (strict)"("DisabledEnum"=w4) -> ()  [unwired: 2 in, 2 out]
  n1188 = local write "OMA V aquire mode"(T4."OMA V mode Single spectrum" ("OMA V aquire mode")) -> ()
  n1189 = local write "Configuration File"(path "C:/LabView_Projects/LifeEye/system.xml" ("Configuration File")) -> ()
  "Mono ON" <- w8
  "PicoHarp ON" <- w8
  "PiezoStage ON" <- w8
  "Busy" <- FALSE ("Busy")
  "MonoError" <- errorcluster {"status"=FALSE, "code"=0, "source"=""} ("error out")
  "Piezohandle" <- 0 ("handle")
  "PicoHarpHandle" <- 0
  "PicoHarpInitError" <- w17
  "Error" <- w17
  "Resolution" <- 0
  "LockIn ON" <- w8
  "LLTF ON" <- w8
  "LLTF handle" <- u32 0 ("LLTF handle")
  "timestart" <- 0.0 ("timestart")
  "timeend" <- 0.0 ("timeend")
  "Real Delay (seconds/step)" <- 0.0 ("Speed(nm/s)")
  "OMA  V ON" <- w8
  "OMAV external sync" <- FALSE ("OMAV external triggered")
  "OMA V ready for sync" <- FALSE ("OMA V ready for sync")
  "OMA V acquire from external" <- FALSE ("OMA V acquire from external")
